vi "WorkingWithoutCheck-MatlabImageProcessing-red_tweezers_interface_linegen - test_edited for seq order - Copy - Copy - Copy.vi"() -> ()   [LabVIEW 2015]
doc: "This is the interface, the one VI which loads all the others. Run this one first.\n\n(the line below ensures settings are saved)\n[Red Tweezers Save Settings]"
uses:
  subvis/line_trapping.ctl
  subvis/spot.ctl
  <vilib>/userdefined/High Color/IMAQdx.ctl
  subvis/selection_element.ctl
  subvis/mouse_info.ctl
  <vilib>/Analysis/baseanly.llb/Real A x B.vi
  subvis/red_tweezers_globals_INTERNAL_VOLATILE.vi
  subvis/red_tweezers_globals.vi
  <vilib>/Analysis/NI_AALBase.lvlib
  <vilib>/vision/driver/NI_Vision_Acquisition_Software.lvlib
panel:
  out "Spot Storage":T1[](array[typedef]) {"Amplitude Correction" step=0.1; "Line Trapping"."Phase Gradient" step=0.05; "Line Trapping"."Vector"."x" step=1e-06 format="%#_6p"; "Line Trapping"."Vector"."y" step=1e-06 format="%#_6p"; "Line Trapping"."Vector"."z" step=1e-06 format="%#_6p"; "NA Position"."r" step=1e-06; "NA Position"."y" step=1e-06; "NA Position"."x" step=1e-06; "Position"."z" step=1e-06; "Position"."y" step=1e-06; "Position"."x" step=1e-06; "Phase" step=0.7753; "Intensity" step=0.1}
  out "# selected":i16
  out "Last Pattern":T1[](array[typedef]) {"Amplitude Correction" step=0.1; "Line Trapping"."Phase Gradient" step=0.05; "Line Trapping"."Vector"."x" step=1e-06 format="%#_6p"; "Line Trapping"."Vector"."y" step=1e-06 format="%#_6p"; "Line Trapping"."Vector"."z" step=1e-06 format="%#_6p"; "NA Position"."r" step=1e-06; "NA Position"."y" step=1e-06; "NA Position"."x" step=1e-06; "Position"."z" step=1e-06; "Position"."y" step=1e-06; "Position"."x" step=1e-06; "Phase" step=0.7753; "Intensity" step=0.1}
  out "Plugins":T3(array[cluster])=[{"Name"="ASI Stage", "Folder"=path "C:/Users/Richard Bowman/Dropbox/red_tweezers_1_4_rc4/plugins/ASI Stage.llb", "vi reference"=refnum, "Needs to be run"=TRUE, "Error"={"status"=FALSE, "code"=0, "source"=""}}, {"Name"="iTweezers", "Folder"=path "C:/Users/Richard Bowman/Dropbox/red_tweezers_1_4_rc4/plugins/iTweezers.llb", "vi reference"=refnum, "Needs to be run"=TRUE, "Error"={"status"=FALSE, "code"=0, "source"=""}}, {"Name"="MightexLED", "Folder"=path "C:/Users/Richard Bowman/Dropbox/red_tweezers_1_4_rc4/plugins/MightexLED.llb", "vi reference"=refnum, "Needs to be run"=TRUE, "Error"={"status"=FALSE, "code"=0, "source"=""}}]
  in  "Tab":T4(tab)
  out "Play Pressed":bool
  out "Y":dbl
  out "X":dbl
  in  "O Button":bool
  in  "OK Button":bool
  in  "Bubble Size":dbl=50.0002
  out "Hit Indicator":bool
  in  "On":bool
  out "Induce check":bool
  out "Area+ Buffer":dbl
  in  "Area to check":dbl=0.00025
  out "Prev Current Spot":dbl
  out "spots selected 2":i32=4
  out "Spot # Check":dbl
  out "Orig Y SC":dbl
  out "Orig X SC":dbl
  out "ID num check":dbl
  out "Value Check":dbl
  out "ID":dbl[](array[numeric])
  out "Null array":dbl[](array[numeric])
  out "Potential Collisions":dbl
  out "What to Check":dbl[](array[numeric])
  out "Num":dbl
  out "Old Y":dbl
  out "Old X":dbl
  out "init":dbl
  out "Looper":bool
  in  "Output to SLM":bool
  out "Maximum":dbl
  out "Projected Distance":dbl
  out "Previous Distance":dbl
  out "Group ID #":dbl
  in  "Buffer Zone":dbl=7e-05
  out "# of Spots":dbl
  out "Distance":dbl
  out "Hit":bool
  out "Y Displacement":dbl
  out "X Displacement":dbl
  out "Current Spot #":dbl
  out "spots selected":i32=4
  in  "lock aspect ratio":bool=TRUE
  in  "Size":cluster{"x":dbl, "y":dbl, "z":dbl} {"z" step=1e-06 format="%#_4p"; "y" step=1e-06 format="%#_4p"; "x" step=1e-06 format="%#_4p"}
  in  "Position":cluster{"x":dbl, "y":dbl, "z":dbl}={"x"=1e-06, "y"=-6.3e-06, "z"=0.0} {"z" step=1e-06 format="%#_4p"; "y" step=1e-06 format="%#_4p"; "x" step=1e-06 format="%#_4p"}
  in  "phase":dbl step=0.7753
  in  "Vortex Charge":i8
  in  "Intensity":dbl=1.0 step=0.1
  in  "add to selection":bool
  in  "random position":bool
  in  "new spot":bool
  in  "delete":bool
  in  "rotate":bool
  in  "Rotation Axis":u16(ring)=2 items=["Z", "X", "Y", "Custom"]
  in  "Angle (degrees)":dbl=2.0
  in  "Custom Axis":cluster{dbl, dbl, dbl}
  in  "Spot Shape":enum32{"Normal", "Line", "NA", "Mixed"}(tab)=enum."Mixed"
  in  "Line Trapping":T2 {"Phase Gradient" step=0.05; "Vector"."x" step=1e-06 format="%#_4p"; "Vector"."y" step=1e-06 format="%#_4p"; "Vector"."z" step=1e-06 format="%#_4p"}
  in  "Scale back aperture":dbl=1.1 step=0.1
  in  "Scale BA":bool
  in  "Position on back aperture":cluster{"x":dbl, "y":dbl}={"x"=-5.84327907697451e-18, "y"=0.0} {"y" step=0.1 format="%#_4p"; "x" step=0.1 format="%#_4p"}
  in  "Radius on back aperture":dbl=1.1 step=0.1
  in  "Generate":bool
  in  "Pattern":T5(tab)
  in  "Spots across centre":i32=5
  in  "Reference Array?":bool
  in  "Fraction of SLM":dbl=1.0
  in  "Spots across centre":i32=5
  in  "N":cluster{i32, i32}
  in  "spacing/m":dbl=2.0
  in  "Iterations":i32=10
  out "non-uniformity":dbl(slide)=0.031119223416512406 scale=0.0..0.2
  out "efficiency":dbl(slide)=0.8985936267644501 scale=0.0..1.0
  in  "Optimise":bool
  in  "Reset Phase/Amplitude":bool
  in  "Fall-off/m":dbl=0.00025 min=0.0 step=1e-06 format="%#_4p"
  in  "Abort Plugin":bool
  in  "Plugin:":u16(ring)=1 items=["ASI Stage", "iTweezers", "MightexLED"]
  in  "Save Video":bool
  in  "Global ROI (requires restart)":i32[](array[numeric])=[0, 0, 1280, 512]
  in  "Zoom":bool
  in  "Draw ROI":bool
  in  "Zoom to Fit":bool
  out "Image Information":string="640x480 1.93X 8-bit image 255    (0,0)"
  in  "Camera":T6
  in  "Time per Frame (ms)":dbl
  in  "Edit Sequence Mode":bool
  in  "Manual Edit":bool
  in  "Bubble ID to Empty":dbl
  in  "Clearance Button":bool
  in  "Manual Sequence":bool
  in  "Play Sequence":bool
  in  "Reset":bool
  out "Sequence Instances":dbl
  out "Counter":dbl
  in  "Save State":bool
  out "Sequence On?":bool
  in  "Sequence Order":dbl
  out "Selection/Group":T7[](array[typedef])
  in  "Sequence Storer":T1[][](array[typedef]) {"Amplitude Correction" step=0.1; "Line Trapping"."Phase Gradient" step=0.05; "Line Trapping"."Vector"."x" step=1e-06 format="%#_6p"; "Line Trapping"."Vector"."y" step=1e-06 format="%#_6p"; "Line Trapping"."Vector"."z" step=1e-06 format="%#_6p"; "NA Position"."r" step=1e-06; "NA Position"."y" step=1e-06; "NA Position"."x" step=1e-06; "Position"."z" step=1e-06; "Position"."y" step=1e-06; "Position"."x" step=1e-06; "Phase" step=0.7753; "Intensity" step=0.1}
  out "Time Elapsed(ms)":i32
  out "Start":i32
  out "Stop":i32
  out "Insert End":bool
  out "NewXYRates":dbl[][](array[numeric])
  out "NewXYArraySize":dbl
  out "NewXYArray":dbl[][](array[numeric])
  out "Rates":dbl
  out "LCS Y":dbl
  out "LCS X":dbl
  out "LCS":dbl
  in  "Play":bool
  out "Initiate Creation 2":dbl
  out "Max Number of Bubbles 2":dbl
  out "Number of Planned Sequence Frames 2":dbl
  in  "Add Additional Frames":bool
  in  "Frame Location":dbl
  in  "Additional Frames Wanted":dbl
  in  "Tab Control":enum32{"Line", "Arc"}(tab)
  out "X Rate":dbl
  out "Y Rate":dbl
  out "Degree Rate":dbl
  out "Radians":dbl
  out "Center Y":dbl
  out "Center X":dbl
  in  "Radius X":dbl
  in  "Theta":dbl
  in  "Lock Current Spot":bool
  out "Locked Current Spot":dbl
  out "Numeric":dbl
  out "probe":dbl
  in  "Insert":bool
  in  "Start at Which Frame?":dbl
  out "Original Y":dbl
  out "Original X":dbl
  in  "Mark Original Position":bool
  in  "How Many Frames?":dbl
  out "New Y":dbl
  out "New X":dbl
  out "Spot Storage 2":T1[](array[typedef]) {"Amplitude Correction" step=0.1; "Line Trapping"."Phase Gradient" step=0.05; "Line Trapping"."Vector"."x" step=1e-06 format="%#_6p"; "Line Trapping"."Vector"."y" step=1e-06 format="%#_6p"; "Line Trapping"."Vector"."z" step=1e-06 format="%#_6p"; "NA Position"."r" step=1e-06; "NA Position"."y" step=1e-06; "NA Position"."x" step=1e-06; "Position"."z" step=1e-06; "Position"."y" step=1e-06; "Position"."x" step=1e-06; "Phase" step=0.7753; "Intensity" step=0.1}
  in  "Save":bool
  in  "Load":bool
  out "Video Frame Rate":dbl(knob)=50.00000000000003 scale=0.0..100.0 scale format="%.1f"
  out "Interface Frame Rate":dbl(knob)=97.23240312927678 scale=0.0..100.0 scale format="%.1f"
  in  "stop":bool=TRUE
  out "error out":errorcluster
  out "MOP pressed":bool
  out "MOP pressed After":bool
  out "X Pos every 10 sec":dbl
  out "Elapsed Time":dbl
  out "Position Indicator":string
  out "Spot Checker":T1[](array[typedef]) {"Amplitude Correction" step=0.1; "Line Trapping"."Phase Gradient" step=0.05; "Line Trapping"."Vector"."x" step=1e-06 format="%#_6p"; "Line Trapping"."Vector"."y" step=1e-06 format="%#_6p"; "Line Trapping"."Vector"."z" step=1e-06 format="%#_6p"; "NA Position"."r" step=1e-06; "NA Position"."y" step=1e-06; "NA Position"."x" step=1e-06; "Position"."z" step=1e-06; "Position"."y" step=1e-06; "Position"."x" step=1e-06; "Phase" step=0.7753; "Intensity" step=0.1}
  out "Image":T8(plugin-control)
  # "Notes:\n\nIf you are doing non-sequence controls,\nthe delete function can be used as intended.\nHowever, do not use the delete function after\nrunning a sequence! Using it will prevent\nthe bubbles from appearing as the\nnumber of spots will change, which is\nessential for the sequence to work (it would\nbe displaying the maximum number of\nbubbles). \n\nIf you happen to delete a bubble, it can be \nrestored by inserting a new spot. Once enough\nspots have been restored, click on manual edit\nto correct the # of spots tracker. It should \nbe restored to where it originally was."
  # "The SLM can be used to shape spots; here you can restrict the NA of a spot (so it comes only from part of the back aperture), or create a line-trap"
  # "The traps do not have any spot-shaping applied (so they should just be diffraction-limited focal spots)."
  # "This shapes the amplitude (and phase) of the beam to create extended line traps.  The \"Phase Gradient\" control allows the Poynting vector to push things along the line.  Unfortunately, some work is needed on the scaling factors so the phase gradient control will need tweaking if the line trap has a nonzero z component."
  # "By default,each spot comes from the whole back aperture.  Here, you can limit a spot to come from a specific part of the back aperture."
  # "The control below allows you to scale the whole back aperture (i.e. the position and size of all the apertures).  It's a one-time operation, i.e. only changes things when you push \"ok\"."
  # "A Combination of line-trapping and NA restriction has been applied to these traps.  You can get at the line trap or NA parameters on the other tabs, switching to the NA tab does not delete the line-trap settings."
  # "This tab generates Shack-Hartmann type holograms, which are often useful when aligning the system, and arrays of spots."
  # "The controls above only work when using the \"IMAQdx with ROI Buttons\" case in the bottom loop.  You can save video regardless of camera code though."
  # "Manual Edit allows a user to\ngo to a specific sequence frame."
  # "To clear the sequence, you must\nclear the array. Right click on sequence\nstorer to do this."
  # "Use this to \"clear\" a \nspecific bubble. If\nworking on a sequence,\nuse this as your delete\nbutton! You can update\nthe view by using manual edit."
  # "Use the reset button\nto clear counter.\nIt becomes necessary\nwhen you clear the array,\nespecially in manual mode."
  # "Use the sequence creator tab to specify the\nnumber of bubbles you want along with\nthe number of frames.\n\nTo save at a specific interval, the sequence\norder can be used to place the state. If used\nto correct something, it will replace the\nentire sequence frame.\n\n\"Sequence On?\" is only used in auto mode."
  # "Multiple bubbles can  be done with the\nline function. One bubble at a time for the arc\nfunction."
  # "Using the Load/Save function:\n\nRed Tweezers itself is unable to save long \nsequences, but a separate program is able to\naccomplish this. To do this, follow these\nsteps:\n\n1. After creating your sequence, press the save\nbutton below.\n\n2. Then, go to the subvi folder and find\nSequenceSaver.vi.\n\n3. At the control \"Sequence Storer,\" right-click\nthe dimensions part of the array and go to\ndata operations.\n\n4. Press \"Make Current Values Default\" and save\nthe sequence.\n\n5. The next time you load the program, simply\npress load to re-acquire the sequence. You\nwill need to insert the bubbles again, but after\nthe first frame can be recovered by using\nSequenceControl.vi."
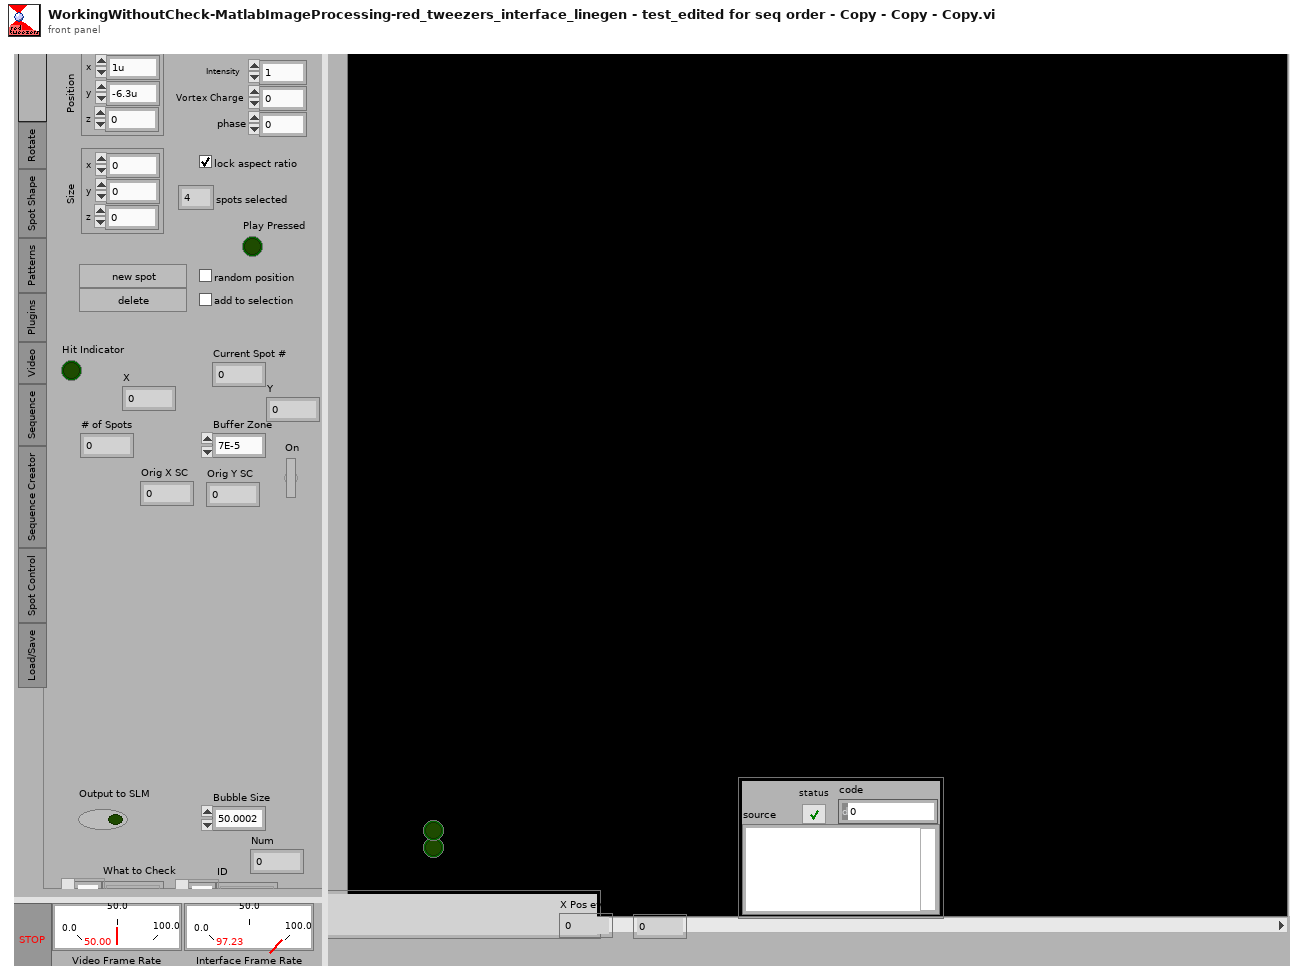
[diagram p1: front panel]
types:
  T1 = typedef "spot.ctl" = cluster{"Position":cluster{"x":dbl, "y":dbl, "z":dbl}, "Intensity":dbl, "Vortex Charge":i8, "Phase":dbl, "NA Position":cluster{"x":dbl, "y":dbl, "r":dbl}, "Line Trapping":T2, "Amplitude Correction":dbl}
  T2 = typedef "line_trapping.ctl" = cluster{"Vector":cluster{"x":dbl, "y":dbl, "z":dbl}, "Phase Gradient":dbl}
  T3 = cluster{"Name":string, "Folder":path, "vi reference":refnum<vi>, "Needs to be run":bool, "Error":errorcluster}[]
  T4 = enum32{"Current Spot", "Rotate", "Spot Shape", "Patterns", "Plugins", "Video", "Sequence", "Sequence Creator", "Spot Control", "Load/Save"}
  T5 = enum32{"HCP Shack-Hartmann", "Square Shack-Hartmann", "Rectangular Grid"}
  T6 = typedef "IMAQdx.ctl" = refnum<k21>
  T7 = typedef "selection_element.ctl" = cluster{"Group ID":i32, "Selected":bool}
  T8 = typedef "IMAQ Image.ctl" = refnum<image>
  T9 = typedef "mouse_info.ctl" = cluster{"Button Down":bool, "Dragging":bool, "Position (Image Pixels)":cluster{"X":dbl, "Y":dbl}, "Previous Position (Image Pixels)":cluster{"X":dbl, "Y":dbl}, "Button":u16, "Mods":cluster{"Double Click":bool, "Menu Key":bool}, "PlatMods":cluster{"Shift":bool, "Ctrl":bool, "Alt":bool, "Cmd":bool, "Opt":bool}}
  T10 = cluster{"Position":cluster{"x":dbl, "y":dbl, "z":dbl}, "Intensity":dbl, "Vortex Charge":i8, "Phase":dbl, "NA Position":cluster{"x":dbl, "y":dbl, "r":dbl}, "Line Trapping":T2, "Amplitude Correction":dbl}
  T11 = enum16{"Set guide visibility", "Set grid visibility", "Show front panel", "Render on image"}
  T12 = enum32{"Current Spot", "Rotate", "Spot Shape", "Patterns", "Plugins", "Video"}
  T13 = enum16{"Left Button", "Center Button", "Right Button", "Window Close"}
  T14 = cluster{"number: 0 to 1":dbl, "number: 0 to 1":dbl}
  T15 = typedef "NI_Matrix.lvlib/RealMatrix.ctl" = dbl[][]
  T16 = typedef "overlay_element.ctl" = cluster{"Tool":enum16{"Lines", "Oval", "Rectangle", "Text"}, "Points":cluster{"X":dbl, "Y":dbl}[], "Drawing Mode":u32, "Color":u32, "String":string}
  T17 = enum32{"Current Spot", "Rotate", "Spot Shape", "Patterns", "Plugins", "Video", "Particle Tracking", "Clamping", "Blank"}[]
  T18 = typedef "LVMenuShortCut.ctl" = cluster{"include Shift key?":bool, "include Ctrl key?":bool, "shortcut key":string}
  T19 = typedef "LVPoint32TypeDef.ctl" = cluster{"Horizontal":i32, "Vertical":i32}
  T20 = cluster{"Shift":bool, "Ctrl":bool, "Alt":bool, "Cmd":bool, "Opt":bool}
  T21 = cluster{"Button Down":bool, "Dragging":bool, "Mouse Coords (image pixels)":cluster{dbl, dbl}, "Mouse Coords (image pixels)":cluster{dbl, dbl}, "Button":u16, "Mods":cluster{"Double Click":bool, "Menu Key":bool}, "PlatMods":cluster{"Shift":bool, "Ctrl":bool, "Alt":bool, "Cmd":bool, "Opt":bool}}
  T22 = cluster{"NewXYArray[0]":dbl, "NewXYArray[1]":dbl, "NewXYArray[2]":dbl, "NewXYArray[3]":dbl, "NewXYArray[4]":dbl, "NewXYArray[5]":dbl, "NewXYArray[6]":dbl, "NewXYArray[7]":dbl, "NewXYArray[8]":dbl}
  T23 = cluster{"Average Frame Time":dbl, "millisecond timer value":u32}
  T24 = cluster{"Position":cluster{"x":dbl, "y":dbl, "z":dbl}, "Intensity":dbl, "Vortex Charge":i8, "Phase":dbl, "NA Position":cluster{"x":dbl, "y":dbl, "r":dbl}, "Line Trapping":T2, "Amplitude Correction":dbl}[]
  T25 = enum32{"Bad", "Idle", "Run top level", "Running"}
  T26 = typedef "Image Type" = u32
  T27 = typedef "AviRefnum.ctl" = refnum<k1>
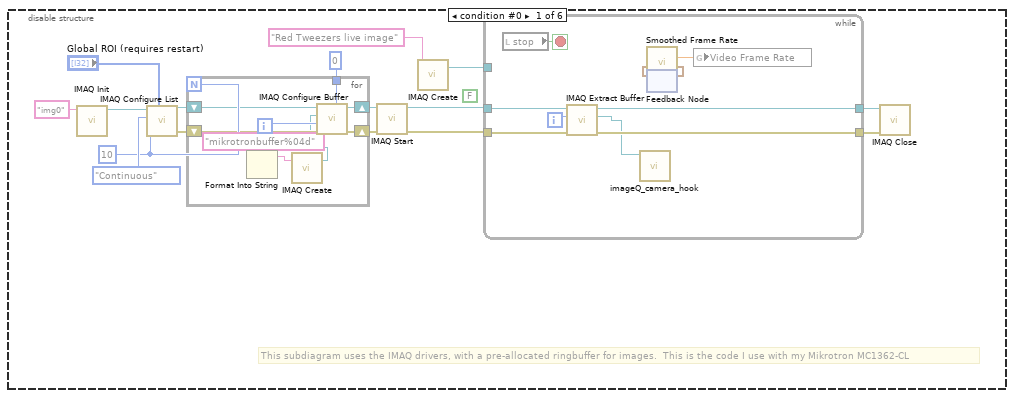
[diagram p3: hidden frame]
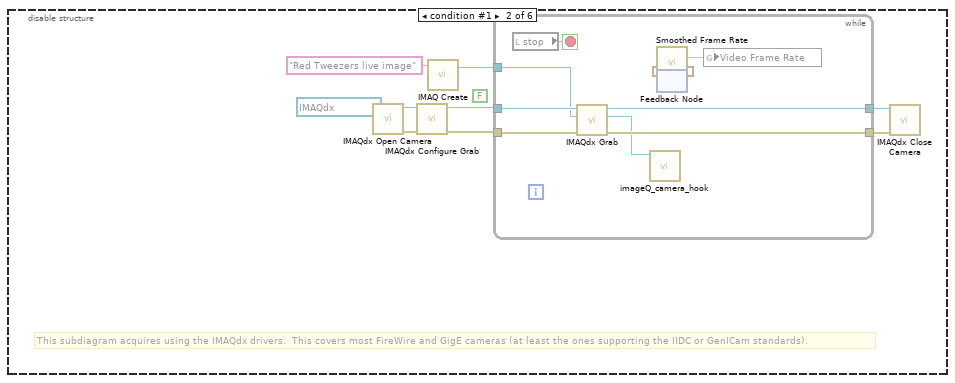
[diagram p4: hidden frame]
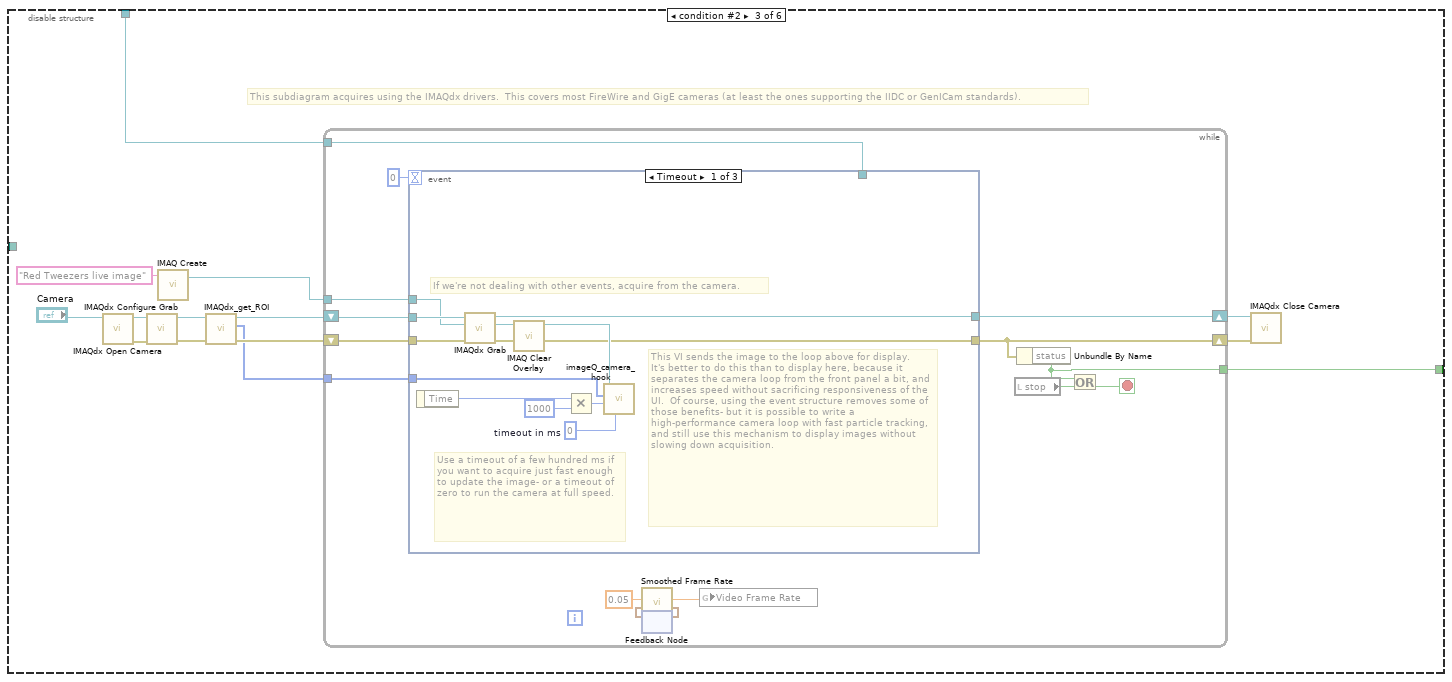
[diagram p5: hidden frame]
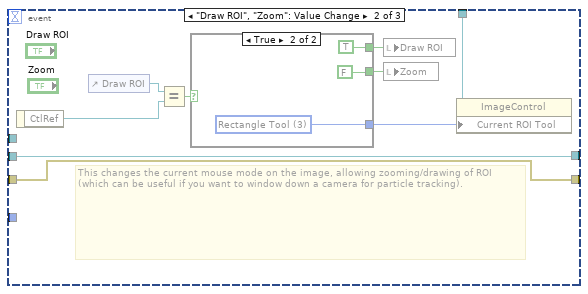
[diagram p6: hidden frame]
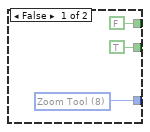
[diagram p7: hidden frame]
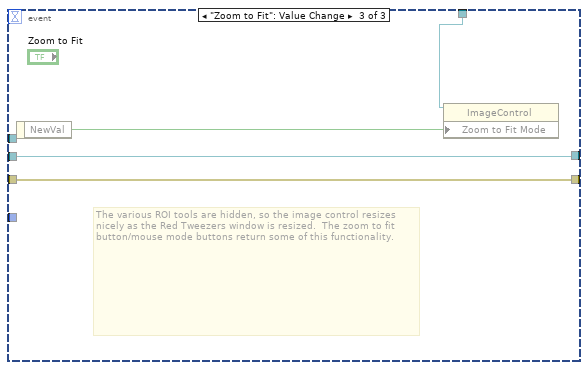
[diagram p8: hidden frame]
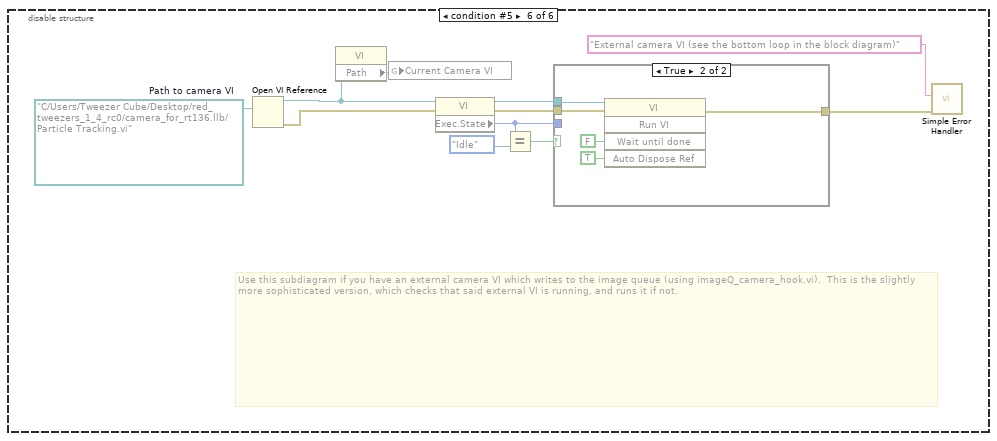
[diagram p10: hidden frame]
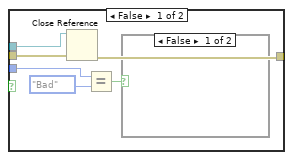
[diagram p11: hidden frame]
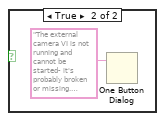
[diagram p12: hidden frame]
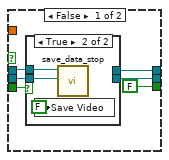
[diagram p13: hidden frame]
diagram:
  w11 = "red_tweezers_display_imageQ" ("Queue Name")
  w23 = T9 {"Button Down"=FALSE, "Dragging"=FALSE, "Position (Image Pixels)"={"X"=0.0, "Y"=0.0}, "Previous Position (Image Pixels)"={"X"=0.0, "Y"=0.0}, "Button"=0, "Mods"={"Double Click"=FALSE, "Menu Key"=FALSE}, "PlatMods"={"Shift"=FALSE, "Ctrl"=FALSE, "Alt"=FALSE, "Cmd"=FALSE, "Opt"=FALSE}}  # Mouse Information
  w24 = refnum<vi> refnum  # Image
  # "The funny looking feedback-node structure is deliberate (if odd).  We want to reload settings from the last used file (stored in the registry) only if this program has not been run since it was last loaded from file/recompiled.  That's why I use an uninitialised shift register: every time the program runs, it increments.  So, if it is zero, this is our first run (or we've been recently recompiled)."
  # "This loop handles the video that is displayed on-screen and saved to file."
  # "Initially, we only register to be told when the user clicks the image"
  # "This is the actual image control"
  # "This is a generic reference.\nIt is just a placeholder, so we can register for events later."
  # "This version of red tweezers uses two coordinate systems: \n1. Real Coordinates - corresponding to physical distances in 3D in microns\n2. Image Coordinates - position on the camera image, relative to the top left of the CURRENT ROI, measured in pixels. If the ROI changes, the relationship between \"real units\" and \"image pixels\" may change, so all values should be stored and presented to the user in REAL units unless there is a good reason to do otherwise."
  n1 = control-ref of="Plugin Pnl"() -> (w20:refnum<vi>)
  n2 = flat-sequence {
    tunnel: [w27] -> w6
    tunnel: w4 -> [_]
    frame #0 {
      n3 = vi-ref "red_tweezers_globals_INTERNAL.vi"() -> (w28:refnum<vi>)
      n4 = property class="VI"(reference=w28) -> ("Path"=w27:path)  [unwired: 1 in, 2 out]
      n5 = global write "red_tweezers_globals_INTERNAL_VOLATILE.vi" "Current Camera VI"(w27) -> ()
    }
  }
  n6 = control-ref of="Plugin:"() -> (w21:refnum<vi>)
  n7 = feedback #1() -> (w14:dbl)  [unwired: 1 in]
  n8 = Equal To 0?(x=w14) -> (x = 0?=w13:bool)
  n9 = Increment(x=w14) -> (x+1=w12:dbl)
  n10 = feedback-in #1(w12) -> ()
  n11 = call "plugins_load.vi"("Sub Panel"=w20, "Plugin Chooser"=w21) -> ("error out"=w15:errorcluster, "Plugins"=w17:T3)  [unwired: 2 in, 2 out]
  "Plugins" <- w17
  n12 = control-ref of="Image"() -> (w5:refnum<vi>)
  n13 = case shown="True" w13 {
    tunnel: w15 -> [_ w29]
    tunnel: [_ w29] -> w4
    frame False {
    }
    frame True {
      n14 = call "settings_load_default_file.vi"("error out"=w29) -> ()
    }
  }
  n15 = flat-sequence {
    tunnel: w4 -> [_]
    tunnel: w2 -> [w31]
    frame #0 {
      # "ensure we don't accidentally start saving video, and run UDP Sender to set up the hologram window."
      n16 = local write "Save Video"(FALSE ("background subtraction")) -> ()
      n17 = call "UDP Sender generic_2.vi"("Spots"=w31) -> ()  [unwired: 2 in, 1 out]
    }
  }
  n18 = global read "red_tweezers_globals.vi" "Selection/Group"() -> (w22:T7[])
  n19 = register-events(w5, w24, w24, w24) -> (reference out=w25:refnum<event-registration>)  [unwired: 2 in, 1 out]
  n20 = global read "red_tweezers_globals.vi" "Spots"() -> (w2:T1[])
  n21 = local write "stop"(FALSE ("STOP")) -> ()
  n22 = call "ensure_selection_matches_spots.vi"("Selection and Groups in"=w22, "Spots"=w2) -> ("Selection and Groups out"=w26:T7[], "Spots (duplicate)"=w1:T1[])  [unwired: 4 in]
  n23 = call "IMAQ Create"("Image Name"=w11) -> ("New Image"=w9:T8)  [unwired: 4 in, 1 out]
  n24 = call "imageQ_create_return_queue.vi"("Queue Name"=w11) -> ("queue out"=w10:refnum<queue>)
  n25 = while {
    shift-right: [w110] -> _
    shift-left: w1 -> [w130]
    shift-right: [w129] -> _
    shift-left: w26 -> [w128]
    shift-right: [w132] -> _
    shift-left: _ -> [w123]
    shift-right: [w131] -> _
    shift-left: _ -> [w122]
    tunnel: w5 -> [w127]
    shift-right: [w121] -> _
    shift-left: w23 -> [w120]
    shift-right: [w124] -> _
    shift-left: w25 -> [w125]
    border: errorcluster {"status"=FALSE, "code"=0, "source"=""} ("error out") -> [_]
    tunnel: [errorcluster {"status"=FALSE, "code"=0, "source"=""} ("error in (no error)")] -> w18
    border: w17 -> [_]
    tunnel: w1 -> [w111]
    stop <- w112 stop-if-true
    # "This Play Function inserts bubbles from a given .mat file into the sequence storer"
    # "The function inserts the newly generated sequence for the automatic sequence generator. It also contains the code\nthe code necessary to check whether the bubbles will intersect with each other in the sequence."
    # "This calculates the size of the area including the buffer zone length.\nThe bubble diameter will also be included in the near future."
    # "The statement to the right controls the area that are being chcecked and checks\nwhich bubbles need to be checked.  There are two instances where this activates\nin this case:\n\nWhen a new bubble is selected\nWhen a bubble is deselected, reverting to the last current spot #\n\nThe other case, when the bubble moves out of the area specified, is located\ninside the while loop controlling the bubble movement with a mouse."
    # "Timer function example"
    # "These functions help with the calculations for the sequence generator."
    # "This loads the sequence from the \"saver\" VI. The save function below \"saves\" the sequence into the saver VI."
    # "The VI above is SequenceSaver.vi which contains the\ncode necessary to create a sequence."
    # "This case structure is the Save State structure. This stores\nthe current state of the bubbles (ie position)."
    # "Reset sets the counter back to zero. This is particularly useful \nwhen using the manual sequence."
    # "This case structure helps to continue the sequence.\nThis takes the true case of the Sequence On? function\nor the true case for the Manual Sequence function\nin order to go to the next sequence frame."
    # "This case structure allows for the playing of the sequence.\nThe amount of time it takes to go through the sequence\ncan be edited on the current spot menu."
    # "We only write to the image overlay when we are in one of the tabs, to prevent it disappearing when we are (for example) using the mouse."
    # "These wires control saving undo info. See the VI below's tip strips for details."
    # "Setting these wires to false means:\n(1) dragging moves the selection\n(2) clicking spots changes selection\nset them to true to stop the default mouse behaviour, don't wire them straight through!"
    n26 = event shown="[0] Timeout" {
      selector: w125 -> [w440 w1111 w1116 w1338 w1366 w1383 w1480 _]
      dyn-events: [w440 w1110 w1116 w1336 w1363 w1384 w1480 _] -> w124
      timeout: 0 -> [_ _ _ _ _ _ _ _]
      tunnel: [w448 _ w1118 w1333 w1368 w1375 w1467 _] -> w132
      tunnel: [w447 _ w1117 w1332 w1367 w1374 w1471 _] -> w131
      tunnel: [w446 _ _ _ _ _ _ _] -> w83
      tunnel: w130 -> [w445 w1106 w1123 w1328 w1361 w1380 w1475 w1798]
      tunnel: [w444 w1106 w1121 w1328 w1361 w1371 w1473 w1798] -> w118
      tunnel: [w443 w1105 w1120 w1317 w1360 w1381 w1463 w1797] -> w117
      tunnel: w128 -> [w442 w1105 w1122 w1317 w1360 w1379 w1474 w1797]
      tunnel: w127 -> [w441 w1107 w1113 w1327 w1364 w1382 w1476 _]
      tunnel: [w439 _ w1115 w1337 T9 {"Button Down"=FALSE, "Dragging"=FALSE, "Position (Image Pixels)"={"X"=0.0, "Y"=0.0}, "Previous Position (Image Pixels)"={"X"=0.0, "Y"=0.0}, "Button"=0, "Mods"={"Double Click"=FALSE, "Menu Key"=FALSE}, "PlatMods"={"Shift"=FALSE, "Ctrl"=FALSE, "Alt"=FALSE, "Cmd"=FALSE, "Opt"=FALSE}} T9 {"Button Down"=FALSE, "Dragging"=FALSE, "Position (Image Pixels)"={"X"=0.0, "Y"=0.0}, "Previous Position (Image Pixels)"={"X"=0.0, "Y"=0.0}, "Button"=0, "Mods"={"Double Click"=FALSE, "Menu Key"=FALSE}, "PlatMods"={"Shift"=FALSE, "Ctrl"=FALSE, "Alt"=FALSE, "Cmd"=FALSE, "Opt"=FALSE}} w1479 _] -> w121
      tunnel: w120 -> [w439 _ w1115 _ _ w1378 w1470 _]
      tunnel: w123 -> [_ _ w1118 w1333 w1368 w1375 w1467 _]
      tunnel: w122 -> [_ _ w1117 w1332 w1367 w1374 w1471 _]
      tunnel: [w438 _ _ _ _ _ _ _] -> w119
      tunnel: [_ _ w1114 _ _ _ TRUE _] -> w116
      tunnel: [_ _ _ TRUE TRUE TRUE FALSE _] -> w115
      tunnel: [TRUE _ _ _ _ _ _ _] -> w113
      tunnel: [_ _ _ _ _ _ _ "stop"] -> w112
      tunnel: w111 -> [_ _ _ _ _ _ w1464 _]
      event Timeout {
        n27 = event-data() -> ()  [unwired: 1 in, 1 out]
        n28 = case shown="\"Current Spot\", Default" "Tab" {
          tunnel: [w463 w731 w878 w980 w1061 w1099] -> w444
          tunnel: w445 -> [w460 w733 w879 w982 w1061 w1099]
          tunnel: w442 -> [w449 w732 w876 w981 w1060 w1098]
          tunnel: [w462 w730 w877 w979 w1060 w1098] -> w443
          tunnel: [w450 _ TRUE _ _ _] -> w448
          tunnel: [w450 _ _ _ _ _] -> w447
          tunnel: [_ _ _ FALSE _ _] -> w446
          tunnel: w441 -> [_ _ _ _ _ w1095]
          tunnel: w439 -> [_ _ w858 _ _ _]
          tunnel: [_ _ w860 _ _ _] -> w438
          frame "Current Spot", Default {
            w450 = FALSE
            # "The function below contains the code necessary to use the automatic sequence generator to create specific movements. It also helps translate cases where the point is entered in not dragged.\nThis prevents bubbles from intersecting if the bubble is told not to intersect."
            # "If it's out of date, update front panel"
            n29 = call "find_centroid.vi"("Selection and Groups"=w449, "Spots"=w460) -> ("Mean Values"=w458:T1, "size"=w452:cluster{"x":dbl, "y":dbl, "z":dbl}, "centroid"=w453:cluster{"x":dbl, "y":dbl, "z":dbl}, "# selected"=w451:i16)  [unwired: 2 in, 1 out]
            n30 = stacked-sequence {
              tunnel: w451 -> [_ w465]
              frame #0 {
                n31 = local read "spots selected"() -> (→"spots selected 2":i32)
              }
              frame #1 {
                "spots selected" <- w465
              }
            }
            n32 = feedback-in #2(w458) -> ()
            n33 = feedback #2() -> (w459:T1)  [unwired: 1 in]
            n34 = feedback #3() -> (w457:cluster{"x":dbl, "y":dbl, "z":dbl})  [unwired: 1 in]
            n35 = feedback-in #3(w452) -> ()
            n36 = Not Equal?(x=w459, y=w458) -> (x != y?=w456:bool)
            n37 = Not Equal?(x=w457, y=w452) -> (x != y?=w455:bool)
            n38 = Or(x=w456, y=w455) -> (x .or. y?=w454:bool)
            n39 = case shown="True" w454 {
              tunnel: w458 -> [_ w471]
              tunnel: w452 -> [_ w467]
              frame False {
              }
              frame True {
                n40 = Unbundle By Name(w471) -> ("Position"=w466:cluster{"x":dbl, "y":dbl, "z":dbl}, "Intensity"=w469:dbl, "Vortex Charge"=w468:i8, "Phase"=w470:dbl)
                n41 = local write "Size"(w467) -> ()
                n42 = local write "Vortex Charge"(w468) -> ()
                n43 = local write "Intensity"(w469) -> ()
                n44 = local write "Position"(w466) -> ()
                n45 = local write "phase"(w470) -> ()
                n46 = Unbundle By Name(w466) -> ()  [unwired: 2 out]
              }
            }
            n47 = local write "Selection/Group"(w449) -> ()
            n48 = event shown="[0] Timeout" {
              selector: _ -> [_ _ _ _ _ _ _ _]
              dyn-events: _ -> [_ _ _ _ _ _ _ _]
              timeout: 10 -> [_ _ _ _ _ _ _ _]
              tunnel: w460 -> [w473 w477 w491 w514 w618 w663 w689 w712]
              tunnel: w449 -> [w472 w476 w494 w521 w605 w660 w686 w710]
              tunnel: [w473 w475 w492 w513 w606 w661 w687 w711] -> w463
              tunnel: [w472 w474 w493 w521 w605 w660 w686 w710] -> w462
              tunnel: w453 -> [_ _ _ _ w617 _ _ _]
              event Timeout {
                n49 = event-data() -> ()  [unwired: 3 out]
              }
              event "delete": Value Change {
                n50 = event-data() -> ()  [unwired: 7 out]
                n51 = call "delete_selected_spots.vi"("Selection/Group 3"=w476, "Spots 3"=w477) -> ("Selection/Group 2"=w474:T7[], "Spots 2"=w475:T1[])  [unwired: 4 in]
              }
              event "new spot": Value Change {
                # "If we're not adding it to the selection, de-select all the other spots"
                n52 = event-data() -> ()  [unwired: 7 out]
                n53 = call "coords_ROI_currentimage.vi"() -> ("Mono ROI"=w478:i32[])
                n54 = case shown="False" "add to selection" {
                  tunnel: w494 -> [w507 w512]
                  tunnel: [w506 w512] -> w489
                  frame False {
                    n55 = for {
                      tunnel: w507 -> [w510] mode=indexing
                      tunnel: [w511] -> w506 mode=indexing
                      n56 = Unbundle(w510) -> ("Group ID"=w509:i32)  [unwired: 1 out]
                      n57 = Bundle(cluster=w510, "Group ID"=w509, "Selected"=FALSE ("Label.Visible")) -> (w511:T7)
                    }
                  }
                  frame True {
                  }
                }
                n58 = Index Array(array=w478) -> (element #1=w484:i32, element #2=w485:i32, element #3=w483:i32, element #4=w482:i32)  [unwired: 4 in]
                n59 = Bundle("Numeric"=w484, "Numeric"=w485) -> (w479:cluster{"Numeric":i32, "Numeric":i32})  [unwired: 1 in]
                n60 = Bundle("Numeric"=w483, "Numeric"=w482) -> (w481:cluster{"Numeric":i32, "Numeric":i32})  [unwired: 1 in]
                n61 = Subtract(x=w481, y=w479) -> (x-y=w480:cluster{"Numeric":i32, "Numeric":i32})
                n62 = case shown="True" "random position" {
                  tunnel: [w496 w502] -> w487
                  tunnel: w480 -> [_ w498]
                  tunnel: w479 -> [_ w497]
                  frame False {
                    n63 = call "replace_position.vi"("Position"=cluster{"x":dbl, "y":dbl, "z":dbl} {"x"=0.0, "y"=0.0, "z"=0.0}) -> ("Spot"=w496:T1)  [unwired: 1 in, 2 out]
                  }
                  frame True {
                    n64 = Random Number (0-1)() -> (number: 0 to 1=w504:dbl)
                    n65 = Random Number (0-1)() -> (number: 0 to 1=w505:dbl)
                    n66 = Bundle("number: 0 to 1"=w505, "number: 0 to 1"=w504) -> (w503:T14)  [unwired: 1 out]
                    n67 = Multiply(x=w503, y=w498) -> (x*y=w500:cluster{dbl, dbl})
                    n68 = Add(x=w500, y=w497) -> (x+y=w499:cluster{dbl, dbl})
                    n69 = call "coords_image_to_real_currentimage.vi"("Position (pixels on image)"=w499) -> ("Position (real coords)"=w501:cluster{dbl, dbl, "Z":dbl})  [unwired: 9 in]
                    n70 = call "replace_position.vi"("Position"=w501) -> ("Spot"=w502:T1)  [unwired: 1 in, 2 out]
                  }
                }
                n71 = Build Array (concatenate)(w491, w487) -> (w492:T1[])
                n72 = Build Array (concatenate)(w489, cluster{i32, "Label.Visible":bool} {0, "Label.Visible"=TRUE}) -> (w493:T7[])
              }
              event "Position": Value Change {
                # "If the position has changed, translate the spots"
                n73 = event-data() -> ("OldVal"=w519:cluster{"x":dbl, "y":dbl, "z":dbl}, "NewVal"=w520:cluster{"x":dbl, "y":dbl, "z":dbl})  [unwired: 5 out]
                n74 = flat-sequence {
                  tunnel: w521 -> [w525]
                  tunnel: w518 -> [w524]
                  tunnel: w514 -> [w523]
                  tunnel: [w522] -> w515
                  frame #0 {
                    n75 = for {
                      tunnel: w523 -> [w530] mode=indexing
                      tunnel: w525 -> [w527] mode=indexing
                      tunnel: [w529] -> w522 mode=indexing
                      tunnel: w524 -> [w528]
                      n76 = Unbundle(w527) -> ("Selected"=w526:bool)  [unwired: 1 out]
                      n77 = case shown="True" w526 {
                        tunnel: w530 -> [w531 w536]
                        tunnel: [w531 w535] -> w529
                        tunnel: w528 -> [_ w532]
                        frame False {
                        }
                        frame True {
                          n78 = call "extract_position.vi"("Spot"=w536) -> ("Position"=w533:cluster{"x":dbl, "y":dbl, "z":dbl})
                          n79 = Add(x=w533, y=w532) -> (x+y=w534:cluster{"x":dbl, "y":dbl, "z":dbl})
                          n80 = call "replace_position.vi"("Position"=w534, "Spot in"=w536) -> ("Spot"=w535:T1)  [unwired: 2 out]
                        }
                      }
                    }
                  }
                }
                n81 = Subtract(x=w520, y=w519) -> (x-y=w518:cluster{"x":dbl, "y":dbl, "z":dbl})
                n82 = local read "# of Spots"() -> (w517:dbl)
                n83 = stacked-sequence {
                  tunnel: w514 -> [_ w541 _]
                  tunnel: w515 -> [_ w540 _]
                  tunnel: w517 -> [_ w539 _]
                  tunnel: [_ _ w588] -> w516
                  tunnel: w515 -> [_ _ w587]
                  tunnel: w514 -> [_ _ w586]
                  tunnel: [_ _ w585] -> w513
                  frame #0 {
                    n84 = local write "Looper"(FALSE) -> ()
                    "init" <- 0
                  }
                  frame #1 {
                    n85 = for {
                      N: w539 -> [_]
                      tunnel: w541 -> [w546]
                      tunnel: w540 -> [w551]
                      stop <- w552 stop-if-true
                      n86 = local read "init"() -> (w545:dbl)
                      n87 = Index Array(array=w551, index=w545) -> (element=w550:T1)
                      n88 = Index Array(array=w546, index=w545) -> (element=w544:T1)
                      n89 = Unbundle By Name(w550) -> ("Position.x"=w549:dbl, "Position.y"=w548:dbl)
                      n90 = local read "# of Spots"() -> (w547:dbl)
                      n91 = Unbundle By Name(w544) -> ("Position.x"=→"Old X":dbl, "Position.y"=→"Old Y":dbl)
                      n92 = local write "New X"(w549) -> ()
                      n93 = local write "New Y"(w548) -> ()
                      n94 = stacked-sequence {
                        tunnel: w546 -> [w557 _]
                        tunnel: w549 -> [w556 _]
                        tunnel: w548 -> [w555 _]
                        tunnel: w547 -> [w554 _]
                        tunnel: w545 -> [w553 _]
                        frame #0 {
                          n95 = for {
                            N: w554 -> [_]
                            tunnel: w557 -> [w579]
                            tunnel: w556 -> [w578]
                            tunnel: w555 -> [w576]
                            tunnel: w553 -> [w561]
                            i -> [w563]
                            stop <- w562 stop-if-true
                            n96 = Index Array(array=w579, index=w563) -> (element=w580:T1)
                            n97 = Unbundle By Name(w580) -> ("Position.x"=w577:dbl, "Position.y"=w575:dbl)
                            n98 = Subtract(x=w578, y=w577) -> (x-y=w574:dbl)
                            n99 = Subtract(x=w576, y=w575) -> (x-y=w573:dbl)
                            n100 = Square(x=w574) -> (x^2=w572:dbl)
                            n101 = Square(x=w573) -> (x^2=w571:dbl)
                            n102 = local read "# of Spots"() -> (w565:dbl)
                            n103 = Add(x=w572, y=w571) -> (x+y=w570:dbl)
                            n104 = local read "Buffer Zone"() -> (w560:dbl)
                            n105 = Square Root(x=w570) -> (sqrt(x)=w569:dbl)
                            n106 = Multiply(x=2, y=w560) -> (x*y=w558:dbl)
                            n107 = Less?(x=w569, y=w558) -> (x < y?=w567:bool)
                            n108 = Not Equal?(x=w561, y=w563) -> (x != y?=w566:bool)
                            n109 = Equal?(x=w565, y=w563) -> (x = y?=w568:bool)
                            n110 = And(x=w566, y=w567) -> (x .and. y?=w564:bool)
                            "Looper" <- w564
                            n111 = Or(x=w564, y=w568) -> (x .or. y?=w562:bool)
                          }
                        }
                        frame #1 {
                          n112 = local read "Looper"() -> (w581:bool)
                          n113 = case shown="False" w581 {
                            frame False {
                              n114 = local read "init"() -> (w582:dbl)
                              n115 = Add(x=w582, y=1) -> (x+y=w584:dbl)
                              n116 = local write "init"(w584) -> ()
                            }
                            frame True {
                            }
                          }
                        }
                      }
                      n117 = local read "Looper"() -> (w552:bool)
                    }
                  }
                  frame #2 {
                    n118 = local read "Looper"() -> (w589:bool)
                    n119 = case shown="True" w589 {
                      tunnel: w587 -> [w593 _]
                      tunnel: w586 -> [_ w601]
                      tunnel: ["This is an acceptable entry." "ERROR: A bubble will intersect the buffer zone."] -> w588
                      tunnel: [w593 w601] -> w585
                      frame False {
                        n120 = local write "Looper"(FALSE) -> ()
                        n121 = local read "Current Spot #"() -> (w594:dbl)
                        n122 = Index Array(array=w593, index=w594) -> (element=w592:T1)
                        n123 = Unbundle By Name(w592) -> ("Position.x"=w591:dbl, "Position.y"=w590:dbl)
                        n124 = local write "New Y"(w590) -> ()
                        n125 = local write "New X"(w591) -> ()
                      }
                      frame True {
                        # "Restore original position"
                        n126 = local write "Looper"(FALSE) -> ()
                        n127 = local read "Old Y"() -> (w598:dbl)
                        n128 = local read "Old X"() -> (w599:dbl)
                        n129 = local read "Position"() -> (w597:cluster{"x":dbl, "y":dbl, "z":dbl})
                        n130 = Bundle By Name(cluster=w597, "x"=w599, "y"=w598) -> (w600:cluster{"x":dbl, "y":dbl, "z":dbl})
                        n131 = local write "Position"(w600) -> ()
                      }
                    }
                  }
                }
                "Position Indicator" <- w516
              }
              event "Size": Value Change {
                # "If we were constraining the aspect ratio, or preventing a divide by zero, the size control on the FP may be incorrect.  We refresh it in here to stop it displaying a wrong value."
                # "If the size has changed, scale the spots"
                n132 = event-data() -> ("OldVal"=w610:cluster{"x":dbl, "y":dbl, "z":dbl}, "NewVal"=w616:cluster{"x":dbl, "y":dbl, "z":dbl})  [unwired: 5 out]
                n133 = Not Equal?(x=w610, y=w616) -> (x != y?=w609:cluster{"x":bool, "y":bool, "z":bool})
                n134 = Divide(x=w616, y=w610) -> (x/y=w615:cluster{"x":dbl, "y":dbl, "z":dbl})
                n135 = Not Equal To 0?(x=w610) -> (x != 0?=w608:cluster{"x":bool, "y":bool, "z":bool})
                n136 = And(x=w609, y=w608) -> (x .and. y?=w607:cluster{"x":bool, "y":bool, "z":bool})
                n137 = Cluster To Array(cluster=w607) -> (array=w614:bool[])
                n138 = Cluster To Array(cluster=w615) -> (array=w613:dbl[])
                n139 = case shown="True" "lock aspect ratio" {
                  tunnel: w614 -> [w622 w639]
                  tunnel: w613 -> [w621 w637]
                  tunnel: [w619 w629] -> w612
                  frame False {
                    # "We are not constraining the aspect ratio here, so just check we're not introducing NAs"
                    n140 = for {
                      tunnel: w622 -> [w628] mode=indexing
                      tunnel: w621 -> [w624] mode=indexing
                      tunnel: [w626] -> w620 mode=indexing
                      n141 = Not A Number/Path/Refnum?(number/path/refnum=w624) -> (NaN/Path/Refnum?=w625:bool)
                      n142 = Compound Arithmetic op=AND(w628, invert w625) -> (w627:bool)
                      n143 = Select(t=w624, s=w627, f=1.0) -> (s? t:f=w626:dbl)
                    }
                    n144 = Array To Cluster(array=w620) -> (cluster=w619:cluster{"[0]":dbl, "[1]":dbl, "[2]":dbl})
                  }
                  frame True {
                    # "Pick the first element that changed and use it.  Also need to make sure (1) an element did change and (2) everything's valid (no divide by zeros)"
                    n145 = Search 1D Array(1D array=w639, element=TRUE) -> (index of element=w636:i32)  [unwired: 1 in]
                    n146 = Index Array(array=w637, index=w636) -> (element=w632:dbl)
                    n147 = Not A Number/Path/Refnum?(number/path/refnum=w632) -> (NaN/Path/Refnum?=w635:bool)
                    n148 = Less Than 0?(x=w636) -> (x < 0?=w634:bool)
                    n149 = Or(x=w635, y=w634) -> (x .or. y?=w633:bool)
                    n150 = Select(t=1.0, s=w633, f=w632) -> (s? t:f=w630:dbl)
                    n151 = Bundle("x"=w630, "x"=w630, "x"=w630) -> (w629:cluster{"x":dbl, "x":dbl, "x":dbl})  [unwired: 1 in]
                  }
                }
                n152 = for {
                  tunnel: w618 -> [w645] mode=indexing
                  tunnel: w605 -> [w642] mode=indexing
                  tunnel: [w644] -> w606 mode=indexing
                  tunnel: w612 -> [w643]
                  tunnel: w617 -> [w640]
                  n153 = Unbundle(w642) -> ("Selected"=w641:bool)  [unwired: 1 out]
                  n154 = case shown="True" w641 {
                    tunnel: w645 -> [w646 w654]
                    tunnel: [w646 w653] -> w644
                    tunnel: w643 -> [_ w652]
                    tunnel: w640 -> [_ w648]
                    frame False {
                    }
                    frame True {
                      n155 = call "extract_position.vi"("Spot"=w654) -> ("Position"=w650:cluster{"x":dbl, "y":dbl, "z":dbl})
                      n156 = Subtract(x=w650, y=w648) -> (x-y=w651:cluster{"x":dbl, "y":dbl, "z":dbl})
                      n157 = Multiply(x=w651, y=w652) -> (x*y=w649:cluster{"x":dbl, dbl, dbl})
                      n158 = Add(x=w648, y=w649) -> (x+y=w647:cluster{"x":dbl, dbl, dbl})
                      n159 = call "replace_position.vi"("Position"=w647, "Spot in"=w654) -> ("Spot"=w653:T1)  [unwired: 2 out]
                    }
                  }
                }
                n160 = call "find_centroid.vi"("Selection and Groups"=w605, "Spots"=w606) -> ("size"=w604:cluster{"x":dbl, "y":dbl, "z":dbl})  [unwired: 2 in, 4 out]
                n161 = local write "Size"(w604) -> ()
              }
              event "Intensity": Value Change {
                # "When  the user changes intensity, scale all the spots selected so the new mean is correct but keep the ratio between the selected spots.\n\nThe exception to this is when the mean intensity is zero, in which case multiplying makes no sense- in that case we just replace with the new value."
                n162 = event-data() -> ("NewVal"=w655:dbl, "OldVal"=w662:dbl)  [unwired: 5 out]
                n163 = Equal To 0?(x=w662) -> (x = 0?=w658:bool)
                n164 = Not A Number/Path/Refnum?(number/path/refnum=w662) -> (NaN/Path/Refnum?=w657:bool)
                n165 = Or(x=w658, y=w657) -> (x .or. y?=w656:bool)
                n166 = Divide(x=w655, y=w662) -> (x/y=w659:dbl)
                n167 = for {
                  tunnel: w663 -> [w668] mode=indexing
                  tunnel: w660 -> [w670] mode=indexing
                  tunnel: [w667] -> w661 mode=indexing
                  tunnel: w659 -> [w666]
                  tunnel: w656 -> [w665]
                  tunnel: w655 -> [w664]
                  n168 = Unbundle(w670) -> ("Selected"=w669:bool)  [unwired: 1 out]
                  n169 = case shown="True" w669 {
                    tunnel: w668 -> [w671 w678]
                    tunnel: [w671 w675] -> w667
                    tunnel: w666 -> [_ w674]
                    tunnel: w665 -> [_ w673]
                    tunnel: w664 -> [_ w672]
                    frame False {
                    }
                    frame True {
                      n170 = Unbundle By Name(w678) -> ("Intensity"=w676:dbl)
                      n171 = case shown="True" w673 {
                        tunnel: [w681 w682] -> w677
                        tunnel: w676 -> [w680 _]
                        tunnel: w674 -> [w679 _]
                        tunnel: w672 -> [_ w682]
                        frame False {
                          n172 = Multiply(x=w680, y=w679) -> (x*y=w681:dbl)
                        }
                        frame True {
                        }
                      }
                      n173 = Bundle By Name(cluster=w678, "Intensity"=w677) -> (w675:T1)
                    }
                  }
                }
              }
              event "phase": Value Change {
                # "When  the user changes phase, translate the phase of all spots selectedd"
                n174 = event-data() -> ("NewVal"=w684:dbl, "OldVal"=w688:dbl)  [unwired: 5 out]
                n175 = Not A Number/Path/Refnum?(number/path/refnum=w688) -> (NaN/Path/Refnum?=w683:bool)
                n176 = Subtract(x=w684, y=w688) -> (x-y=w685:dbl)
                n177 = for {
                  tunnel: w689 -> [w694] mode=indexing
                  tunnel: w686 -> [w696] mode=indexing
                  tunnel: [w693] -> w687 mode=indexing
                  tunnel: w685 -> [w692]
                  tunnel: w683 -> [w691]
                  tunnel: w684 -> [w690]
                  n178 = Unbundle(w696) -> ("Selected"=w695:bool)  [unwired: 1 out]
                  n179 = case shown="False" w695 {
                    tunnel: w694 -> [w697 w704]
                    tunnel: [w697 w701] -> w693
                    tunnel: w692 -> [_ w700]
                    tunnel: w691 -> [_ w699]
                    tunnel: w690 -> [_ w698]
                    frame False {
                    }
                    frame True {
                      n180 = Unbundle By Name(w704) -> ("Phase"=w702:dbl)
                      n181 = case shown="False" w699 {
                        tunnel: [w707 w708] -> w703
                        tunnel: w702 -> [w706 _]
                        tunnel: w700 -> [w705 _]
                        tunnel: w698 -> [_ w708]
                        frame False {
                          n182 = Add(x=w706, y=w705) -> (x+y=w707:dbl)
                        }
                        frame True {
                        }
                      }
                      n183 = Bundle By Name(cluster=w704, "Phase"=w703) -> (w701:T1)
                    }
                  }
                }
              }
              event "Vortex Charge": Value Change {
                # "When  the user changes l, just set all selected spots to have that value of l."
                n184 = event-data() -> ("NewVal"=w709:i8)  [unwired: 6 out]
                n185 = for {
                  tunnel: w712 -> [w715] mode=indexing
                  tunnel: w710 -> [w717] mode=indexing
                  tunnel: [w714] -> w711 mode=indexing
                  tunnel: w709 -> [w713]
                  n186 = Unbundle(w717) -> ("Selected"=w716:bool)  [unwired: 1 out]
                  n187 = case shown="True" w716 {
                    tunnel: w715 -> [w718 w721]
                    tunnel: [w718 w720] -> w714
                    tunnel: w713 -> [_ w719]
                    frame False {
                    }
                    frame True {
                      n188 = Bundle By Name(cluster=w721, "Vortex Charge"=w719) -> (w720:T1)
                    }
                  }
                }
              }
            }
          }
          frame "Spot Shape" {
            # "We update the spot shape tab only when spots have changed OUTSIDE this tab.  This avoids unnecessary jumping about of the tab control."
            n189 = call "find_centroid.vi"("Selection and Groups"=w732, "Spots"=w733) -> ("Mean Values"=w728:T1)  [unwired: 2 in, 4 out]
            n190 = Wait (ms)(milliseconds to wait=u32 10) -> ()  [unwired: 1 out]
            n191 = call "spots_shape.vi"("Selection and Groups"=w732, "Spots"=w733) -> ("Spot Shape"=w735:enum32{"Normal", "Line", "NA", "Mixed"})  [unwired: 7 in]
            n192 = feedback-in #4(w728) -> ()
            n193 = feedback #4() -> (w729:T1)  [unwired: 1 in]
            n194 = Not Equal?(x=w729, y=w728) -> (x != y?=w734:bool)
            n195 = feedback #5() -> (w724:enum32{"Normal", "Line", "NA", "Mixed"})  [unwired: 1 in]
            n196 = feedback #6() -> (w726:T1)  [unwired: 1 in]
            n197 = Not Equal?(x=w726, y=w728) -> (x != y?=w725:bool)
            n198 = case shown="False" w725 {
              tunnel: w735 -> [_ w854]
              tunnel: ["Spot Shape" w854] -> w723
              frame False {
              }
              frame True {
                n199 = local write "Spot Shape"(w854) -> ()
              }
            }
            n200 = feedback-in #5(w723) -> ()
            n201 = Not Equal?(x=w723, y=w724) -> (x != y?=w722:bool)
            n202 = case shown="\"Normal\", Default" w723 {
              tunnel: w733 -> [w739 w756 w782 w852]
              tunnel: w732 -> [w738 w755 w781 w851]
              tunnel: [w738 w754 w779 w851] -> w730
              tunnel: [w737 w753 w780 w852] -> w731
              tunnel: w728 -> [_ w752 w778 _]
              tunnel: w734 -> [_ w751 w777 _]
              tunnel: w722 -> [_ w749 w775 _]
              frame "Normal", Default {
                # "If \"normal\" is selected, don't allow any NA or line-trapping stuff"
                n203 = for {
                  tunnel: w739 -> [w742] mode=indexing
                  tunnel: w738 -> [w741] mode=indexing
                  tunnel: [w743] -> w737 mode=indexing
                  n204 = Unbundle(w741) -> ("Selected"=w740:bool)  [unwired: 1 out]
                  n205 = case shown="True" w740 {
                    tunnel: [w744 w748] -> w743
                    tunnel: w742 -> [w744 w747]
                    frame False {
                    }
                    frame True {
                      n206 = Bundle By Name(cluster=w747, "NA Position"=cluster{"x":dbl, "y":dbl, "r":dbl} {"x"=0.0, "y"=0.0, "r"=1.0} ("x"), "Line Trapping"=T2 {"Vector"={"x"=0.0, "y"=0.0, "z"=0.0}, "Phase Gradient"=0.0}) -> (w748:T1)
                    }
                  }
                }
              }
              frame "Line" {
                # "If it's out of date, update front panel"
                n207 = Or(x=w751, y=w749) -> (x .or. y?=w750:bool)
                n208 = case shown="True" w750 {
                  tunnel: w752 -> [_ w759]
                  frame False {
                  }
                  frame True {
                    n209 = Unbundle By Name(w759) -> ("Line Trapping"=w758:T2)
                    n210 = local write "Line Trapping"(w758) -> ()
                  }
                }
                n211 = event shown="[1] \"Line Trapping\": Value Change" {
                  selector: _ -> [_ _]
                  dyn-events: _ -> [_ _]
                  timeout: 10 -> [_ _]
                  tunnel: w756 -> [w761 w765]
                  tunnel: w755 -> [w760 w763]
                  tunnel: [w761 w764] -> w753
                  tunnel: [w760 w763] -> w754
                  event Timeout {
                    n212 = event-data() -> ()  [unwired: 3 out]
                  }
                  event Value Change {
                    # "If the line vector has changed, update it"
                    n213 = event-data() -> ("NewVal"=w762:T2)  [unwired: 6 out]
                    n214 = for {
                      tunnel: w765 -> [w770] mode=indexing
                      tunnel: w763 -> [w767] mode=indexing
                      tunnel: [w769] -> w764 mode=indexing
                      tunnel: w762 -> [w768]
                      n215 = Unbundle(w767) -> ("Selected"=w766:bool)  [unwired: 1 out]
                      n216 = case shown="True" w766 {
                        tunnel: w770 -> [w771 w773]
                        tunnel: [w771 w774] -> w769
                        tunnel: w768 -> [_ w772]
                        frame False {
                        }
                        frame True {
                          n217 = Bundle By Name(cluster=w773, "Line Trapping"=w772) -> (w774:T1)
                        }
                      }
                    }
                  }
                }
              }
              frame "NA" {
                n218 = Or(x=w775, y=w777) -> (x .or. y?=w776:bool)
                n219 = case shown="True" w776 {
                  tunnel: w778 -> [_ w787]
                  frame False {
                  }
                  frame True {
                    n220 = Unbundle By Name(w787) -> ("NA Position"=w786:cluster{"x":dbl, "y":dbl, "r":dbl})
                    n221 = call "xyz_to_xy.vi"("Position"=w786) -> ("Position (2D)"=w785:cluster{"x":dbl, "y":dbl}, "z"=w784:dbl)  [unwired: 6 out]
                    n222 = local write "Position on back aperture"(w785) -> ()
                    n223 = local write "Radius on back aperture"(w784) -> ()
                  }
                }
                n224 = event shown="[3] \"Scale BA\": Value Change" {
                  selector: _ -> [_ _ _ _]
                  dyn-events: _ -> [_ _ _ _]
                  timeout: 10 -> [_ _ _ _]
                  tunnel: w782 -> [w789 w795 w816 w838]
                  tunnel: w781 -> [w788 w793 w813 w839]
                  tunnel: [w789 w794 w814 w836] -> w780
                  tunnel: [w788 w793 w813 w839] -> w779
                  event Timeout {
                    n225 = event-data() -> ()  [unwired: 3 out]
                  }
                  event "Position on back aperture": Value Change {
                    # "If the position has changed, translate the spots"
                    n226 = event-data() -> ("OldVal"=w791:cluster{"x":dbl, "y":dbl}, "NewVal"=w792:cluster{"x":dbl, "y":dbl})  [unwired: 5 out]
                    n227 = Subtract(x=w792, y=w791) -> (x-y=w790:cluster{"x":dbl, "y":dbl})
                    n228 = for {
                      tunnel: w795 -> [w800] mode=indexing
                      tunnel: w793 -> [w797] mode=indexing
                      tunnel: [w799] -> w794 mode=indexing
                      tunnel: w790 -> [w798]
                      n229 = Unbundle(w797) -> ("Selected"=w796:bool)  [unwired: 1 out]
                      n230 = case shown="True" w796 {
                        tunnel: w800 -> [w801 w803]
                        tunnel: [w801 w804] -> w799
                        tunnel: w798 -> [_ w805]
                        frame False {
                        }
                        frame True {
                          n231 = Unbundle By Name(w803) -> ("NA Position"=w807:cluster{"x":dbl, "y":dbl, "r":dbl})
                          n232 = call "xy_to_xyz.vi"("Position (2D)"=w805) -> ("Position (3D)"=w806:cluster{dbl, dbl, dbl})  [unwired: 1 in, 2 out]
                          n233 = Add(x=w807, y=w806) -> (x+y=w802:cluster{dbl, dbl, dbl})
                          n234 = Bundle By Name(cluster=w803, "NA Position"=w802) -> (w804:T1)
                        }
                      }
                    }
                  }
                  event "Radius on back aperture": Value Change {
                    # "When  the user changes intensity, scale all the spots selected so the new mean is correct but keep the ratio between the selected spots.\n\nThe exception to this is when the mean intensity is zero, in which case multiplying makes no sense- in that case we just replace with the new value."
                    n235 = event-data() -> ("NewVal"=w808:dbl, "OldVal"=w815:dbl)  [unwired: 5 out]
                    n236 = Equal To 0?(x=w815) -> (x = 0?=w811:bool)
                    n237 = Not A Number/Path/Refnum?(number/path/refnum=w815) -> (NaN/Path/Refnum?=w810:bool)
                    n238 = Or(x=w811, y=w810) -> (x .or. y?=w809:bool)
                    n239 = Divide(x=w808, y=w815) -> (x/y=w812:dbl)
                    n240 = for {
                      tunnel: w816 -> [w821] mode=indexing
                      tunnel: w813 -> [w823] mode=indexing
                      tunnel: [w820] -> w814 mode=indexing
                      tunnel: w812 -> [w819]
                      tunnel: w809 -> [w818]
                      tunnel: w808 -> [w817]
                      n241 = Unbundle(w823) -> ("Selected"=w822:bool)  [unwired: 1 out]
                      n242 = case shown="True" w822 {
                        tunnel: w821 -> [w824 w831]
                        tunnel: [w824 w828] -> w820
                        tunnel: w819 -> [_ w827]
                        tunnel: w818 -> [_ w826]
                        tunnel: w817 -> [_ w825]
                        frame False {
                        }
                        frame True {
                          n243 = Unbundle By Name(w831) -> ("NA Position.r"=w829:dbl)
                          n244 = case shown="False" w826 {
                            tunnel: [w834 w835] -> w830
                            tunnel: w829 -> [w833 _]
                            tunnel: w827 -> [w832 _]
                            tunnel: w825 -> [_ w835]
                            frame False {
                              n245 = Multiply(x=w833, y=w832) -> (x*y=w834:dbl)
                            }
                            frame True {
                            }
                          }
                          n246 = Bundle By Name(cluster=w831, "NA Position.r"=w830) -> (w828:T1)
                        }
                      }
                    }
                  }
                  event "Scale BA": Value Change {
                    n247 = event-data() -> ()  [unwired: 7 out]
                    n248 = for {
                      tunnel: w839 -> [w844] mode=indexing
                      tunnel: w838 -> [w842] mode=indexing
                      tunnel: "Scale back aperture" -> [w841]
                      tunnel: [w840] -> w836 mode=indexing
                      n249 = Unbundle(w844) -> ("Selected"=w843:bool)  [unwired: 1 out]
                      n250 = case shown="True" w843 {
                        tunnel: w842 -> [w845 w846]
                        tunnel: w841 -> [_ w849]
                        tunnel: [w845 w847] -> w840
                        frame False {
                        }
                        frame True {
                          n251 = Unbundle By Name(w846) -> ("NA Position"=w850:cluster{"x":dbl, "y":dbl, "r":dbl})
                          n252 = Multiply(x=w849, y=w850) -> (x*y=w848:cluster{"x":dbl, "y":dbl, "r":dbl})
                          n253 = Bundle By Name(cluster=w846, "NA Position"=w848) -> (w847:T1)
                        }
                      }
                    }
                  }
                }
              }
              frame "Mixed" {
              }
            }
            n254 = call "find_centroid.vi"("Selection and Groups"=w730, "Spots"=w731) -> ("Mean Values"=w727:T1)  [unwired: 2 in, 4 out]
            n255 = feedback-in #6(w727) -> ()
          }
          frame "Rotate" {
            w865 = u32 0 items=["Frame", "Fill", "Highlight"] ("Drawing Mode")
            w864 = u32 0 ("Color")
            w861 = i16 100 ("radius")
            # "It's necessary to check this has changed to stop us unintentionally \"spinning\" the spots..."
            # "Draw the centroid as a spot, then a large circle+cross"
            # "It's important that this loop doesn't go too fast- it hogs the CPU.  However, each tab can have a different loop speed."
            n256 = Unbundle By Name(w858) -> ("Position (Image Pixels)"=w874:cluster{"X":dbl, "Y":dbl}, "Previous Position (Image Pixels)"=w873:cluster{"X":dbl, "Y":dbl}, "Dragging"=w875:bool)
            n257 = feedback-in #7(w858) -> ()
            n258 = feedback #7() -> (w859:T9)  [unwired: 1 in]
            n259 = call "find_centroid.vi"("Selection and Groups"=w876, "Spots"=w879) -> ("centroid"=w872:cluster{"x":dbl, "y":dbl, "z":dbl})  [unwired: 2 in, 4 out]
            n260 = Not Equal?(x=w858, y=w859) -> (x != y?=w856:bool)
            n261 = Wait (ms)(milliseconds to wait=u32 10) -> ()  [unwired: 1 out]
            n262 = And(x=w856, y=w875) -> (x .and. y?=w857:bool)
            n263 = call "coords_real_to_image_currentview.vi"("Position (real coords)"=w872) -> ("Position (pixels, relative to the top left of the image)"=w855:cluster{dbl, dbl})  [unwired: 7 in, 1 out]
            n264 = case shown="True" w857 {
              tunnel: w879 -> [w888 w932]
              tunnel: [w890 w931] -> w878
              tunnel: w876 -> [w889 w933]
              tunnel: [w889 w933] -> w877
              tunnel: w872 -> [w887 w924]
              tunnel: w874 -> [_ w923]
              tunnel: w873 -> [_ w922]
              tunnel: w855 -> [_ w921]
              frame False {
                n265 = event shown="[1] Timeout" {
                  selector: _ -> [_ _]
                  dyn-events: _ -> [_ _]
                  timeout: 10 -> [_ _]
                  tunnel: [w903 w920] -> w890
                  tunnel: w889 -> [w902 _]
                  tunnel: w888 -> [w901 w920]
                  tunnel: w887 -> [w897 _]
                  event "rotate": Value Change {
                    n266 = event-data() -> ()  [unwired: 6 out]
                    n267 = case shown="3" "Rotation Axis" {
                      tunnel: [cluster{dbl, dbl, dbl} {0.0, 0.0, 1.0} ("Custom Axis") cluster{dbl, dbl, dbl} {1.0, 0.0, 0.0} ("Custom Axis") cluster{dbl, dbl, dbl} {0.0, 1.0, 0.0} ("Custom Axis") "Custom Axis"] -> w898
                      frame 0, Default {
                        # "Z"
                      }
                      frame 1 {
                        # "X"
                      }
                      frame 2 {
                        # "Y"
                      }
                      frame 3 {
                      }
                    }
                    n268 = call "normalise_3d_vector.vi"("Vector"=w898) -> ("Unit Vector"=w900:cluster{dbl, dbl, dbl})  [unwired: 3 out]
                    n269 = Divide(x=6.283185307179586, y=360.0) -> (x/y=w895:dbl)
                    n270 = Multiply(x="Angle (degrees)", y=w895) -> (x*y=w892:dbl)
                    n271 = call "arb_rotation_matrix.vi"("Unit Vector"=w900, "theta"=w892) -> ("Real Matrix"=w904:T15)
                    n272 = for {
                      tunnel: w902 -> [w914] mode=indexing
                      tunnel: w901 -> [w909] mode=indexing
                      tunnel: [w910] -> w903 mode=indexing
                      tunnel: w897 -> [w912]
                      tunnel: w904 -> [w911]
                      n273 = Unbundle(w914) -> ("Selected"=w913:bool)  [unwired: 1 out]
                      n274 = case shown="True" w913 {
                        tunnel: w912 -> [_ w919]
                        tunnel: [w915 w918] -> w910
                        tunnel: w909 -> [w915 w917]
                        tunnel: w911 -> [_ w916]
                        frame False {
                        }
                        frame True {
                          n275 = call "apply_matrix_transformation_to_spots.vi"("Transform centre (i.e. transform about this point)"=w919, "Transformation Matrix (3x3)"=w916, "Spot In"=w917) -> ("Spot Out"=w918:T1)  [unwired: 5 out]
                        }
                      }
                    }
                  }
                  event Timeout {
                    n276 = event-data() -> ()  [unwired: 4 out]
                  }
                }
              }
              frame True {
                # "if the mouse has not moved, stuff will be NaN, so let's make like a leopard and not change our spots"
                # "the magnitude of the change in our direction vector gives the rotation angle in radians"
                # "If it's within 100px of the centroid, pretend the mouse is on the surface of a sphere, and synthesize Z accordingly (z^2=100^2-x^2-y^2).  This allows rotation in 3d :)  The output should always be a unit vector."
                n277 = Build Array(w923, w922) -> (w938:cluster{"X":dbl, "Y":dbl}[])
                n278 = for {
                  tunnel: w921 -> [w971]
                  tunnel: w938 -> [w967] mode=indexing
                  tunnel: [w957] -> w937 mode=indexing
                  n279 = Subtract(x=w967, y=w971) -> (x-y=w962:cluster{dbl, dbl})
                  n280 = Divide(x=w962, y=100.0 ("x")) -> (x/y=w963:cluster{dbl, dbl})
                  n281 = Square(x=w963) -> (x^2=w970:cluster{dbl, dbl})
                  n282 = Unbundle(w970) -> (w968:dbl, w969:dbl)
                  n283 = Add(x=w968, y=w969) -> (x+y=w959:dbl)
                  n284 = Subtract(x=1.0, y=w959) -> (x-y=w965:dbl)
                  n285 = Square Root(x=w959) -> (sqrt(x)=w960:dbl)
                  n286 = Greater Than 0?(x=w965) -> (x > 0?=w966:bool)
                  n287 = case shown="False" w966 {
                    tunnel: w965 -> [_ w978]
                    tunnel: [0.0 w977] -> w956
                    tunnel: w963 -> [w975 w976]
                    tunnel: w960 -> [w974 _]
                    tunnel: [w973 w976] -> w958
                    frame False {
                      n288 = Divide(x=w975, y=w974) -> (x/y=w973:cluster{dbl, dbl})
                    }
                    frame True {
                      n289 = Square Root(x=w978) -> (sqrt(x)=w977:dbl)
                    }
                  }
                  n290 = call "xy_to_xyz.vi"("z"=w956, "Position (2D)"=w958) -> ("Position (3D)"=w957:cluster{dbl, dbl, dbl})  [unwired: 2 out]
                }
                n291 = Index Array(array=w937) -> (element #1=w936:cluster{dbl, dbl, dbl}, element #2=w927:cluster{dbl, dbl, dbl})  [unwired: 2 in]
                n292 = Add(x=w936, y=w927) -> (x+y=w926:cluster{dbl, dbl, dbl})
                n293 = Subtract(x=w936, y=w927) -> (x-y=w925:cluster{dbl, dbl, dbl})
                n294 = call "cross_product.vi"("b"=w926, "a"=w925) -> ("a cross b"=w935:cluster{dbl, dbl, dbl})
                n295 = call "normalise_3d_vector.vi"("Vector"=w935) -> ("Unit Vector"=w934:cluster{dbl, dbl, dbl})  [unwired: 3 out]
                n296 = call "normalise_3d_vector.vi"("Vector"=w925) -> ("magnitude"=w929:dbl)  [unwired: 3 out]
                n297 = Not Equal To 0?(x=w929) -> (x != 0?=w928:bool)
                n298 = call "arb_rotation_matrix.vi"("Unit Vector"=w934, "theta"=w929) -> ("Real Matrix"=w930:T15)
                n299 = case shown="True" w928 {
                  tunnel: w933 -> [_ w944]
                  tunnel: w932 -> [w939 w943]
                  tunnel: [w939 w942] -> w931
                  tunnel: w930 -> [_ w941]
                  tunnel: w924 -> [_ w940]
                  frame False {
                  }
                  frame True {
                    n300 = for {
                      tunnel: w944 -> [w950] mode=indexing
                      tunnel: w943 -> [w947] mode=indexing
                      tunnel: [w946] -> w942 mode=indexing
                      tunnel: w941 -> [w948]
                      tunnel: w940 -> [w945]
                      n301 = Unbundle(w950) -> ("Selected"=w949:bool)  [unwired: 1 out]
                      n302 = case shown="True" w949 {
                        tunnel: [w951 w954] -> w946
                        tunnel: w947 -> [w951 w955]
                        tunnel: w948 -> [_ w952]
                        tunnel: w945 -> [_ w953]
                        frame False {
                        }
                        frame True {
                          n303 = call "apply_matrix_transformation_to_spots.vi"("Transform centre (i.e. transform about this point)"=w953, "Transformation Matrix (3x3)"=w952, "Spot In"=w955) -> ("Spot Out"=w954:T1)  [unwired: 5 out]
                        }
                      }
                    }
                  }
                }
              }
            }
            n304 = call "coords_real_to_image_currentview.vi"("Position (real coords)"=w872) -> ("Position (pixels, relative to the top left of the image)"=w867:cluster{dbl, dbl}, "z (real coords)"=w871:dbl)  [unwired: 7 in]
            n305 = expression code="z*1e7+20"(w871) -> (w883:dbl)
            n306 = In Range and Coerce(upper limit=100.0, x=w883, lower limit=2.0) -> (coerced(x)=w870:dbl)  [unwired: 1 out]
            n307 = Bundle("upper limit"=w870, "upper limit"=w870) -> (w863:cluster{"upper limit":dbl, "upper limit":dbl})  [unwired: 1 in]
            n308 = call "myoverlay_oval.vi"("Color"=w864, "Drawing Mode"=w865, "Size"=w863, "Centre Position (pixels on image)"=w867) -> ("Overlay Elements Out"=w869:T16[])  [unwired: 5 in]
            n309 = Bundle("radius"=w861, "radius"=w861) -> (w862:cluster{"radius":i16, "radius":i16})  [unwired: 1 in]
            n310 = call "myoverlay_oval.vi"("Color"=w864, "Drawing Mode"=w865, "Size"=w862, "Centre Position (pixels on image)"=w867, "Overlay Elements In"=w869) -> ("Overlay Elements Out"=w868:T16[])  [unwired: 4 in]
            n311 = Multiply(x=w861, y=cluster{dbl, dbl}[] [{0.0, 0.0}, {1.0, 0.0}, {0.0, 0.0}, {0.0, 1.0}, {0.0, 0.0}, {-1.0, 0.0}, {0.0, 0.0}, {0.0, -1.0}, {0.0, 0.0}]) -> (x*y=w880:cluster{dbl, dbl}[])
            n312 = Add(x=w867, y=w880) -> (x+y=w866:cluster{dbl, dbl}[])
            n313 = call "myoverlay_lines.vi"("Color"=w864, "Drawing Mode"=w865, "Line Endpoints"=w866, "Overlay Elements In"=w868) -> ("Overlay Elements Out"=w860:T16[])  [unwired: 5 in]
          }
          frame "Patterns" {
            n314 = event shown="[3] \"Optimise\": Value Change" {
              selector: _ -> [_ _ _ _ _]
              dyn-events: _ -> [_ _ _ _ _]
              timeout: u32 10 ("milliseconds to wait") -> [_ _ _ _ _]
              tunnel: [w997 w1027 w1031 w1034 w1045] -> w980
              tunnel: [w996 w1028 w1030 w1037 w1046] -> w979
              tunnel: w982 -> [w995 w1027 w1031 w1035 w1044]
              tunnel: w981 -> [w994 w1028 w1030 w1037 w1046]
              event "Generate": Value Change {
                # "If there were previous spots, centre the pattern on the spots"
                n315 = event-data() -> ()  [unwired: 1 in, 1 out]
                n316 = call "find_centroid.vi"("Selection and Groups"=w994, "Spots"=w995) -> ("size"=w990:cluster{"x":dbl, "y":dbl, "z":dbl}, "centroid"=w986:cluster{"x":dbl, "y":dbl, "z":dbl}, "# selected"=w992:i16)  [unwired: 2 in, 2 out]
                n317 = Greater?(x=w992, y=i16 1) -> (0:w987:bool)
                n318 = case shown="False" w987 {
                  tunnel: w990 -> [_ w1013]
                  tunnel: [cluster{"x":dbl, "y":dbl, "z":dbl} {"x"=2e-05, "y"=2e-05, "z"=2e-05} ("size") w1013] -> w989
                  frame False {
                  }
                  frame True {
                  }
                }
                n319 = case shown="\"HCP Shack-Hartmann\"" "Pattern" {
                  tunnel: [w1015 w1018 w1024] -> w988
                  tunnel: w989 -> [_ w1017 _]
                  frame "Square Shack-Hartmann" {
                    n320 = call "patterns_square_shack_hartmann.vi"("N"="Spots across centre") -> ("Spots"=w1015:T1[])
                  }
                  frame "HCP Shack-Hartmann" {
                    n321 = Unbundle By Name(w1017) -> ("x"=w1016:dbl)
                    n322 = call "pattern_hcp_shack_hartmann.vi"("Width"=w1016, "Reference Array?"="Reference Array?", "Fraction of SLM"="Fraction of SLM", "N"="Spots across centre") -> ("Shack-Hartmann Spots"=w1018:T1[])  [unwired: 7 in]
                  }
                  frame "Rectangular Grid" {
                    n323 = call "patterns_rectangular_grid.vi"("spacing/m"="spacing/m", "N"="N") -> ("Spots"=w1024:T1[])
                  }
                }
                n324 = local write "Generate"(FALSE ("Generate")) -> ()
                n325 = case shown="True" w987 {
                  tunnel: w988 -> [w1000 w1004]
                  tunnel: w986 -> [_ w1006]
                  tunnel: [w1000 w1002] -> w998
                  frame False {
                  }
                  frame True {
                    n326 = call "find_centroid.vi"("Spots"=w1004) -> ("centroid"=w1005:cluster{"x":dbl, "y":dbl, "z":dbl}, "# selected"=→"# selected":i16)  [unwired: 3 in, 3 out]
                    n327 = Subtract(x=w1006, y=w1005) -> (x-y=w1003:cluster{"x":dbl, "y":dbl, "z":dbl})
                    n328 = for {
                      tunnel: w1004 -> [w1009] mode=indexing
                      tunnel: w1003 -> [w1008]
                      tunnel: [w1007] -> w1002 mode=indexing
                      n329 = call "extract_position.vi"("Spot"=w1009) -> ("Position"=w1010:cluster{"x":dbl, "y":dbl, "z":dbl})
                      n330 = Add(x=w1010, y=w1008) -> (x+y=w1011:cluster{"x":dbl, "y":dbl, "z":dbl})
                      n331 = call "replace_position.vi"("Position"=w1011, "Spot in"=w1009) -> ("Spot"=w1007:T1)  [unwired: 2 out]
                    }
                  }
                }
                "Last Pattern" <- w998
                n332 = call "ensure_selection_matches_spots.vi"("Select All (default: no)"=TRUE ("Select All (default: true)"), "Spots"=w998) -> ("Selection and Groups out"=w996:T7[], "Spots (duplicate)"=w997:T1[])  [unwired: 4 in]
              }
              event "Spots across centre", "Fraction of SLM", "Reference Array?", "N", "spacing/m", "Spots across centre": Value Change {
                n333 = event-data() -> ()  [unwired: 1 in, 1 out]
                n334 = local read "Last Pattern"() -> (w1026:T1[])
                n335 = Equal?(x=w1027, y=w1026) -> (x = y?=w1025:bool)
                n336 = case shown="True" w1025 {
                  selector: w1025 -> [_ w1029]
                  frame False {
                  }
                  frame True {
                    n337 = property on="Generate" class="Bool (strict)"("Val(Sgnl)"=w1029) -> ()  [unwired: 2 in, 2 out]
                  }
                }
              }
              event Timeout {
                n338 = event-data() -> ()  [unwired: 1 in, 1 out]
              }
              event "Optimise": Value Change {
                n339 = event-data() -> ()  [unwired: 1 in, 1 out]
                n340 = for {
                  N: "Iterations" -> [_]
                  tunnel: 203 ("Optimisation Resolution") -> [w1041]
                  shift-right: [w1042] -> w1034
                  shift-left: w1035 -> [w1043]
                  tunnel: "Fall-off/m" -> [w1038]
                  n341 = call "do_gsw_step.vi"("Optimisation Resolution"=w1041, "Sinc Zero"=w1038, "Spots In"=w1043) -> ("non-uniformity"=→"non-uniformity":dbl, "efficiency"=→"efficiency":dbl, "Spots Out"=w1042:T1[])  [unwired: 6 in]
                }
              }
              event "Reset Phase/Amplitude": Value Change {
                n342 = event-data() -> ()  [unwired: 1 in, 1 out]
                n343 = for {
                  tunnel: [w1049] -> w1045 mode=indexing
                  tunnel: w1044 -> [w1050] mode=indexing
                  n344 = Bundle By Name(cluster=w1050, "Phase"=0.0, "Amplitude Correction"=0.0) -> (w1049:T1)
                }
              }
            }
          }
          frame "Plugins" {
            # "The local variable ensures the references are  correct when they make it through to the \"close plugins\" block."
            # "This is the error from loading/unloading VIs on the front panel"
            n345 = control-ref of="Plugin Pnl"() -> (w1054:refnum<vi>)
            n346 = Wait (ms)(milliseconds to wait=u32 10) -> ()  [unwired: 1 out]
            n347 = feedback #8() -> (w1053:T3)
            n348 = feedback #9() -> (w1055:errorcluster)
            n349 = event shown="[1] \"Plugin:\": Value Change" {
              selector: _ -> [_ _ _]
              dyn-events: _ -> [_ _ _]
              timeout: 10 -> [_ _ _]
              tunnel: "Abort Plugin" -> [w1062 _ _]
              tunnel: "Plugin:" -> [w1067 _ w1083]
              tunnel: w1055 -> [w1066 w1081 w1085]
              tunnel: [w1065 w1076 w1084] -> w1056
              tunnel: [w1064 w1077 w1087] -> w1052
              tunnel: w1053 -> [w1068 w1078 w1086]
              tunnel: w1054 -> [_ w1079 _]
              event Timeout {
                n350 = event-data() -> ()  [unwired: 1 in, 2 out]
                n351 = Not(x=w1062) -> (.not. x?=w1063:bool)
                n352 = case shown="True" w1063 {
                  tunnel: w1068 -> [w1070 w1075]
                  tunnel: w1067 -> [_ w1074]
                  tunnel: w1066 -> [w1069 w1073]
                  tunnel: [w1069 w1072] -> w1065
                  tunnel: [w1070 w1071] -> w1064
                  frame False {
                  }
                  frame True {
                    n353 = call "plugins_run.vi"("Error In"=w1073, "Plugin Index"=w1074, "Plugins In"=w1075) -> ("Error Out"=w1072:errorcluster, "Plugins"=w1071:T3)  [unwired: 7 in]
                  }
                }
              }
              event "Plugin:": Value Change {
                n354 = event-data() -> ("NewVal"=w1080:u16)  [unwired: 1 in]
                n355 = call "plugins_switch.vi"("error in"=w1081, "Plugin Pnl"=w1079, "Plugin Index"=w1080, "Plugins In"=w1078) -> ("error out"=w1076:errorcluster, "Plugins Out"=w1077:T3)  [unwired: 4 in]
              }
              event "Abort Plugin": Value Change {
                n356 = event-data() -> ("NewVal"=w1082:bool)  [unwired: 1 in]
                n357 = case shown="True" w1082 {
                  tunnel: [w1089 w1094] -> w1087
                  tunnel: w1086 -> [w1089 w1093]
                  tunnel: w1085 -> [w1088 w1092]
                  tunnel: [w1088 w1091] -> w1084
                  tunnel: w1083 -> [_ w1090]
                  frame False {
                  }
                  frame True {
                    n358 = call "plugins_abort.vi"("Error In"=w1092, "Plugin Index"=w1090, "Plugins In"=w1093) -> ("Error Out"=w1091:errorcluster, "Plugins Out"=w1094:T3)  [unwired: 7 in]
                  }
                }
              }
            }
            n359 = feedback-in #8(w1052) -> ()
            n360 = feedback-in #9(w1056) -> ()
            n361 = local write "Plugins"(w1052) -> ()
          }
          frame "Video" {
            # "All the controls on this tab are in the bottom (camera) loop."
            n362 = Wait (ms)(milliseconds to wait=u32 10) -> ()  [unwired: 1 out]
            n363 = property on="Property Node" class="ImageControl"(reference=w1095) -> ("Image Information String"=→"Image Information":string)  [unwired: 1 in, 2 out]
          }
        }
      }
      event "Tab": Value Change {
        w1103 = T17 [enum."Video", enum."Particle Tracking"] items=["Current Spot", "Rotate", "Spot Shape", "Patterns", "Plugins", "Video", "Particle Tracking", "Clamping", "Blank"]
        w1108 = refnum<vi> refnum  # Image
        # "This allows us to disable custom mouse-handling for certain tabs.  It can also be done from within the \"mouse down\" event case."
        n364 = event-data() -> ("NewVal"=w1104:T4)  [unwired: 1 in, 3 out]
        n365 = Equal?(x=w1103, y=w1104) -> (x = y?=w1102:bool[])
        n366 = Or Array Elements(Boolean array=w1102) -> (logical OR=w1101:bool)
        n367 = Not(x=w1101) -> (.not. x?=w1100:bool)
        n368 = Select(t=w1107, s=w1100, f=w1108) -> (s? t:f=w1109:refnum<vi>)
        n369 = register-events(reference=w1111, w1109, w1108, w1108, w1108) -> (reference out=w1110:refnum<event-registration>)  [unwired: 1 in, 1 out]
      }
      event Menu Selection (User) {
        n370 = event-data() -> ("ItemTag"=w1119:string, "MenuRef"=w1112:refnum<k9>)  [unwired: 1 in]
        n371 = case shown="\"ToggleSavingData\"" w1119 {
          tunnel: w1123 -> [w1127 w1137 w1146 w1160 w1179 w1183 w1186 w1193 w1200 w1202 w1205 w1234 w1260 w1281 w1292 w1303 w1306 w1308 w1313 w1316]
          tunnel: w1122 -> [w1126 w1136 w1145 w1169 w1178 w1182 w1184 w1191 w1199 w1201 w1204 w1233 w1259 w1280 w1291 w1302 w1305 w1309 w1314 w1315]
          tunnel: [w1127 w1137 w1146 w1160 w1177 w1180 w1186 w1193 w1200 w1202 w1205 w1234 w1260 w1281 w1292 w1303 w1306 w1308 w1313 w1316] -> w1121
          tunnel: [w1126 w1136 w1145 w1169 w1176 w1181 w1185 w1192 w1198 w1203 w1206 w1233 w1259 w1280 w1291 w1302 w1305 w1309 w1314 w1315] -> w1120
          tunnel: [_ _ _ _ TRUE _ _ _ _ _ _ _ _ _ _ _ _ _ _ _] -> w1114
          tunnel: w1113 -> [_ _ _ _ _ _ _ _ _ _ _ w1232 w1258 w1272 _ _ _ _ _ _]
          tunnel: w1112 -> [_ _ _ _ _ _ _ _ _ _ _ w1223 w1252 w1275 w1286 w1297 _ _ _ _]
          frame "ToggleSavingData" {
            # "Data is saved from the middle loop: look there for an explanation."
            n372 = local read "Save Video"() -> (w1125:bool)
            n373 = Not(x=w1125) -> (.not. x?=w1124:bool)
            n374 = local write "Save Video"(w1124) -> ()
          }
          frame "SaveStateToFile" {
            # "Save the current settings (i.e. the values of all the controls in VIs that have [Red Tweezers Save Settings] in their documentation string) to a file."
            n375 = call "File Dialog"("prompt"="Please select a location to save the settings", "button label"="Save", "default name"="red_tweezers_settings.xml", "pattern (all files)"="*.xml" ("pattern label"), "pattern label"="XML Settings Files") -> ("selected path"=w1135:path, "cancelled"=w1128:bool)  [unwired: 7 in, 2 out]
            n376 = Not(x=w1128) -> (.not. x?=w1129:bool)
            n377 = case shown="True" w1129 {
              tunnel: w1135 -> [_ w1139]
              frame False {
              }
              frame True {
                n378 = Path To String(path=w1139) -> (string=w1138:string)
                n379 = call "settings_save_to_file.vi"("XML File Path"=w1139) -> ()  [unwired: 11 in]
                n380 = call "settings_filename_to_registry.vi"("Last Used Settings File"=w1138) -> ()  [unwired: 11 in]
              }
            }
          }
          frame "SaveStateToCurrentFile" {
            # "As SaveStateToFile, but using the current file (i.e. Save not Save As...)."
            n381 = global read "red_tweezers_globals_INTERNAL_VOLATILE.vi" "Current Settings File"() -> (w1144:path)
            n382 = call <vilib>:"Check if File or Folder Exists.vi"("path"=w1144) -> ("file or folder exists?"=w1143:bool, "dup path"=w1142:path)  [unwired: 8 in, 1 out]
            n383 = case shown="True" w1143 {
              selector: w1143 -> [_ w1157]
              tunnel: w1142 -> [_ w1158]
              tunnel: [w1149 w1158] -> w1141
              tunnel: [w1150 w1157] -> w1140
              frame False {
                n384 = call "File Dialog3"("prompt"="Please select a location to save the settings", "button label"="Save", "default name"="red_tweezers_settings.xml", "pattern (all files)"="*.xml" ("pattern label"), "pattern label"="XML Settings Files") -> ("selected path"=w1149:path, "cancelled"=w1156:bool)  [unwired: 7 in, 2 out]
                n385 = Not(x=w1156) -> (.not. x?=w1150:bool)
              }
              frame True {
              }
            }
            n386 = case shown="True" w1140 {
              tunnel: w1141 -> [_ w1148]
              frame False {
              }
              frame True {
                n387 = Path To String(path=w1148) -> (string=w1147:string)
                n388 = call "settings_save_to_file.vi"("XML File Path"=w1148) -> ()  [unwired: 11 in]
                n389 = call "settings_filename_to_registry.vi"("Last Used Settings File"=w1147) -> ()  [unwired: 11 in]
              }
            }
          }
          frame "LoadStateFromFile" {
            # "Load a file, and use it to reset the values of all the front panel controls."
            # "We need to re-run the initialisation stuff in UDP sender after changing settings\n(for example, this synchronises the settings like camera pixel size with the\nrelevant global variable)"
            n390 = call "File Dialog2"("prompt"="Please select a settings file", "button label"="Open", "default name"="red_tweezers_settings.xml", "pattern (all files)"="*.xml" ("pattern label"), "pattern label"="XML Settings Files") -> ("selected path"=w1161:path, "cancelled"=w1168:bool)  [unwired: 7 in, 2 out]
            n391 = Not(x=w1168) -> (.not. x?=w1167:bool)
            n392 = case shown="False" w1167 {
              selector: w1167 -> [w1170 w1171]
              tunnel: w1161 -> [_ w1172]
              tunnel: [w1170 w1171] -> w1159
              frame False {
              }
              frame True {
                n393 = call "settings_load_from_file.vi"("XML File Path"=w1172) -> ()  [unwired: 9 in, 2 out]
                n394 = Path To String(path=w1172) -> (string=w1173:string)
                n395 = call "settings_filename_to_registry.vi"("Last Used Settings File"=w1173) -> ()  [unwired: 11 in]
              }
            }
            n396 = call "UDP Sender generic_2.vi"("re-initialise"=w1159, "Spots"=w1160) -> ()  [unwired: 1 in, 1 out]
          }
          frame "Undo" {
            # "This should get the last undo vector and replace the spots with it :)"
            n397 = call "red_tweezers_UNDO.vi"("Selection/Group"=w1178, "Undo/Store (store, False)"=TRUE, "Spots"=w1179) -> ("Selection/Group Out (Undo only)"=w1176:T7[], "Spots Out (Undo only)"=w1177:T1[])  [unwired: 7 in]
          }
          frame "Delete" {
            n398 = call "delete_selected_spots.vi"("Selection/Group 3"=w1182, "Spots 3"=w1183) -> ("Selection/Group 2"=w1181:T7[], "Spots 2"=w1180:T1[])  [unwired: 4 in]
          }
          frame "SelectAllSpots" {
            n399 = for {
              tunnel: w1184 -> [w1189] mode=indexing
              tunnel: [w1190] -> w1185 mode=indexing
              n400 = Unbundle(w1189) -> ("Group ID"=w1188:i32)  [unwired: 1 out]
              n401 = Bundle(cluster=w1189, "Group ID"=w1188, "Selected"=TRUE ("Label.Visible")) -> (w1190:T7)
            }
          }
          frame "SelectNoSpots" {
            n402 = for {
              tunnel: w1191 -> [w1196] mode=indexing
              tunnel: [w1197] -> w1192 mode=indexing
              n403 = Unbundle(w1196) -> ("Group ID"=w1195:i32)  [unwired: 1 out]
              n404 = Bundle(cluster=w1196, "Group ID"=w1195, "Selected"=FALSE ("Label.Visible")) -> (w1197:T7)
            }
          }
          frame "SelectSpecificSpots" {
            n405 = call "select_by_id.vi"("Selection/Group"=w1199, "Spots"=w1200) -> ("Selection/Group Out"=w1198:T7[])  [unwired: 9 in]
          }
          frame "Group" {
            # "Group the currently selected spots"
            n406 = call "group_selected_spots.vi"("Selection/Group 2"=w1201) -> ("Array"=w1203:T7[])
          }
          frame "Ungroup" {
            # "Ungroup the currently selected spots"
            n407 = for {
              tunnel: [w1210] -> w1206 mode=indexing
              tunnel: w1204 -> [w1209] mode=indexing
              tunnel: 0 -> [w1208]
              n408 = Unbundle(w1209) -> ("Selected"=w1211:bool)  [unwired: 1 out]
              n409 = case shown="False" w1211 {
                tunnel: [w1212 w1215] -> w1210
                tunnel: w1209 -> [w1212 w1214]
                tunnel: w1208 -> [_ w1213]
                frame False {
                }
                frame True {
                  n410 = Unbundle(w1214) -> ("Selected"=w1216:bool)  [unwired: 1 out]
                  n411 = Bundle(cluster=w1214, "Group ID"=w1213, "Selected"=w1216) -> (w1215:T7)
                }
              }
            }
          }
          frame "ZoomIn" {
            w1217 = "ZoomToFit" ("item tag")
            # "turn off \"zoom to fit\""
            n412 = property class="ImageControl"(reference=w1232) -> (reference out=w1226:refnum<vi>, "ZoomSingle"=w1231:cluster{"X":sgl, "Y":sgl}, "Image Center Position"=w1224:cluster{"X":u32, "Y":u32})  [unwired: 1 in, 1 out]
            n413 = Unbundle(w1231) -> ("X"=w1229:sgl)  [unwired: 1 out]
            n414 = Round To Nearest(number=w1229) -> (nearest integer value=w1225:sgl)
            n415 = Greater Than 0?(x=w1225) -> (x > 0?=w1230:bool)
            n416 = case shown="True" w1230 {
              tunnel: w1229 -> [w1239 w1242]
              tunnel: [w1238 w1240] -> w1228
              frame False {
                n417 = Reciprocal(x=w1239) -> (1/x=w1236:sgl)
                n418 = Round Toward +Infinity(x=w1236) -> (ceil(x): smallest int >= x=w1237:sgl)
                n419 = Decrement(x=w1237) -> (x-1=w1235:sgl)
                n420 = Reciprocal(x=w1235) -> (1/x=w1238:sgl)
              }
              frame True {
                n421 = Round Toward -Infinity(1:w1242) -> (0:w1241:sgl)
                n422 = Increment(x=w1241) -> (x+1=w1240:sgl)
              }
            }
            n423 = Bundle(w1228, w1228) -> (w1227:cluster{sgl, sgl})  [unwired: 1 in]
            n424 = property class="ImageControl"(reference=w1226, "ZoomSingle"=w1227, "Image Center Position"=w1224) -> ()  [unwired: 1 in, 2 out]
            n425 = Get Menu Item Info(7:w1217, 11:w1223) -> (1:w1220:bool, 2:w1221:string, 3:w1222:refnum<k9>, 6:w1219:T18)  [unwired: 1 in, 3 out]
            n426 = Set Menu Item Info(4:w1219, 6:FALSE ("checked"), 7:w1217, 9:w1220, 10:w1221, 11:w1222) -> ()  [unwired: 1 in, 2 out]
          }
          frame "ZoomOut" {
            w1246 = "ZoomToFit" ("item tag")
            # "turn off \"zoom to fit\""
            n427 = property class="ImageControl"(reference=w1258) -> (reference out=w1254:refnum<vi>, "ZoomSingle"=w1257:cluster{"X":sgl, "Y":sgl}, "Image Center Position"=w1253:cluster{"X":u32, "Y":u32})  [unwired: 1 in, 1 out]
            n428 = Unbundle(w1257) -> ("X"=w1243:sgl)  [unwired: 1 out]
            n429 = Greater?(x=w1243, y=1.0) -> (0:w1245:bool)
            n430 = case shown="False" w1245 {
              tunnel: w1243 -> [w1267 w1270]
              tunnel: [w1266 w1268] -> w1256
              frame False {
                n431 = Reciprocal(x=w1267) -> (1/x=w1264:sgl)
                n432 = Add(x=w1264, y=sgl 0.01 ("x")) -> (x+y=w1262:sgl)
                n433 = Round Toward -Infinity(1:w1262) -> (0:w1265:sgl)
                n434 = Increment(x=w1265) -> (x+1=w1263:sgl)
                n435 = Reciprocal(x=w1263) -> (1/x=w1266:sgl)
              }
              frame True {
                n436 = Round Toward +Infinity(x=w1270) -> (ceil(x): smallest int >= x=w1269:sgl)
                n437 = Decrement(x=w1269) -> (x-1=w1268:sgl)
              }
            }
            n438 = Bundle(w1256, w1256) -> (w1255:cluster{sgl, sgl})  [unwired: 1 in]
            n439 = property class="ImageControl"(reference=w1254, "ZoomSingle"=w1255, "Image Center Position"=w1253) -> ()  [unwired: 1 in, 2 out]
            n440 = Get Menu Item Info(7:w1246, 11:w1252) -> (1:w1249:bool, 2:w1250:string, 3:w1251:refnum<k9>, 6:w1248:T18)  [unwired: 1 in, 3 out]
            n441 = Set Menu Item Info(4:w1248, 6:FALSE ("checked"), 7:w1246, 9:w1249, 10:w1250, 11:w1251) -> ()  [unwired: 1 in, 2 out]
          }
          frame "ZoomToFit" {
            w1276 = "ZoomToFit" ("item tag")
            # "and make sure the image obeys the result"
            # "Toggle menu checkmark"
            n442 = Get Menu Item Info(7:w1276, 11:w1275) -> (1:w1274:bool, 2:w1278:string, 3:w1279:refnum<k9>, 4:w1273:bool, 6:w1277:T18)  [unwired: 1 in, 2 out]
            n443 = Not(x=w1273) -> (.not. x?=w1271:bool)
            n444 = Set Menu Item Info(4:w1277, 6:w1271, 7:w1276, 9:w1274, 10:w1278, 11:w1279) -> ()  [unwired: 1 in, 2 out]
            n445 = property class="ImageControl"(reference=w1272, "Zoom to Fit Mode"=w1271) -> ()  [unwired: 1 in, 2 out]
          }
          frame "ShowGrid" {
            w1287 = "ShowGrid" ("item tag")
            # "Toggle menu checkmark"
            n446 = Get Menu Item Info(7:w1287, 11:w1286) -> (1:w1285:bool, 2:w1289:string, 3:w1290:refnum<k9>, 4:w1284:bool, 6:w1288:T18)  [unwired: 1 in, 2 out]
            n447 = Not(x=w1284) -> (.not. x?=w1283:bool)
            n448 = Set Menu Item Info(4:w1288, 6:w1283, 7:w1287, 9:w1285, 10:w1289, 11:w1290) -> ()  [unwired: 1 in, 2 out]
            n449 = call "grid_and_guides.vi"("Boolean"=w1283, "Operation"=T11."Set grid visibility") -> ()  [unwired: 9 in, 1 out]
          }
          frame "ShowGuides" {
            w1298 = "ShowGuides" ("item tag")
            # "Toggle menu checkmark"
            n450 = Get Menu Item Info(7:w1298, 11:w1297) -> (1:w1296:bool, 2:w1300:string, 3:w1301:refnum<k9>, 4:w1295:bool, 6:w1299:T18)  [unwired: 1 in, 2 out]
            n451 = Not(x=w1295) -> (.not. x?=w1294:bool)
            n452 = Set Menu Item Info(4:w1299, 6:w1294, 7:w1298, 9:w1296, 10:w1300, 11:w1301) -> ()  [unwired: 1 in, 2 out]
            n453 = call "grid_and_guides.vi"("Boolean"=w1294, "Operation"=T11."Set guide visibility") -> ()  [unwired: 9 in, 1 out]
          }
          frame "ConfigureGridAndGuides" {
            n454 = call "grid_and_guides.vi"("Operation"=T11."Show front panel") -> ()  [unwired: 10 in, 1 out]
          }
          frame "ShowSettings" {
            n455 = call "UDP Sender generic_2.vi"("Show panel"=TRUE, "Spots"=w1308) -> ()  [unwired: 1 in, 1 out]
          }
          frame "CameraSettings" {
            n456 = global read "red_tweezers_globals_INTERNAL_VOLATILE.vi" "Current Camera VI"() -> (w1311:path)
            n457 = Open VI Reference(vi path=w1311) -> (vi reference=w1310:refnum<vi>)  [unwired: 5 in, 1 out]
            n458 = property class="VI"(reference=w1310, "Front Panel.Open"=TRUE ("Front Panel Window:Open")) -> ()  [unwired: 1 in, 2 out]
          }
          frame Default {
          }
        }
      }
      event Mouse Down? {
        # "We don't process clicks when the user is on the video tab, so that we can set ROIs."
        # "When the mouse button goes down over the image, we save where it went down, etc. and wait to see what happens next.  We also register to be told when the mouse leaves the control, goes up, or moves.  \"click\" or \"drag\" are only detected once the mouse moves or goes up."
        n459 = event-data() -> ("Coords"=w1331:T19, "Button"=w1326:u16, "Mods"=w1335:cluster{"Double Click":bool, "Menu Key":bool}, "PlatMods"=w1334:T20)  [unwired: 1 in]
        n460 = call "mouse_to_image_coords.vi"("Mouse Coords (screen/pane units)"=w1331, "Image Control"=w1327) -> ("Cursor is on Display Area"=w1325:bool, "Mouse Coords (image pixels)"=w1330:cluster{dbl, dbl})  [unwired: 4 in]
        n461 = disable-structure shown="Enabled" {
          disable-tunnel: w1326 -> [w1343 _]
          disable-tunnel: w1325 -> [w1341 w1344]
          disable-tunnel: [w1340 w1344] -> w1321
          frame Enabled {
            n462 = Equal?(x=u16 1, y=w1343) -> (x = y?=w1342:bool)
            n463 = And(x=w1341, y=w1342) -> (x .and. y?=w1340:bool)
          }
          frame Disabled {
            # "use other pane to allow right-clicking on image"
          }
        }
        n464 = local read "Tab"() -> (w1322:T4)
        n465 = Not Equal?(x=w1322, y=T12."Video" ("Tab")) -> (x != y?=w1320:bool)
        n466 = And(x=w1321, y=w1320) -> (x .and. y?=w1319:bool)
        n467 = case shown="False" w1319 {
          tunnel: w1338 -> [w1347 w1358]
          tunnel: [T9 {"Button Down"=FALSE, "Dragging"=FALSE, "Position (Image Pixels)"={"X"=0.0, "Y"=0.0}, "Previous Position (Image Pixels)"={"X"=0.0, "Y"=0.0}, "Button"=0, "Mods"={"Double Click"=FALSE, "Menu Key"=FALSE}, "PlatMods"={"Shift"=FALSE, "Ctrl"=FALSE, "Alt"=FALSE, "Cmd"=FALSE, "Opt"=FALSE}} w1357] -> w1337
          tunnel: [w1347 w1354] -> w1336
          tunnel: w1326 -> [_ w1353]
          tunnel: w1335 -> [_ w1352]
          tunnel: w1334 -> [_ w1351]
          tunnel: w1330 -> [_ w1350]
          tunnel: [FALSE TRUE] -> w1329
          tunnel: w1327 -> [_ w1348]
          frame False {
            # "If the user clicked on a scrollbar, ignore it and let LabVIEW handle it. (this keeps the scrollbars working)"
          }
          frame True {
            w1356 = FALSE  # Dragging
            w1355 = TRUE  # Button Down
            n468 = register-events(reference=w1358, w1348, w1348, w1348, w1348) -> (reference out=w1354:refnum<event-registration>)  [unwired: 1 in, 1 out]
            n469 = Bundle("Button Down"=w1355, "Dragging"=w1356, "Mouse Coords (image pixels)"=w1350, "Mouse Coords (image pixels)"=w1350, "Button"=w1353, "Mods"=w1352, "PlatMods"=w1351) -> (w1357:T21)  [unwired: 1 in]
          }
        }
        n470 = Array Size(array=w1317) -> (size(s)=w1318:i32)
        n471 = local write "# of Spots"(w1318) -> ()
        n472 = local write "Selection/Group"(w1317) -> ()
        n473 = event-data("Discard?"=w1329) -> ()  [unwired: 4 in, 1 out]
      }
      event Mouse Leave {
        w1365 = refnum<vi> refnum  # Dummy
        # "When the mouse leaves, we reset things."
        n474 = event-data() -> ()  [unwired: 1 in, 2 out]
        n475 = register-events(reference=w1366, w1364, w1365, w1365, w1365) -> (reference out=w1363:refnum<event-registration>)  [unwired: 1 in, 1 out]
      }
      event Mouse Up {
        w1385 = refnum<vi> refnum  # Dummy
        # "Double clicking adds a spot at the mouse position."
        # "deregister"
        # "If we get here the mouse has gone down and up again.  If we've not moved in between, we have a Click.\nEither way we're no longer interested in mouse leave/move/up events."
        n476 = event-data() -> ("Mods"=w1372:cluster{"Double Click":bool, "Menu Key":bool})  [unwired: 1 in, 5 out]
        n477 = Unbundle By Name(w1378) -> ("Dragging"=w1387:bool)
        n478 = Unbundle By Name(w1372) -> ("Double Click"=w1369:bool)
        n479 = Not(x=w1387) -> (.not. x?=w1386:bool)
        n480 = Not(x=w1374) -> (.not. x?=w1376:bool)
        n481 = And(x=w1386, y=w1376) -> (x .and. y?=w1370:bool)
        n482 = case shown="True" w1370 {
          tunnel: w1378 -> [_ w1393]
          tunnel: w1380 -> [w1388 w1392]
          tunnel: w1379 -> [w1389 w1395]
          tunnel: [w1389 w1394] -> w1381
          tunnel: w1369 -> [_ w1390]
          tunnel: [w1388 w1391] -> w1371
          frame False {
          }
          frame True {
            n483 = case shown="True" w1390 {
              tunnel: w1395 -> [w1402 w1452]
              tunnel: [w1400 w1458] -> w1394
              tunnel: w1392 -> [w1396 w1459]
              tunnel: w1393 -> [w1399 w1454]
              tunnel: [w1396 w1450] -> w1391
              frame False {
                w1406 = 400.0  # 20^2 px
                # "If the user clicked, determine which spots should be selected: if we've clicked a spot/group then select it.  Shift-clicking toggles selection for that spot, and leaves the rest of the selection unchanged."
                # "check we're close enough"
                # "find closest"
                n484 = Unbundle By Name(w1399) -> ("Position (Image Pixels)"=w1398:cluster{"X":dbl, "Y":dbl}, "PlatMods.Shift"=w1397:bool)
                n485 = for {
                  tunnel: [w1442] -> w1404 mode=indexing
                  tunnel: w1398 -> [w1441]
                  tunnel: w1396 -> [w1440] mode=indexing
                  # "calculate distances between mouse position and spot positions"
                  n486 = call "extract_position.vi"("Spot"=w1440) -> ("Position"=w1439:cluster{"x":dbl, "y":dbl, "z":dbl})
                  n487 = call "coords_real_to_image_currentview.vi"("Position (real coords)"=w1439) -> ("Position (pixels, relative to the top left of the image)"=w1438:cluster{dbl, dbl})  [unwired: 7 in, 1 out]
                  n488 = Subtract(x=w1438, y=w1441) -> (x-y=w1445:cluster{dbl, dbl})
                  n489 = Multiply(x=w1445, y=w1445) -> (x*y=w1444:cluster{dbl, dbl})
                  n490 = Cluster To Array(cluster=w1444) -> (array=w1443:dbl[])
                  n491 = Add Array Elements(numeric array=w1443) -> (sum=w1442:dbl)
                }
                n492 = Array Max & Min(array=w1404) -> (min value=w1405:dbl, min index (indices)=w1401:i32)  [unwired: 2 out]
                n493 = Less Or Equal?(x=w1405, y=w1406) -> (x <= y?=w1403:bool)
                n494 = case shown="True" w1403 {
                  tunnel: w1402 -> [w1407 w1414]
                  tunnel: w1401 -> [_ w1408]
                  tunnel: w1397 -> [_ w1410]
                  tunnel: [w1407 w1409] -> w1400
                  frame False {
                    # "If we didn't click a spot, do nothing."
                  }
                  frame True {
                    # "If the spot is in a group, act on all spots in that group, not just the spot we clicked."
                    # "This case statement toggles the selection of the spot/group we clicked, and leaves other spots unchanged if we're holding shift.  Otherwise, we select the spot/group that was clicked and deselect everything else."
                    n495 = stacked-sequence {
                      tunnel: w1408 -> [_ w1416]
                      frame #0 {
                        n496 = local read "Current Spot #"() -> (→"Prev Current Spot":dbl)
                      }
                      frame #1 {
                        "Current Spot #" <- w1416
                      }
                    }
                    n497 = Index Array(array=w1414, index=w1408) -> (element=w1413:T7)
                    n498 = Unbundle(w1413) -> ("Group ID"=w1411:i32)  [unwired: 1 out]
                    n499 = Greater Than 0?(x=w1411) -> (x > 0?=w1412:bool)
                    n500 = for {
                      tunnel: w1414 -> [w1427] mode=indexing
                      tunnel: w1412 -> [w1424]
                      tunnel: w1411 -> [w1423]
                      tunnel: w1408 -> [w1422]
                      tunnel: w1410 -> [w1420]
                      tunnel: [w1418] -> w1409 mode=indexing
                      i -> [w1421]
                      n501 = Unbundle(w1427) -> ("Group ID"=w1417:i32, "Selected"=w1425:bool)
                      n502 = case shown="True" w1424 {
                        tunnel: w1417 -> [_ w1431]
                        tunnel: [w1429 w1433] -> w1419
                        tunnel: w1423 -> [_ w1432]
                        tunnel: w1422 -> [w1430 _]
                        tunnel: w1421 -> [w1428 _]
                        frame False {
                          n503 = Equal?(x=w1428, y=w1430) -> (x = y?=w1429:bool)
                        }
                        frame True {
                          n504 = Equal?(x=w1431, y=w1432) -> (x = y?=w1433:bool)
                        }
                      }
                      n505 = case shown="True" w1420 {
                        tunnel: [w1434 w1435] -> w1426
                        tunnel: w1425 -> [_ w1436]
                        tunnel: w1419 -> [w1434 w1437]
                        frame False {
                        }
                        frame True {
                          n506 = Exclusive Or(1:w1437, 2:w1436) -> (0:w1435:bool)
                        }
                      }
                      n507 = Bundle("Group ID"=w1417, w1426) -> (w1418:cluster{"Group ID":i32, bool})  [unwired: 1 out]
                    }
                  }
                }
              }
              frame True {
                # "convert mouse position to real coords, and add a spot there."
                # "Double-click detected"
                n508 = Unbundle By Name(w1454) -> ("Position (Image Pixels)"=w1453:cluster{"X":dbl, "Y":dbl})
                n509 = for {
                  tunnel: w1452 -> [w1462] mode=indexing
                  tunnel: [w1461] -> w1451 mode=indexing
                  n510 = Bundle(cluster=w1462, "Selected"=FALSE) -> (w1461:T7)  [unwired: 1 in]
                }
                n511 = call "coords_image_to_real_currentimage.vi"("Position (pixels on image)"=w1453) -> ("Position (real coords)"=w1455:cluster{dbl, dbl, "Z":dbl})  [unwired: 9 in]
                n512 = call "replace_position.vi"("Position"=w1455) -> ("Spot"=w1457:T1)  [unwired: 3 in]
                n513 = Build Array (concatenate)(w1459, w1457) -> (w1450:T1[])
                n514 = Build Array (concatenate)(w1451, T7 {"Group ID"=0, "Selected"=TRUE} ("selection_element")) -> (w1458:T7[])
                n515 = Array Size(array=w1450) -> (size(s)=w1449:i32)
                n516 = local write "Induce check"(TRUE) -> ()
                n517 = Subtract(x=w1449, y=1) -> (x-y=w1448:i32)
                n518 = local write "Current Spot #"(w1448) -> ()
              }
            }
          }
        }
        n519 = register-events(reference=w1383, w1382, w1385, w1385, w1385) -> (reference out=w1384:refnum<event-registration>)  [unwired: 1 in, 1 out]
      }
      event Mouse Move {
        n520 = event-data() -> ("Coords"=w1477:T19)  [unwired: 1 in, 2 out]
        n521 = call "mouse_to_image_coords.vi"("Mouse Coords (screen/pane units)"=w1477, "Image Control"=w1476) -> ("Mouse Coords (image pixels)"=w1468:cluster{dbl, dbl})  [unwired: 4 in, 1 out]
        n522 = Not(x=w1467) -> (.not. x?=w1472:bool)
        n523 = case shown="True" w1472 {
          tunnel: w1470 -> [_ w1490]
          tunnel: w1475 -> [w1482 w1492]
          tunnel: w1474 -> [w1481 w1491]
          tunnel: [w1481 w1491] -> w1463
          tunnel: [w1482 w1493] -> w1473
          tunnel: w1468 -> [_ w1484]
          tunnel: w1464 -> [_ w1483]
          frame False {
          }
          frame True {
            # "this is the displacement of the mouse, since the last iteration, in \"real\" coordinates (NB the conversions go before subtracting, as it may involve adding a constant as well as multiplying, which would confuse things as we're only interested in displacements here."
            # "The \"position\" local variable is there just in case we're on the \"current spot\" tab, so that the position updates nicely"
            # "If the user is dragging, translate the spots.\nHolding down shift causes the mouse's motion to be transformed into scaling about the centroid of the spots and rotation about the same point"
            n524 = Unbundle By Name(w1490) -> ("Position (Image Pixels)"=w1485:cluster{"X":dbl, "Y":dbl})
            n525 = call "find_centroid.vi"("Selection and Groups"=w1491, "Spots"=w1492) -> ("centroid"=w1486:cluster{"x":dbl, "y":dbl, "z":dbl})  [unwired: 2 in, 4 out]
            n526 = Unbundle By Name(w1490) -> ("PlatMods.Shift"=w1489:bool)
            n527 = disable-structure shown="Disabled" {
              disable-tunnel: w1486 -> [w1494 _]
              frame Disabled {
                n528 = local write "Position"(w1494) -> ()
              }
              frame Enabled {
              }
            }
            n529 = call "coords_image_to_real_currentimage.vi"("Position (pixels on image)"=w1484) -> ("Position (real coords)"=w1487:cluster{dbl, dbl, "Z":dbl})  [unwired: 9 in]
            n530 = call "coords_image_to_real_currentimage.vi"("Position (pixels on image)"=w1485) -> ("Position (real coords)"=w1488:cluster{dbl, dbl, "Z":dbl})  [unwired: 9 in]
            n531 = case shown="False" w1489 {
              tunnel: [w1499 w1773] -> w1493
              tunnel: w1492 -> [w1505 w1774]
              tunnel: w1491 -> [w1504 w1772]
              tunnel: w1488 -> [w1503 w1759]
              tunnel: w1486 -> [_ w1769]
              tunnel: w1487 -> [w1500 w1760]
              tunnel: w1483 -> [_ _]
              frame False {
                # "Spot Checker passes on information for the bubble collision,system so proper calculations can be made."
                n532 = while {
                  tunnel: w1503 -> [w1544]
                  tunnel: [w1534] -> w1501
                  tunnel: w1500 -> [w1533]
                  i -> [w1527]
                  stop <- w1529 stop-if-true
                  w1519 = 0
                  # "This while loop statement makes sure\nthat every spot gets checked before \nallowing any spot to move."
                  # "Buffer zone controls the amount of space between the\ncenter of a spot compared to the center of another spot.\nThis is used to prevent bubbles from colliding with each other."
                  # "Projected distance calculates the distance between two spots- this is used for when a \"hit\" occurs. If the projected distance becomes larger than the previous distance, the program will assume that the spot is being pulled from the buffer zone and as a result will allow the bubble to exit."
                  # "This subVI leads to the distance function, which outputs the distance between a spot being checked compared to the current spot number."
                  n533 = control-ref of="Value Check"() -> (w1524:refnum<vi>)
                  n534 = control-ref of="ID num check"() -> (w1523:refnum<vi>)
                  n535 = control-ref of="Spot Checker"() -> (w1540:refnum<vi>)
                  n536 = Subtract(x=w1533, y=w1544) -> (x-y=w1534:cluster{dbl, dbl, "Z":dbl})
                  n537 = call "DistanceFunction.vi"("Condition Driver"=FALSE, "Position (real coords)"=w1544, "Current Spot Number"=w1523, "Spot Checker"=w1540, "Spot Number Being Checked"=w1524) -> ("Distance"=w1508:dbl)  [unwired: 6 in]
                  n538 = stacked-sequence {
                    tunnel: w1508 -> [_ w1549]
                    frame #0 {
                      n539 = local read "Distance"() -> (→"Previous Distance":dbl)
                    }
                    frame #1 {
                      "Distance" <- w1549
                    }
                  }
                  n540 = Unbundle(w1534) -> (→"X Displacement":dbl, →"Y Displacement":dbl)  [unwired: 1 out]
                  n541 = control-ref of="ID num check"() -> (w1525:refnum<vi>)
                  n542 = control-ref of="Spot Checker"() -> (w1538:refnum<vi>)
                  n543 = control-ref of="Y Displacement"() -> (w1536:refnum<vi>)
                  n544 = control-ref of="Value Check"() -> (w1526:refnum<vi>)
                  n545 = control-ref of="X Displacement"() -> (w1537:refnum<vi>)
                  n546 = call "ProjectedDistance.vi"("X Displacement"=w1537, "Spot Number Check"=w1526, "Current Spot #"=w1525, "Spot Checker"=w1538, "Y Displacement"=w1536) -> ("Numeric"=→"Projected Distance":dbl)  [unwired: 6 in]
                  n547 = Multiply(x="Buffer Zone", y=2) -> (x*y=w1543:dbl)
                  n548 = local read "ID num check"() -> (w1520:dbl)
                  n549 = local read "Value Check"() -> (w1521:dbl)
                  n550 = local read "Projected Distance"() -> (w1512:dbl)
                  n551 = Equal?(x=w1508, y=0) -> (x = y?=w1509:bool)
                  n552 = case shown="False" w1509 {
                    frame False {
                      n553 = local read "Hit"() -> (w1546:bool)
                      n554 = local write "Hit Indicator"(w1546) -> ()
                    }
                    frame True {
                      "Hit Indicator" <- FALSE
                    }
                  }
                  n555 = Not Equal?(x=w1512, y=0) -> (x != y?=w1510:bool)
                  n556 = Less Or Equal?(x=w1508, y=w1543) -> (x <= y?=w1513:bool)
                  n557 = Equal?(x=w1520, y=w1519) -> (x = y?=w1518:bool)
                  n558 = And(x=w1513, y=w1510) -> (x .and. y?=w1506:bool)
                  "Hit" <- w1506
                  n559 = Equal?(x=w1519, y=w1521) -> (x = y?=w1517:bool)
                  n560 = Not(x=w1506) -> ()  [unwired: 1 out]
                  n561 = And(x=w1518, y=w1517) -> (x .and. y?=w1516:bool)
                  n562 = Or(x=w1506, y=w1516) -> (x .or. y?=w1522:bool)
                  n563 = case shown="False" w1522 {
                    frame False {
                      n564 = stacked-sequence {
                        frame #0 {
                          n565 = local read "Potential Collisions"() -> (w1552:dbl)
                          n566 = local read "Spot # Check"() -> (w1554:dbl)
                          n567 = Subtract(x=w1552, y=1) -> (x-y=w1550:dbl)
                          n568 = Less Or Equal?(x=w1554, y=w1550) -> (x <= y?=w1553:bool)
                          n569 = case shown="True" w1553 {
                            frame False {
                              # "Spot # Check resets if the the number of potential collisons is more than Spot # Check."
                              n570 = local write "Spot # Check"(0) -> ()
                            }
                            frame True {
                              n571 = stacked-sequence {
                                frame #0 {
                                # "Spot # Check increments by 1 every time it is greater than the # of potential collisions."
                                n572 = local read "Spot # Check"() -> (w1558:dbl)
                                n573 = Add(x=w1558, y=1) -> (x+y=→"Spot # Check":dbl)
                                }
                                frame #1 {
                                # "Spot # Check resets if the Spot # Check is eqaul to the # of potential collisions."
                                n574 = local read "Potential Collisions"() -> (w1559:dbl)
                                n575 = local read "Spot # Check"() -> (w1560:dbl)
                                n576 = Equal?(x=w1560, y=w1559) -> (x = y?=w1561:bool)
                                n577 = case shown="True" w1561 {
                                frame False {
                                }
                                frame True {
                                n578 = local write "Spot # Check"(0) -> ()
                                }
                                }
                                }
                                frame #2 {
                                n579 = local read "Spot Checker"() -> (w1576:T1[])
                                n580 = local read "Current Spot #"() -> (w1577:dbl)
                                n581 = local read "Area to check"() -> (w1563:dbl)
                                n582 = Index Array(array=w1576, index=w1577) -> (element=w1575:T1)
                                n583 = local read "Orig Y SC"() -> (w1572:dbl)
                                n584 = Unbundle By Name(w1575) -> ("Position.x"=w1573:dbl, "Position.y"=w1571:dbl)
                                n585 = local read "Orig X SC"() -> (w1574:dbl)
                                n586 = Subtract(x=w1571, y=w1572) -> (x-y=w1564:dbl)
                                n587 = Absolute Value(x=w1564) -> (abs(x)=w1565:dbl)
                                n588 = Subtract(x=w1573, y=w1574) -> (x-y=w1567:dbl)
                                n589 = Greater?(x=w1565, y=w1563) -> (0:w1569:bool)
                                n590 = Absolute Value(x=w1567) -> (abs(x)=w1566:dbl)
                                n591 = Greater?(x=w1566, y=w1563) -> (0:w1568:bool)
                                n592 = Or(x=w1568, y=w1569) -> (x .or. y?=w1570:bool)
                                n593 = case shown="True" w1570 {
                                frame False {
                                }
                                frame True {
                                n594 = stacked-sequence {
                                frame #0 {
                                n595 = local read "Null array"() -> (w1582:dbl[])
                                n596 = local write "What to Check"(w1582) -> ()
                                n597 = local write "ID"(w1582) -> ()
                                n598 = local read "Current Spot #"() -> (w1584:dbl)
                                n599 = local write "Potential Collisions"(0) -> ()
                                n600 = local read "Spot Checker"() -> (w1583:T1[])
                                n601 = Index Array(array=w1583, index=w1584) -> (element=w1585:T1)
                                n602 = Wait (ms)(milliseconds to wait=100) -> ()  [unwired: 1 out]
                                n603 = Unbundle By Name(w1585) -> ("Position.x"=w1579:dbl, "Position.y"=w1580:dbl)
                                n604 = local write "Orig Y SC"(w1580) -> ()
                                n605 = local write "Orig X SC"(w1579) -> ()
                                }
                                frame #1 {
                                # "All this is a  statement checking whether the microrobot is within the area being checked using absolute value statements. The number of potential collisions gets added by 1 every time a bubble is detected within the area."
                                n606 = local read "# of Spots"() -> (w1586:dbl)
                                n607 = for {
                                N: w1586 -> [_]
                                tunnel: w1586 -> [w1591]
                                i -> [w1587]
                                n608 = local read "Selection/Group"() -> (w1590:T7[])
                                n609 = Index Array(array=w1590, index=w1587) -> (element=w1589:T7)
                                n610 = Unbundle By Name(w1589) -> ("Selected"=w1588:bool)
                                n611 = case shown="True" w1588 {
                                tunnel: w1591 -> [_ w1593]
                                tunnel: w1587 -> [_ w1592]
                                frame False {
                                }
                                frame True {
                                n612 = for {
                                N: w1593 -> [_]
                                tunnel: w1592 -> [w1594]
                                i -> [w1595]
                                n613 = local read "Selection/Group"() -> (w1599:T7[])
                                n614 = Index Array(array=w1599, index=w1595) -> (element=w1598:T7)
                                n615 = Unbundle By Name(w1598) -> ("Selected"=w1596:bool)
                                n616 = Not(x=w1596) -> (.not. x?=w1597:bool)
                                n617 = case shown="True" w1597 {
                                tunnel: w1595 -> [_ w1603]
                                tunnel: w1594 -> [_ w1602]
                                tunnel: w1594 -> [_ w1601]
                                frame False {
                                }
                                frame True {
                                n618 = local read "Spot Checker"() -> (w1620:T1[])
                                n619 = Index Array(array=w1620, index=w1603) -> (element=w1621:T1)
                                n620 = Index Array(array=w1620, index=w1602) -> (element=w1619:T1)
                                n621 = Unbundle By Name(w1619) -> ("Position.x"=w1616:dbl, "Position.y"=w1612:dbl)
                                n622 = Unbundle By Name(w1621) -> ("Position.x"=w1613:dbl, "Position.y"=w1609:dbl)
                                n623 = local read "Area+ Buffer"() -> (w1600:dbl)
                                n624 = Subtract(x=w1616, y=w1600) -> (x-y=w1617:dbl)
                                n625 = Greater Or Equal?(x=w1613, y=w1617) -> (x >= y?=w1618:bool)
                                n626 = Add(x=w1612, y=w1600) -> (x+y=w1611:dbl)
                                n627 = Subtract(x=w1612, y=w1600) -> (x-y=w1610:dbl)
                                n628 = Add(x=w1616, y=w1600) -> (x+y=w1614:dbl)
                                n629 = Less Or Equal?(x=w1609, y=w1611) -> (x <= y?=w1608:bool)
                                n630 = Greater Or Equal?(x=w1609, y=w1610) -> (x >= y?=w1607:bool)
                                n631 = Less Or Equal?(x=w1613, y=w1614) -> (x <= y?=w1615:bool)
                                n632 = And(x=w1618, y=w1615) -> (x .and. y?=w1605:bool)
                                n633 = And(x=w1608, y=w1607) -> (x .and. y?=w1606:bool)
                                n634 = And(x=w1605, y=w1606) -> (x .and. y?=w1604:bool)
                                n635 = case shown="True" w1604 {
                                tunnel: w1603 -> [_ _]
                                tunnel: w1603 -> [_ w1623]
                                tunnel: w1601 -> [_ w1622]
                                frame False {
                                }
                                frame True {
                                n636 = stacked-sequence {
                                tunnel: w1623 -> [w1624 _]
                                tunnel: w1622 -> [w1625 _]
                                frame #0 {
                                n637 = local read "Potential Collisions"() -> (w1628:dbl)
                                n638 = local read "What to Check"() -> (w1629:dbl[])
                                n639 = Insert Into Array(array=w1629, index=w1628, new element=w1624) -> (w1630:dbl[])
                                n640 = local read "ID"() -> (w1627:dbl[])
                                n641 = local write "What to Check"(w1630) -> ()
                                n642 = Insert Into Array(array=w1627, index=w1628, new element=w1625) -> (w1626:dbl[])
                                n643 = local write "ID"(w1626) -> ()
                                }
                                frame #1 {
                                n644 = local read "Potential Collisions"() -> (w1633:dbl)
                                n645 = Add(x=w1633, y=1) -> (x+y=w1631:dbl)
                                n646 = local write "Potential Collisions"(w1631) -> ()
                                }
                                }
                                }
                                }
                                }
                                }
                                }
                                }
                                }
                                }
                                }
                                frame #2 {
                                n647 = local read "Current Spot #"() -> (w1634:dbl)
                                n648 = local write "Prev Current Spot"(w1634) -> ()
                                }
                                }
                                }
                                }
                                }
                              }
                            }
                          }
                        }
                        frame #1 {
                          # "This updates the ID and Value being checked at the beginning of IDs and values being checked."
                          n649 = local read "Spot # Check"() -> (w1637:dbl)
                          n650 = local read "What to Check"() -> (w1638:dbl[])
                          n651 = local read "ID"() -> (w1639:dbl[])
                          n652 = Index Array(array=w1639, index=w1637) -> (element=w1636:dbl)
                          n653 = Index Array(array=w1638, index=w1637) -> (element=w1635:dbl)
                          n654 = local write "Value Check"(w1635) -> ()
                          n655 = local write "ID num check"(w1636) -> ()
                        }
                      }
                    }
                    frame True {
                      n656 = stacked-sequence {
                        frame #0 {
                          # "This section activate a case statement which allows us to change the area being checked. Orig X/Y SC holds the position of the area to check and changes after the bubble exits the area beig checked."
                          # "This statement controls the areas selected and finds which bubbles needs to be checked. This activates when the bubble\nmoves out of the area specified."
                          n657 = local read "# of Spots"() -> (w1659:dbl)
                          n658 = local read "Current Spot #"() -> (w1658:dbl)
                          n659 = Subtract(x=w1659, y=1) -> (x-y=w1660:dbl)
                          n660 = Equal?(x=w1658, y=w1660) -> (x = y?=w1656:bool)
                          n661 = case shown="True" w1656 {
                            tunnel: [w1719 w1722] -> w1657
                            frame True {
                              n662 = local read "# of Spots"() -> (w1720:dbl)
                              n663 = Subtract(x=w1720, y=2) -> (x-y=w1719:dbl)
                            }
                            frame False {
                              n664 = local read "# of Spots"() -> (w1721:dbl)
                              n665 = Subtract(x=w1721, y=1) -> (x-y=w1722:dbl)
                            }
                          }
                          "Maximum" <- w1657
                          n666 = local read "Spot Checker"() -> (w1655:T1[])
                          n667 = local read "Current Spot #"() -> (w1654:dbl)
                          n668 = Index Array(array=w1655, index=w1654) -> (element=w1653:T1)
                          n669 = Unbundle By Name(w1653) -> ("Position.x"=w1652:dbl, "Position.y"=w1651:dbl)
                          n670 = local read "Orig Y SC"() -> (w1649:dbl)
                          n671 = local read "Orig X SC"() -> (w1650:dbl)
                          n672 = Subtract(x=w1651, y=w1649) -> (x-y=w1646:dbl)
                          n673 = Subtract(x=w1652, y=w1650) -> (x-y=w1648:dbl)
                          n674 = Absolute Value(x=w1646) -> (abs(x)=w1645:dbl)
                          n675 = Absolute Value(x=w1648) -> (abs(x)=w1647:dbl)
                          n676 = local read "Area to check"() -> (w1641:dbl)
                          n677 = local read "Area to check"() -> (w1640:dbl)
                          n678 = Greater?(x=w1647, y=w1641) -> (0:w1644:bool)
                          n679 = Greater?(x=w1645, y=w1640) -> (0:w1643:bool)
                          n680 = Or(x=w1644, y=w1643) -> (x .or. y?=w1642:bool)
                          n681 = case shown="True" w1642 {
                            frame False {
                            }
                            frame True {
                              n682 = stacked-sequence {
                                frame #0 {
                                # "A small time delay of 100 ms is provided to allow the data to pass throguh properly."
                                n683 = Wait (ms)(milliseconds to wait=100) -> ()  [unwired: 1 out]
                                n684 = local read "Null array"() -> (→"What to Check" →"ID":dbl[])
                                n685 = local read "Spot Checker"() -> (w1667:T1[])
                                n686 = local read "Current Spot #"() -> (w1666:dbl)
                                n687 = Index Array(array=w1667, index=w1666) -> (element=w1665:T1)
                                n688 = Unbundle By Name(w1665) -> ("Position.x"=→"Orig X SC":dbl, "Position.y"=→"Orig Y SC":dbl)
                                "Potential Collisions" <- 0
                                }
                                frame #1 {
                                n689 = local read "# of Spots"() -> (w1670:dbl)
                                n690 = for {
                                N: w1670 -> [_]
                                tunnel: w1670 -> [w1675]
                                i -> [w1671]
                                n691 = local read "Selection/Group"() -> (w1674:T7[])
                                n692 = Index Array(array=w1674, index=w1671) -> (element=w1673:T7)
                                n693 = Unbundle By Name(w1673) -> ("Selected"=w1672:bool)
                                n694 = case shown="True" w1672 {
                                tunnel: w1675 -> [_ w1677]
                                tunnel: w1671 -> [_ w1676]
                                frame False {
                                }
                                frame True {
                                n695 = for {
                                N: w1677 -> [_]
                                tunnel: w1676 -> [w1678]
                                i -> [w1679]
                                n696 = local read "Selection/Group"() -> (w1683:T7[])
                                n697 = Index Array(array=w1683, index=w1679) -> (element=w1682:T7)
                                n698 = Unbundle By Name(w1682) -> ("Selected"=w1680:bool)
                                n699 = Not(x=w1680) -> (.not. x?=w1681:bool)
                                n700 = case shown="True" w1681 {
                                tunnel: w1679 -> [_ w1687]
                                tunnel: w1678 -> [_ w1686]
                                tunnel: w1678 -> [_ w1685]
                                frame False {
                                }
                                frame True {
                                n701 = local read "Spot Checker"() -> (w1704:T1[])
                                n702 = Index Array(array=w1704, index=w1687) -> (element=w1705:T1)
                                n703 = Index Array(array=w1704, index=w1686) -> (element=w1703:T1)
                                n704 = Unbundle By Name(w1703) -> ("Position.x"=w1700:dbl, "Position.y"=w1696:dbl)
                                n705 = Unbundle By Name(w1705) -> ("Position.x"=w1697:dbl, "Position.y"=w1693:dbl)
                                n706 = local read "Area+ Buffer"() -> (w1684:dbl)
                                n707 = Subtract(x=w1700, y=w1684) -> (x-y=w1701:dbl)
                                n708 = Greater Or Equal?(x=w1697, y=w1701) -> (x >= y?=w1702:bool)
                                n709 = Add(x=w1696, y=w1684) -> (x+y=w1695:dbl)
                                n710 = Subtract(x=w1696, y=w1684) -> (x-y=w1694:dbl)
                                n711 = Add(x=w1700, y=w1684) -> (x+y=w1698:dbl)
                                n712 = Less Or Equal?(x=w1693, y=w1695) -> (x <= y?=w1692:bool)
                                n713 = Greater Or Equal?(x=w1693, y=w1694) -> (x >= y?=w1691:bool)
                                n714 = Less Or Equal?(x=w1697, y=w1698) -> (x <= y?=w1699:bool)
                                n715 = And(x=w1702, y=w1699) -> (x .and. y?=w1689:bool)
                                n716 = And(x=w1692, y=w1691) -> (x .and. y?=w1690:bool)
                                n717 = And(x=w1689, y=w1690) -> (x .and. y?=w1688:bool)
                                n718 = case shown="True" w1688 {
                                tunnel: w1687 -> [_ _]
                                tunnel: w1687 -> [_ w1707]
                                tunnel: w1685 -> [_ w1706]
                                frame False {
                                }
                                frame True {
                                n719 = stacked-sequence {
                                tunnel: w1707 -> [w1708 _]
                                tunnel: w1706 -> [w1709 _]
                                frame #0 {
                                n720 = local read "Potential Collisions"() -> (w1712:dbl)
                                n721 = local read "What to Check"() -> (w1713:dbl[])
                                n722 = Insert Into Array(array=w1713, index=w1712, new element=w1708) -> (w1714:dbl[])
                                n723 = local read "ID"() -> (w1711:dbl[])
                                n724 = Insert Into Array(array=w1711, index=w1712, new element=w1709) -> (w1710:dbl[])
                                n725 = local write "What to Check"(w1714) -> ()
                                n726 = local write "ID"(w1710) -> ()
                                }
                                frame #1 {
                                n727 = local read "Potential Collisions"() -> (w1717:dbl)
                                n728 = Add(x=w1717, y=1) -> (x+y=w1715:dbl)
                                n729 = local write "Potential Collisions"(w1715) -> ()
                                }
                                }
                                }
                                }
                                }
                                }
                                }
                                }
                                }
                                }
                                }
                              }
                            }
                          }
                        }
                        frame #1 {
                          n730 = local read "# of Spots"() -> (w1726:dbl)
                          n731 = Not Equal?(x=w1726, y=1) -> (x != y?=w1724:bool)
                          n732 = case shown="True" w1724 {
                            frame False {
                            }
                            frame True {
                              n733 = stacked-sequence {
                                frame #0 {
                                n734 = local read "Potential Collisions"() -> (w1729:dbl)
                                n735 = local read "Spot # Check"() -> (w1731:dbl)
                                n736 = Subtract(x=w1729, y=1) -> (x-y=w1727:dbl)
                                n737 = Less Or Equal?(x=w1731, y=w1727) -> (x <= y?=w1730:bool)
                                n738 = case shown="False" w1730 {
                                frame False {
                                n739 = local write "Spot # Check"(0) -> ()
                                }
                                frame True {
                                }
                                }
                                }
                                frame #1 {
                                n740 = local read "What to Check"() -> (w1737:dbl[])
                                n741 = local read "ID"() -> (w1735:dbl[])
                                n742 = local read "Spot # Check"() -> (w1733:dbl)
                                n743 = Index Array(array=w1737, index=w1733) -> (element=→"Value Check":dbl)
                                n744 = Index Array(array=w1735, index=w1733) -> (element=→"ID num check":dbl)
                                }
                              }
                            }
                          }
                        }
                      }
                    }
                  }
                  n745 = local read "Potential Collisions"() -> (w1514:dbl)
                  n746 = Subtract(x=w1514, y=1) -> (x-y=w1515:dbl)
                  n747 = local read "Hit"() -> (w1532:bool)
                  n748 = Equal?(x=w1527, y=w1515) -> (x = y?=w1531:bool)
                  n749 = Or(x=w1532, y=w1531) -> (x .or. y?=w1529:bool)
                }
                n750 = for {
                  tunnel: w1504 -> [w1751] mode=indexing
                  tunnel: w1505 -> [w1748] mode=indexing
                  tunnel: [w1750] -> w1499 mode=indexing
                  tunnel: w1501 -> [w1749]
                  # "If the projected distance is greater than the\nprevious distance, then the selected spots will move. \nThis situation only occurs if the bubble is about to/crossing \nthe buffer zone of another bubble. \n\nThe selected spots will also move if none of the bubbles\nare near/crossing the buffer zone of another bubble."
                  n751 = local read "Hit"() -> (w1741:bool)
                  n752 = Unbundle By Name(w1748) -> ()  [unwired: 1 out]
                  n753 = local read "Projected Distance"() -> (w1740:dbl)
                  n754 = Unbundle(w1751) -> ("Group ID"=→"Group ID #":i32, "Selected"=w1745:bool)
                  n755 = local read "Previous Distance"() -> (w1743:dbl)
                  n756 = Not(x=w1741) -> (.not. x?=w1739:bool)
                  n757 = Greater?(x=w1740, y=w1743) -> (0:w1742:bool)
                  n758 = And(x=w1741, y=w1742) -> (x .and. y?=w1738:bool)
                  n759 = Or(x=w1739, y=w1738) -> (x .or. y?=w1744:bool)
                  n760 = And(x=w1745, y=w1744) -> (x .and. y?=w1746:bool)
                  n761 = case shown="True" w1746 {
                    tunnel: w1748 -> [w1752 w1756]
                    tunnel: [w1752 w1755] -> w1750
                    tunnel: w1749 -> [_ w1757]
                    frame False {
                      # "otherwise, leave it alone!"
                    }
                    frame True {
                      # "If the spot is selected, move it by the same amount as the mouse"
                      n762 = call "extract_position.vi"("Spot"=w1756) -> ("Position"=w1754:cluster{"x":dbl, "y":dbl, "z":dbl})
                      n763 = Add(x=w1754, y=w1757) -> (x+y=w1753:cluster{dbl, dbl, dbl})
                      n764 = call "replace_position.vi"("Position"=w1753, "Spot in"=w1756) -> ("Spot"=w1755:T1)  [unwired: 2 out]
                    }
                  }
                }
                "Spot Checker" <- w1499
                n765 = local read "Locked Current Spot"() -> (w1495:dbl)
                n766 = Index Array(array=w1499, index=w1495) -> (element=w1498:T1)
                n767 = Unbundle By Name(w1498) -> ("Position.x"=→"New X":dbl, "Position.y"=→"New Y":dbl)  [unwired: 1 out]
                n768 = Array Size(array=w1499) -> (size(s)=→"# of Spots":i32)
              }
              frame True {
                # "coordinate conversion to find the rotation and scaling done by the mouse, about the centroid of the spots"
                n769 = Subtract(x=w1759, y=w1769) -> (x-y=w1778:cluster{dbl, dbl, dbl})
                n770 = Subtract(x=w1760, y=w1769) -> (x-y=w1777:cluster{dbl, dbl, dbl})
                n771 = Unbundle(w1777) -> (w1763:dbl, w1764:dbl)  [unwired: 1 out]
                n772 = Unbundle(w1778) -> (w1768:dbl, w1767:dbl)  [unwired: 1 out]
                n773 = Re/Im To Polar(2:w1764, 3:w1763) -> (0:w1761:dbl, 1:w1762:dbl)
                n774 = Re/Im To Polar(2:w1767, 3:w1768) -> (0:w1765:dbl, 1:w1766:dbl)
                n775 = Divide(x=w1762, y=w1766) -> (x/y=w1758:dbl)
                n776 = Subtract(x=w1761, y=w1765) -> (x-y=w1770:dbl)
                n777 = Bundle(w1758, w1758, w1758) -> (w1780:cluster{dbl, dbl, dbl})  [unwired: 1 out]
                n778 = call "scale_matrix.vi"("Scale Factors"=w1780) -> ("Scale Matrix"=w1776:T15)
                n779 = call "arb_rotation_matrix.vi"("Unit Vector"=cluster{dbl, dbl, dbl} {0.0, 0.0, 1.0}, "theta"=w1770) -> ("Real Matrix"=w1775:T15)
                n780 = call-poly <vilib>:"A x B.vi"("B"=w1775, "A"=w1776) -> ("A x B"=w1771:T15)  [unwired: 1 out]
                n781 = for {
                  tunnel: w1774 -> [w1786] mode=indexing
                  tunnel: [w1785] -> w1773 mode=indexing
                  tunnel: w1772 -> [w1784] mode=indexing
                  tunnel: w1769 -> [w1782]
                  tunnel: w1771 -> [w1781]
                  n782 = Unbundle(w1784) -> ("Selected"=w1783:bool)  [unwired: 1 out]
                  n783 = case shown="True" w1783 {
                    tunnel: w1786 -> [w1787 w1791]
                    tunnel: [w1787 w1790] -> w1785
                    tunnel: w1782 -> [_ w1789]
                    tunnel: w1781 -> [_ w1788]
                    frame False {
                    }
                    frame True {
                      n784 = call "apply_matrix_transformation_to_spots.vi"("Transform centre (i.e. transform about this point)"=w1789, "Transformation Matrix (3x3)"=w1788, "Spot In"=w1791) -> ("Spot Out"=w1790:T1)  [unwired: 5 out]
                    }
                  }
                }
              }
            }
          }
        }
        "Selection/Group" <- w1463
        n785 = Unbundle By Name(w1470) -> ("Position (Image Pixels)"=w1469:cluster{"X":dbl, "Y":dbl})
        n786 = Bundle By Name(cluster=w1470, "Dragging"=TRUE, "Previous Position (Image Pixels)"=w1469, "Position (Image Pixels)"=w1468) -> (w1479:T9)
      }
      event "stop": Value Change {
        n787 = event-data() -> ()  [unwired: 1 in, 4 out]
        n788 = global read "red_tweezers_globals_INTERNAL_VOLATILE.vi" "Current Settings File"() -> (w1795:path)
        n789 = call <vilib>:"Check if File or Folder Exists.vi"("path"=w1795) -> ("file or folder exists?"=w1794:bool)  [unwired: 8 in, 2 out]
        n790 = case shown="False" w1794 {
          tunnel: [w1802 w1806] -> w1796
          frame False {
            n791 = Two Button Dialog(message="Save current settings?", 1:"Don't Save" ("F button name (\"Cancel\")"), 2:"Save As..." ("T button name (\"OK\")")) -> (T button?=w1799:bool)
            n792 = Select(t=T13."Center Button" ("Which Button?"), s=w1799, f=T13."Right Button" ("Which Button?")) -> (s? t:f=w1802:T13)
          }
          frame True {
            n793 = call <vilib>:"Three Button Dialog.vi"("Allow user to close window? (TRUE)"=TRUE, "Window Title (\"\")"="Save Settings?" ("Window Title (\"\")"), "Right Button Text (\"Cancel\")"="No" ("Right Button Text (\"Cancel\")"), "Center Button Text (\"No\")"="Save As..." ("Center Button Text (\"No\")"), "Left Button Text (\"Yes\")"="Save" ("Left Button Text (\"Yes\")"), "message"="Would you like to save the current settings? You can choose to use the current settings file or save to a new location.") -> ("Which Button?"=w1806:T13)  [unwired: 5 in]
          }
        }
        n794 = case shown="\"Center Button\"" w1796 {
          tunnel: [TRUE TRUE FALSE FALSE] -> w1793
          frame "Left Button", Default {
          }
          frame "Center Button" {
            n795 = call "File Dialog5"("prompt"="Please select a location to save the settings", "button label"="Save", "default name"="red_tweezers_settings.xml", "pattern (all files)"="*.xml" ("pattern label"), "pattern label"="XML Settings Files") -> ("selected path"=w1814:path)  [unwired: 7 in, 3 out]
            n796 = global write "red_tweezers_globals_INTERNAL_VOLATILE.vi" "Current Settings File"(w1814) -> ()
          }
          frame "Right Button" {
          }
          frame "Window Close" {
          }
        }
        n797 = global write "red_tweezers_globals_INTERNAL_VOLATILE.vi" "Save Settings On Exit"(w1793) -> ()
      }
    }
    n798 = local read "Stop"() -> (w33:i32)
    n799 = local read "Start"() -> (w32:i32)
    n800 = Subtract(x=w33, y=w32) -> (x-y=→"Time Elapsed(ms)":i32)
    n801 = case shown="True" "Play" {
      frame False {
      }
      frame True {
        n802 = stacked-sequence {
          frame #0 {
            n803 = Tick Count (ms)() -> (millisecond timer value=→"Start":u32)
          }
          frame #1 {
            # "Activate the MATLAB code\n\nObtain data"
            n804 = script code="%cd ('C:\\Users\\WENQI\\Desktop\\Research\\Current Red Tweezers\\Closed Loop Control\\05')\n%load('22-Jul-2016 16-05-17HoughRslt.mat')\nNumberofPlannedFrames = 30;\n%MaxNumberOfBubbles = 1;\n%Initiate = 1;\n%LockCurrentSpot = 1;\nNewXYmatrix = [\n-7.488E-5 5.0E-5;\n];\n%BubbleNewX = 0.000819;\n%BubbleNewY = 0.000131;\n%BubbleNewX = 0.00116;\n%BubbleNewY = 0.000776;\n%BubbleNewX = 0.001495;\n%BubbleNewY = 0.000374;\n%BubbleNewX = location(1,1)*10^-6;\n%BubbleNewY = location(1,2) * 10^-6;\n%Rates = 1;\n%Insert = 1;\n\n % Variable( for LabVIEW)\nMaxNumberOfBubbles = 1;\nInitiate = 1;\nLockCurrentSpot= 0;\nRates = 0;\n%Insert = 1;\n\n% Loacal variable\nFrameSize = 30;%[um]"() -> ("??"=→"error out":errorcluster, "MaxNumberOfBubbles"=→"Max Number of Bubbles 2":dbl, "Initiate"=→"Initiate Creation 2":dbl, "NumberofPlannedFrames"=w272:dbl, "LockCurrentSpot"=→"LCS":dbl, "Rates"=→"Rates":dbl, "NewXYmatrix"=→"NewXYArray":dbl[][])  [unwired: 1 in]
            "Number of Planned Sequence Frames 2" <- w272
            n805 = local write "How Many Frames?"(w272) -> ()
          }
          frame #2 {
            n806 = local read "NewXYArray"() -> (w279:dbl[][])
            n807 = Array Size(array=w279) -> (size(s)=w278:i32[])
            n808 = Index Array(array=w278, index=0) -> (element=w276:i32)
            "NewXYArraySize" <- w276
            n809 = for {
              N: w276 -> [w281]
              i -> [w282]
              stop <- w280 stop-if-true
              n810 = stacked-sequence {
                tunnel: w282 -> [w284 _]
                tunnel: w281 -> [w283 _]
                tunnel: [_ w287] -> w280
                frame #0 {
                  n811 = local write "Locked Current Spot"(w284) -> ()
                  n812 = local write "# of Spots"(w283) -> ()
                  n813 = local write "Rates"(1) -> ()
                  n814 = local write "LCS"(0) -> ()
                }
                frame #1 {
                  n815 = local read "Insert"() -> (w287:bool)
                  n816 = local write "Insert"(TRUE) -> ()
                }
              }
            }
          }
        }
      }
    }
    n817 = case shown="True" "Lock Current Spot" {
      frame False {
      }
      frame True {
        n818 = global read "red_tweezers_globals.vi" "Spots"() -> (w366:T1[])
        n819 = local read "Current Spot #"() -> (w367:dbl)
        "Locked Current Spot" <- w367
        n820 = Index Array(array=w366, index=w367) -> (element=w368:T1)
        n821 = Unbundle By Name(w368) -> ("Position.x"=→"LCS X":dbl, "Position.y"=→"LCS Y":dbl)
        n822 = local write "LCS"(0) -> ()
      }
    }
    n823 = local read "Rates"() -> (w38:dbl)
    n824 = Equal?(x=w38, y=1.0) -> (x = y?=w36:bool)
    n825 = case shown="True" w36 {
      frame False {
      }
      frame True {
        n826 = stacked-sequence {
          frame #0 {
            n827 = local read "Number of Planned Sequence Frames 2"() -> (w217:dbl)
            n828 = local read "Tab Control"() -> (w218:enum32{"Line", "Arc"})
            n829 = case shown="\"Line\"" w218 {
              tunnel: w217 -> [w219 w238]
              frame "Arc" {
                n830 = stacked-sequence {
                  tunnel: w219 -> [_ w232 _]
                  frame #0 {
                    n831 = expression code="(x/180.0)*pi" "degrees to radians"("Theta") -> (→"Radians":dbl)
                    n832 = local read "Radians"() -> (w231:dbl)
                    n833 = local read "Original Y"() -> (w225:dbl)
                    n834 = local read "Original X"() -> (w223:dbl)
                    n835 = Cosine(x=w231) -> (cos(x)=w220:dbl)
                    n836 = Sine(x=w231) -> (sin(x)=w222:dbl)
                    n837 = Multiply(x=w220, y="Radius X") -> (x*y=w224:dbl)
                    n838 = Multiply(x="Radius X", y=w222) -> (x*y=w226:dbl)
                    n839 = Subtract(x=w223, y=w224) -> (x-y=→"Center X":dbl)
                    n840 = Subtract(x=w225, y=w226) -> (x-y=→"Center Y":dbl)
                  }
                  frame #1 {
                    n841 = local read "Radians"() -> (w236:dbl)
                    n842 = Subtract(x=w232, y=1) -> (x-y=w234:dbl)
                    n843 = Divide(x=w236, y=w234) -> (x/y=→"Degree Rate":dbl)
                  }
                  frame #2 {
                  }
                }
              }
              frame "Line" {
                n844 = local read "Max Number of Bubbles 2"() -> (w237:dbl)
                n845 = for {
                  N: w237 -> [_]
                  tunnel: w238 -> [w240]
                  i -> [w239]
                  n846 = stacked-sequence {
                    tunnel: w240 -> [_ w258]
                    tunnel: w239 -> [w244 w255]
                    frame #0 {
                      n847 = local read "NewXYArray"() -> (w250:dbl[][])
                      n848 = Index Array(array=w250, index (row)=w244) -> (element=w249:dbl[])  [unwired: 1 in]
                      n849 = Array To Cluster(array=w249) -> (cluster=w248:T22)
                      n850 = global read "red_tweezers_globals.vi" "Spots"() -> (w245:T1[])
                      n851 = Unbundle By Name(w248) -> ("NewXYArray[0]"=w247:dbl, "NewXYArray[1]"=w246:dbl)
                      n852 = Index Array(array=w245, index=w244) -> (element=w243:T1)
                      n853 = local write "New Y"(w246) -> ()
                      n854 = local write "New X"(w247) -> ()
                      n855 = Unbundle By Name(w243) -> ("Position.x"=w242:dbl, "Position.y"=w241:dbl)
                      n856 = local write "Original X"(w242) -> ()
                      n857 = local write "Original Y"(w241) -> ()
                    }
                    frame #1 {
                      n858 = local read "Original X"() -> (w259:dbl)
                      n859 = local read "Original Y"() -> (w261:dbl)
                      n860 = Subtract(x=w258, y=1) -> (x-y=w265:dbl)
                      n861 = local read "New Y"() -> (w262:dbl)
                      n862 = local read "New X"() -> (w260:dbl)
                      n863 = Subtract(x=w261, y=w262) -> (x-y=w264:dbl)
                      n864 = Subtract(x=w259, y=w260) -> (x-y=w263:dbl)
                      n865 = Divide(x=w264, y=w265) -> (x/y=w253:dbl)
                      "Y Rate" <- w253
                      n866 = Divide(x=w263, y=w265) -> (x/y=w254:dbl)
                      "X Rate" <- w254
                      n867 = Bundle(w254, w253) -> (w252:cluster{dbl, dbl})  [unwired: 1 in]
                      n868 = local read "NewXYRates"() -> (w256:dbl[][])
                      n869 = Cluster To Array(cluster=w252) -> (array=w251:dbl[])
                      n870 = Insert Into Array(array=w256, index (row)=w255, new element=w251) -> (w257:dbl[][])  [unwired: 1 in]
                      n871 = local write "NewXYRates"(w257) -> ()
                    }
                  }
                }
              }
            }
          }
          frame #1 {
            n872 = local write "Rates"(0) -> ()
          }
        }
      }
    }
    n873 = case shown="True" "Mark Original Position" {
      frame False {
      }
      frame True {
        w369 = TRUE
        n874 = local write "Mark Original Position"(FALSE) -> ()
        n875 = local read "New X"() -> (→"Original X":dbl)
        n876 = local read "New Y"() -> (→"Original Y":dbl)
        "MOP pressed After" <- w369
        "MOP pressed" <- w369
      }
    }
    n877 = local read "Sequence Instances"() -> (w94:dbl)
    n878 = case shown="True" w113 {
      tunnel: w119 -> [_ w435]
      frame False {
      }
      frame True {
        n879 = global write "red_tweezers_globals_INTERNAL.vi" "Image Overlay (extras from control loop)"(w435) -> ()
      }
    }
    n880 = local read "Counter"() -> (w93:dbl)
    n881 = call "red_tweezers_UNDO.vi"("Force Save"=w115, "This change is inconsequential (don't save it)"=w116, "Selection/Group"=w117, "Spots"=w118) -> ()  [unwired: 6 in, 2 out]
    n882 = call "sync_with_globals.vi"("Selection/Group"=w117, "Spots"=w118) -> ("Selection/Group 2"=w129:T7[], "Spots 2"=w80:T1[])  [unwired: 4 in]
    n883 = local read "Sequence Storer"() -> (w89:T1[][])
    n884 = local read "Sequence On?"() -> (w92:bool)
    n885 = local read "Sequence On?"() -> (w107:bool)
    n886 = call "SequenceControl.vi"("Sequence On? 2"=w92, "Counter 2"=w93, "Sequence Instances 2"=w94, "Sequence Storer"=w89) -> ("Time per Frame (ms) 2"=w87:dbl, "Sequence Order 2"=w90:dbl, "Reset 2"=w91:bool, "Sequence Storer 2"=w102:T1[][], "Clearance Button 2"=w101:bool, "Manual Edit 2"=w100:bool, "Save State 2"=w99:bool, "Play Sequence 2"=w96:bool, "Bubble ID to Empty 2"=w95:dbl, "Manual Sequence 2"=w97:bool, "Edit Sequence Mode 2"=w98:bool)  [unwired: 1 in]
    n887 = local write "Play Sequence"(w96) -> ()
    n888 = local write "Bubble ID to Empty"(w95) -> ()
    n889 = local write "Manual Sequence"(w97) -> ()
    n890 = local write "Reset"(w91) -> ()
    n891 = local write "Edit Sequence Mode"(w98) -> ()
    n892 = local write "Clearance Button"(w101) -> ()
    n893 = local write "Sequence Storer"(w102) -> ()
    n894 = local write "Save State"(w99) -> ()
    n895 = local write "Manual Edit"(w100) -> ()
    n896 = Or(x=w107, y="Manual Sequence") -> (x .or. y?=w106:bool)
    n897 = local write "Time per Frame (ms)"(w87) -> ()
    n898 = feedback #10() -> (w134:T23)  [unwired: 1 out]
    n899 = call "Smoothed Frame Rate.vi"("Feedback In"=w134) -> ("Feedback Out"=w133:T23, "Frame Rate"=→"Interface Frame Rate":dbl)  [unwired: 1 in, 4 out]
    n900 = feedback-in #10(w133) -> ()
    n901 = local write "Sequence Order"(w90) -> ()
    n902 = Not(x=w83) -> (.not. x?=w84:bool)
    n903 = Not(x="Output to SLM") -> (.not. x?=w85:bool)
    n904 = case shown="True" w106 {
      tunnel: [w405 w410] -> w110
      tunnel: w80 -> [w404 _]
      frame False {
        n905 = Or(x="Manual Edit", y="Edit Sequence Mode") -> (x .or. y?=w403:bool)
        n906 = case shown="False" w403 {
          tunnel: w404 -> [w406 _]
          tunnel: [w406 w407] -> w405
          frame False {
          }
          frame True {
            n907 = local read "Sequence Order"() -> (w408:dbl)
            n908 = local read "Sequence Storer"() -> (w409:T1[][])
            n909 = Index Array(array=w409, index (row)=w408) -> (element=w407:T1[])  [unwired: 1 in]
          }
        }
      }
      frame True {
        n910 = stacked-sequence {
          tunnel: [w412 _] -> w410
          frame #0 {
            n911 = local read "Counter"() -> (w413:dbl)
            n912 = local read "Sequence Storer"() -> (w414:T1[][])
            n913 = Index Array(array=w414, index (row)=w413) -> (element=w412:T1[])  [unwired: 1 in]
            n914 = Wait (ms)(milliseconds to wait="Time per Frame (ms)") -> ()  [unwired: 1 out]
          }
          frame #1 {
            n915 = local read "Sequence Instances"() -> (w416:dbl)
            n916 = local read "Counter"() -> (w419:dbl)
            n917 = Subtract(x=w416, y=1) -> (x-y=w417:dbl)
            n918 = Equal?(x=w419, y=w417) -> (x = y?=w418:bool)
            n919 = case shown="True" w418 {
              frame False {
                n920 = local read "Counter"() -> (w422:dbl)
                n921 = Add(x=w422, y=1) -> (x+y=→"Counter":dbl)
              }
              frame True {
                w423 = FALSE
                n922 = local write "Counter"(0) -> ()
                n923 = local write "Play Sequence"(w423) -> ()
                n924 = local write "Sequence On?"(w423) -> ()
              }
            }
          }
        }
      }
    }
    n925 = case shown="True" "Save State" {
      tunnel: w80 -> [_ w426]
      frame False {
      }
      frame True {
        n926 = local write "Save State"(FALSE) -> ()
        n927 = stacked-sequence {
          tunnel: w426 -> [w427 _]
          frame #0 {
            "Spot Storage" <- w427
          }
          frame #1 {
            n928 = local read "Spot Storage"() -> (w433:T1[])
            n929 = Replace Array Subset(array="Sequence Storer", new element=w433, index (row)="Sequence Order") -> (w431:T1[][])  [unwired: 1 in]
            n930 = Array Size(array=w431) -> (size(s)=w430:i32[])
            n931 = local write "Sequence Storer"(w431) -> ()
            n932 = Index Array(array=w430, index=0) -> (element=→"Sequence Instances":i32)
          }
        }
      }
    }
    n933 = case shown="True" "Clearance Button" {
      frame False {
      }
      frame True {
        # "This is the Bubble ID to Empty tool- this \"deletes\" the bubble in a sequence."
        n934 = local read "Sequence Order"() -> (w396:dbl)
        n935 = local read "Sequence Storer"() -> (w397:T1[][])
        n936 = Replace Array Subset(array=w397, new element=T10 {"Position"={"x"=nan, "y"=nan, "z"=nan}, "Intensity"=1.0, "Vortex Charge"=1, "Phase"=1.0, "NA Position"={"x"=0.0, "y"=0.0, "r"=1.0}, "Line Trapping"={"Vector"={"x"=0.0, "y"=0.0, "z"=0.0}, "Phase Gradient"=0.0}, "Amplitude Correction"=0.0} ("Cluster"), index (row)=w396, index (col)="Bubble ID to Empty") -> (w393:T1[][])
        n937 = local write "Sequence Storer"(w393) -> ()
      }
    }
    n938 = case shown="True" "Save" {
      frame False {
      }
      frame True {
        n939 = local read "Sequence Storer"() -> (w362:T1[][])
        n940 = call "SequenceSaver.vi"("Sequence Storer"=w362) -> ()  [unwired: 10 in, 1 out]
      }
    }
    n941 = And(x=w85, y=w84) -> (x .and. y?=w88:bool)
    n942 = case shown="True" "Load" {
      frame False {
      }
      frame True {
        n943 = call "SequenceSaver.vi"() -> ("Sequence Storer 2"=w361:T1[][])  [unwired: 11 in]
        n944 = local write "Sequence Storer"(w361) -> ()
      }
    }
    n945 = local read "Initiate Creation 2"() -> (w41:dbl)
    n946 = case shown="True" w88 {
      tunnel: w80 -> [w1823 _]
      frame False {
        n947 = call "UDP Sender generic_2.vi"("Spots"=w1823) -> ()  [unwired: 2 in, 1 out]
      }
      frame True {
      }
    }
    n948 = case shown="True" "Reset" {
      frame False {
      }
      frame True {
        n949 = local write "Counter"(0) -> ()
      }
    }
    n950 = case shown="True" "Add Additional Frames" {
      frame False {
      }
      frame True {
        # "This adds additional frames to the sequence."
        n951 = for {
          N: "Additional Frames Wanted" -> [_]
          i -> [w375]
          n952 = local read "Max Number of Bubbles 2"() -> (w379:dbl)
          n953 = Add(x=1, y=w375) -> (x+y=w376:i32)
          n954 = Add(x="Frame Location", y=w376) -> (x+y=w377:dbl)
          n955 = Initialize Array(T10 {"Position"={"x"=nan, "y"=nan, "z"=nan}, "Intensity"=1.0, "Vortex Charge"=1, "Phase"=1.0, "NA Position"={"x"=0.0, "y"=0.0, "r"=1.0}, "Line Trapping"={"Vector"={"x"=0.0, "y"=0.0, "z"=0.0}, "Phase Gradient"=0.0}, "Amplitude Correction"=0.0} ("Cluster"), w379) -> (w380:T24)
          n956 = local read "Sequence Storer"() -> (w381:T1[][])
          n957 = Insert Into Array(array=w381, index (row)=w377, new element=w380) -> (w382:T1[][])  [unwired: 1 in]
          n958 = local write "Sequence Storer"(w382) -> ()
        }
      }
    }
    n959 = case shown="1" w41 {
      frame 0, Default {
      }
      frame 1 {
        # "This create the array needed for a sequential\narray."
        n960 = local read "Number of Planned Sequence Frames 2"() -> (w386:dbl)
        n961 = local read "Max Number of Bubbles 2"() -> (w385:dbl)
        n962 = for {
          N: w386 -> [_]
          tunnel: w385 -> [w387]
          i -> [w390]
          n963 = Initialize Array(T10 {"Position"={"x"=nan, "y"=nan, "z"=nan}, "Intensity"=1.0, "Vortex Charge"=1, "Phase"=1.0, "NA Position"={"x"=0.0, "y"=0.0, "r"=1.0}, "Line Trapping"={"Vector"={"x"=0.0, "y"=0.0, "z"=0.0}, "Phase Gradient"=0.0}, "Amplitude Correction"=0.0} ("Cluster"), w387) -> (w388:T24)
          n964 = local read "Sequence Storer"() -> (w391:T1[][])
          n965 = Insert Into Array(array=w391, index (row)=w390, new element=w388) -> (w392:T1[][])  [unwired: 1 in]
          n966 = local write "Sequence Storer"(w392) -> ()
        }
        n967 = local write "Initiate Creation 2"(0) -> ()
      }
    }
    n968 = case shown="False" "Play Sequence" {
      frame False {
        n969 = local write "Sequence On?"(FALSE) -> ()
      }
      frame True {
        "Sequence On?" <- TRUE
      }
    }
    n970 = local read "Current Spot #"() -> (w63:dbl)
    n971 = local read "Selection/Group"() -> (w64:T7[])
    n972 = local read "# of Spots"() -> (w79:dbl)
    n973 = Not Equal?(x=w63, y=-1) -> (x != y?=w65:bool)
    n974 = local read "spots selected 2"() -> (w53:i32)
    n975 = Index Array(array=w64, index=w63) -> (element=w62:T7)
    n976 = Unbundle By Name(w62) -> ("Selected"=w61:bool)
    n977 = local read "spots selected"() -> (w54:i32)
    n978 = Not(x=w61) -> (.not. x?=w60:bool)
    n979 = And(x=w60, y=w65) -> (x .and. y?=w55:bool)
    n980 = Less?(x=w54, y=w53) -> (x < y?=w51:bool)
    n981 = case shown="True" "Insert" {
      tunnel: w80 -> [_ w137]
      tunnel: w79 -> [_ w136]
      frame False {
      }
      frame True {
        n982 = for {
          N: w136 -> [_]
          tunnel: w137 -> [w139]
          i -> [w138]
          n983 = stacked-sequence {
            tunnel: w139 -> [w141 w146 _]
            tunnel: w138 -> [_ w142 _]
            frame #0 {
              n984 = local read "Start at Which Frame?"() -> (→"Num":dbl)
              "Spot Storage 2" <- w141
            }
            frame #1 {
              n985 = local read "Selection/Group"() -> (w145:T7[])
              n986 = Index Array(array=w145, index=w142) -> (element=w144:T7)
              n987 = Unbundle By Name(w144) -> ("Selected"=w143:bool)
              n988 = case shown="True" w143 {
                tunnel: w146 -> [_ _]
                frame False {
                }
                frame True {
                  n989 = stacked-sequence {
                    frame #0 {
                      n990 = case shown="\"Arc\"" "Tab Control" {
                        frame "Arc" {
                          n991 = local read "How Many Frames?"() -> (w150:dbl)
                          n992 = Subtract(x=w150, y=1) -> (x-y=w148:dbl)
                          n993 = for {
                            N: w150 -> [_]
                            tunnel: w148 -> [w151]
                            i -> [w153]
                            # "What is this ^\n\nFor # of sequence\nframes, don't worry\nabout it"
                            # "How to make position x and y?\nIt's called a cluster, inser the new position to Position.x and Position.y"
                            n994 = Equal?(x=w151, y=w153) -> (x = y?=w152:bool)
                            n995 = case shown="True" w152 {
                              tunnel: [w176 w185] -> w155
                              tunnel: [w175 w184] -> w154
                              tunnel: w153 -> [w172 _]
                              frame False {
                                # "calculating new position"
                                n996 = local read "Degree Rate"() -> (w174:dbl)
                                n997 = Multiply(x=w174, y=w172) -> (x*y=w173:dbl)
                                n998 = Cosine(x=w173) -> (cos(x)=w182:dbl)
                                n999 = Sine(x=w173) -> (sin(x)=w183:dbl)
                                n1000 = local read "Radius X"() -> (w181:dbl)
                                n1001 = Multiply(x=w181, y=w183) -> (x*y=w180:dbl)
                                n1002 = Multiply(x=w182, y=w181) -> (x*y=w179:dbl)
                                n1003 = local read "Center X"() -> (w178:dbl)
                                n1004 = local read "Center Y"() -> (w177:dbl)
                                n1005 = Add(x=w178, y=w179) -> (x+y=w176:dbl)
                                n1006 = Add(x=w177, y=w180) -> (x+y=w175:dbl)
                              }
                              frame True {
                                n1007 = global read "red_tweezers_globals.vi" "Spots"() -> (w188:T1[])
                                n1008 = local read "Numeric"() -> (w187:dbl)
                                n1009 = Index Array(array=w188, index=w187) -> (element=w186:T1)
                                n1010 = Unbundle By Name(w186) -> ("Position.x"=w185:dbl, "Position.y"=w184:dbl)
                              }
                            }
                            n1011 = local read "Spot Storage 2"() -> (w171:T1[])
                            n1012 = local read "Numeric"() -> (w170:dbl)
                            n1013 = Index Array(array=w171, index=w170) -> (element=w157:T1)
                            n1014 = local read "Start at Which Frame?"() -> (w159:dbl)
                            n1015 = Bundle By Name(cluster=w157, "Position.x"=w155, "Position.y"=w154) -> (w156:T1)
                            n1016 = local read "How Many Frames?"() -> (w158:dbl)
                            n1017 = Subtract(x=w159, y=w153) -> (x-y=w168:dbl)
                            n1018 = local read "Sequence Storer"() -> (w169:T1[][])
                            n1019 = local read "Numeric"() -> (w164:dbl)
                            n1020 = Add(x=w168, y=w158) -> (x+y=w167:dbl)
                            n1021 = Subtract(x=w167, y=1) -> (x-y=w165:dbl)
                            n1022 = Replace Array Subset(array=w169, new element=w156, index (row)=w165, index (col)=w164) -> (w163:T1[][])
                            n1023 = Array Size(array=w163) -> (size(s)=w162:i32[])
                            n1024 = local write "Sequence Storer"(w163) -> ()
                            n1025 = Index Array(array=w162, index=0) -> (element=w160:i32)
                            n1026 = local write "Sequence Instances"(w160) -> ()
                          }
                        }
                        frame "Line" {
                          # "This is the automatic sequence generator which allows for the creation of the sequence. This calculates the LAST coordinates of each bubble first\nbefore going for the first few coordinates of the sequence."
                          n1027 = local read "How Many Frames?"() -> (w189:dbl)
                          n1028 = for {
                            N: w189 -> [_]
                            i -> [w197]
                            # "For why do we multiply?"
                            n1029 = local read "Spot Storage 2"() -> (w207:T1[])
                            n1030 = local read "Numeric"() -> (w194:dbl)
                            n1031 = local read "NewXYRates"() -> (w195:dbl[][])
                            n1032 = Index Array(array=w195, index (row)=w194, index (col)=1) -> (element=w190:dbl)
                            n1033 = Index Array(array=w195, index (row)=w194, index (col)=0) -> (element=w191:dbl)
                            n1034 = Index Array(array=w207, index=w194) -> (element=w205:T1)
                            n1035 = Unbundle By Name(w205) -> ("Position.x"=w212:dbl, "Position.y"=w210:dbl)
                            n1036 = Multiply(x=w191, y=w197) -> (x*y=w211:dbl)
                            n1037 = Multiply(x=w190, y=w197) -> (x*y=w206:dbl)
                            "probe" <- w206
                            n1038 = Subtract(x=w212, y=w211) -> (x-y=w209:dbl)
                            n1039 = Subtract(x=w210, y=w206) -> (x-y=w208:dbl)
                            n1040 = Bundle By Name(cluster=w205, "Position.x"=w209, "Position.y"=w208) -> (w200:T1)
                            n1041 = local read "Sequence Storer"() -> (w213:T1[][])
                            n1042 = local read "Numeric"() -> (w199:dbl)
                            n1043 = Add(x="Start at Which Frame?", y=w197) -> (x+y=w196:dbl)
                            n1044 = Replace Array Subset(array=w213, new element=w200, index (row)=w196, index (col)=w199) -> (w204:T1[][])
                            n1045 = Array Size(array=w204) -> (size(s)=w203:i32[])
                            n1046 = local write "Sequence Storer"(w204) -> ()
                            n1047 = Index Array(array=w203, index=0) -> (element=w201:i32)
                            n1048 = local write "Sequence Instances"(w201) -> ()
                          }
                        }
                      }
                    }
                    frame #1 {
                      w215 = FALSE
                      n1049 = Tick Count (ms)() -> (millisecond timer value=→"Stop":u32)
                      n1050 = local write "Play Pressed"(w215) -> ()
                      "Insert End" <- w215
                    }
                  }
                }
              }
              "Numeric" <- w142
            }
            frame #2 {
              n1051 = local write "Insert"(FALSE) -> ()
            }
          }
        }
      }
    }
    n1052 = And(x=w51, y=w55) -> (x .and. y?=w56:bool)
    n1053 = case shown="True" w56 {
      frame False {
      }
      frame True {
        n1054 = local read "# of Spots"() -> (w296:dbl)
        n1055 = for {
          N: w296 -> [_]
          i -> [w298]
          stop <- w297 stop-if-true
          n1056 = local read "Selection/Group"() -> (w300:T7[])
          n1057 = Index Array(array=w300, index=w298) -> (element=w299:T7)
          n1058 = Unbundle By Name(w299) -> ("Selected"=w297:bool)
          n1059 = case shown="True" w297 {
            tunnel: w298 -> [_ w302]
            frame False {
            }
            frame True {
              n1060 = local write "Current Spot #"(w302) -> ()
              "Induce check" <- TRUE
            }
          }
        }
      }
    }
    n1061 = local read "spots selected"() -> (w66:i32)
    n1062 = local read "spots selected 2"() -> (w67:i32)
    n1063 = local read "Prev Current Spot"() -> (w75:dbl)
    n1064 = local read "Current Spot #"() -> (w76:dbl)
    n1065 = Not Equal?(x=w76, y=w75) -> (x != y?=w74:bool)
    n1066 = Greater?(x=w67, y=w66) -> (0:w68:bool)
    n1067 = local read "Induce check"() -> (w57:bool)
    n1068 = Or(x=w74, y=w68) -> (x .or. y?=w59:bool)
    n1069 = Or(x=w59, y=w57) -> (x .or. y?=w58:bool)
    n1070 = case shown="True" w58 {
      frame False {
      }
      frame True {
        n1071 = stacked-sequence {
          frame #0 {
            # "A small 100 ms delay is given to provide enough time for the data to be processed properly."
            n1072 = local read "Null array"() -> (w308:dbl[])
            n1073 = local write "What to Check"(w308) -> ()
            n1074 = local write "ID"(w308) -> ()
            n1075 = local read "Current Spot #"() -> (w310:dbl)
            n1076 = local write "Potential Collisions"(0) -> ()
            n1077 = local read "Spot Checker"() -> (w309:T1[])
            n1078 = Index Array(array=w309, index=w310) -> (element=w311:T1)
            n1079 = Wait (ms)(milliseconds to wait=10) -> ()  [unwired: 1 out]
            n1080 = Unbundle By Name(w311) -> ("Position.x"=w305:dbl, "Position.y"=w306:dbl)
            n1081 = local write "Orig Y SC"(w306) -> ()
            n1082 = local write "Orig X SC"(w305) -> ()
            n1083 = local write "Induce check"(FALSE) -> ()
          }
          frame #1 {
            n1084 = local read "# of Spots"() -> (w312:dbl)
            n1085 = for {
              N: w312 -> [_]
              tunnel: w312 -> [w317]
              i -> [w313]
              n1086 = local read "Selection/Group"() -> (w316:T7[])
              n1087 = Index Array(array=w316, index=w313) -> (element=w315:T7)
              n1088 = Unbundle By Name(w315) -> ("Selected"=w314:bool)
              n1089 = case shown="True" w314 {
                tunnel: w317 -> [_ w319]
                tunnel: w313 -> [_ w318]
                frame False {
                }
                frame True {
                  n1090 = for {
                    N: w319 -> [_]
                    tunnel: w318 -> [w320]
                    i -> [w321]
                    # "If the bubble is not selected, find difference of bubble to bubble\nbeing checked"
                    n1091 = local read "Selection/Group"() -> (w325:T7[])
                    n1092 = Index Array(array=w325, index=w321) -> (element=w324:T7)
                    n1093 = Unbundle By Name(w324) -> ("Selected"=w322:bool)
                    n1094 = Not(x=w322) -> (.not. x?=w323:bool)
                    n1095 = case shown="True" w323 {
                      tunnel: w321 -> [_ w329]
                      tunnel: w320 -> [_ w328]
                      tunnel: w320 -> [_ w327]
                      frame False {
                      }
                      frame True {
                        n1096 = local read "Spot Checker"() -> (w346:T1[])
                        n1097 = Index Array(array=w346, index=w329) -> (element=w347:T1)
                        n1098 = Index Array(array=w346, index=w328) -> (element=w345:T1)
                        n1099 = Unbundle By Name(w345) -> ("Position.x"=w342:dbl, "Position.y"=w338:dbl)
                        n1100 = Unbundle By Name(w347) -> ("Position.x"=w339:dbl, "Position.y"=w335:dbl)
                        n1101 = local read "Area+ Buffer"() -> (w326:dbl)
                        n1102 = Subtract(x=w342, y=w326) -> (x-y=w343:dbl)
                        n1103 = Greater Or Equal?(x=w339, y=w343) -> (x >= y?=w344:bool)
                        n1104 = Add(x=w338, y=w326) -> (x+y=w337:dbl)
                        n1105 = Subtract(x=w338, y=w326) -> (x-y=w336:dbl)
                        n1106 = Add(x=w342, y=w326) -> (x+y=w340:dbl)
                        n1107 = Less Or Equal?(x=w335, y=w337) -> (x <= y?=w334:bool)
                        n1108 = Greater Or Equal?(x=w335, y=w336) -> (x >= y?=w333:bool)
                        n1109 = Less Or Equal?(x=w339, y=w340) -> (x <= y?=w341:bool)
                        n1110 = And(x=w344, y=w341) -> (x .and. y?=w331:bool)
                        n1111 = And(x=w334, y=w333) -> (x .and. y?=w332:bool)
                        n1112 = And(x=w331, y=w332) -> (x .and. y?=w330:bool)
                        n1113 = case shown="True" w330 {
                          tunnel: w329 -> [_ _]
                          tunnel: w329 -> [_ w349]
                          tunnel: w327 -> [_ w348]
                          frame False {
                          }
                          frame True {
                            n1114 = stacked-sequence {
                              tunnel: w349 -> [w350 _]
                              tunnel: w348 -> [w351 _]
                              frame #0 {
                                n1115 = local read "Potential Collisions"() -> (w354:dbl)
                                n1116 = local read "What to Check"() -> (w355:dbl[])
                                n1117 = Insert Into Array(array=w355, index=w354, new element=w350) -> (w356:dbl[])
                                n1118 = local read "ID"() -> (w353:dbl[])
                                n1119 = local write "What to Check"(w356) -> ()
                                n1120 = Insert Into Array(array=w353, index=w354, new element=w351) -> (w352:dbl[])
                                n1121 = local write "ID"(w352) -> ()
                              }
                              frame #1 {
                                n1122 = local read "Potential Collisions"() -> (w359:dbl)
                                n1123 = Add(x=w359, y=1) -> (x+y=w357:dbl)
                                n1124 = local write "Potential Collisions"(w357) -> ()
                              }
                            }
                          }
                        }
                      }
                    }
                  }
                }
              }
            }
          }
          frame #2 {
            n1125 = local read "Current Spot #"() -> (w360:dbl)
            n1126 = local write "Prev Current Spot"(w360) -> ()
          }
        }
      }
    }
    n1127 = local read "Buffer Zone"() -> (w72:dbl)
    n1128 = Multiply(x=w72, y=2) -> (x*y=w73:dbl)
    n1129 = Add(x="Area to check", y=w73) -> (x+y=→"Area+ Buffer":dbl)
    n1130 = feedback #11() -> (w45:dbl)  [unwired: 1 in]
    n1131 = Equal?(x=w45, y=10000) -> (x = y?=w46:bool)
    n1132 = call "Elapsed Time"("Reset"=w46) -> ("Elapsed Time (s)"=w44:dbl, "Time has Elapsed"=w49:bool)  [unwired: 11 in, 6 out]
    "Elapsed Time" <- w44
    n1133 = feedback-in #11(w44) -> ()
    n1134 = And(x="On", y=w49) -> (x .and. y?=w50:bool)
    n1135 = case shown="True" w50 {
      frame False {
      }
      frame True {
        n1136 = local read "Position"() -> (w295:cluster{"x":dbl, "y":dbl, "z":dbl})
        n1137 = Unbundle By Name(w295) -> ("x"=→"X Pos every 10 sec":dbl)
      }
    }
    n1138 = case shown="True" "OK Button" {
      frame False {
      }
      frame True {
        n1139 = script code="clear all;\nclc;\n\ng = gigecam('169.254.154.83');\n\ng.PixelFormat= 'BayerGR8'\n\nimg = snapshot(g);\n\nimshow(img);"() -> ()  [unwired: 1 in, 1 out]
      }
    }
    n1140 = case shown="True" "O Button" {
      frame False {
      }
      frame True {
        n1141 = script code="%\n    rslt = Hough1_data(img);\n\n    % Frame translation\n    %- omit this as of now \n    \n    % Control method\n    increment = 10; %assuming the diamiter of the agent around 20 pic \n    \n    %- NewLoc = [x,y] whose unit is px\n    %- update new location based on current location obtained by the camera\n    NewLoc(1)= rslt(1);\n    NewLoc(2)= rslt(2);\n    \n    \n    % Update microrobot location with NewLoc\n    % the single robot would move to oblique downword\n    \n    % wait seconds"() -> ("NewLoc"=w291:dbl[])  [unwired: 1 in, 1 out]
        n1142 = Index Array(array=w291, index=1) -> (element=→"Y":dbl)
        n1143 = Index Array(array=w291, index=0) -> (element=→"X":dbl)
      }
    }
  }
  n1144 = flat-sequence {
    tunnel: w6 -> [w1826]
    tunnel: w5 -> [w1825]
    tunnel: [w1824] -> w3
    frame #0 {
      n1145 = disable-structure shown="\"White Image (stub)\"" {
        disable-tunnel: w1826 -> [_ _ _ _ _ _]
        disable-tunnel: w1825 -> [_ _ w1884 _ _ _]
        disable-tunnel: [_ _ w1883 _ _ _] -> w1824
        frame condition #0 {
          w1828 = u32 10 ("Number of buffers")
          (unwired) FALSE ("background subtraction")
          # "This subdiagram uses the IMAQ drivers, with a pre-allocated ringbuffer for images.  This is the code I use with my Mikrotron MC1362-CL"
          n1146 = call <vilib>:"IMAQ Init.vi"("Interface Name"="img0") -> ("IMAQ Session Out"=w1835:refnum<k11>)  [unwired: 9 in, 1 out]
          n1147 = call <vilib>:"IMAQ Configure List.vi"("Region of interest"="Global ROI (requires restart)", "Number of buffers"=w1828, "Continuous?"=enum16{"One-Shot", "Continuous"}."Continuous", "IMAQ Session In"=w1835) -> ("error out"=w1829:errorcluster, "IMAQ Session Out"=w1831:refnum<k11>)  [unwired: 6 in]
          n1148 = for {
            N: w1828 -> [_]
            tunnel: 0 ("Channel") -> [w1848]
            shift-right: [w1851] -> w1833
            shift-left: w1829 -> [w1847]
            shift-right: [w1850] -> w1832
            shift-left: w1831 -> [w1849]
            i -> [w1846]
            n1149 = Format Into String(format string="mikrotronbuffer%04d", w1846) -> (resulting string=w1844:string)  [unwired: 2 in, 1 out]
            n1150 = call "IMAQ Create"("Image Name"=w1844) -> ("New Image"=w1843:T8)  [unwired: 4 in, 1 out]
            n1151 = call <vilib>:"IMAQ Configure Buffer.vi"("Channel"=w1848, "error in (no error)"=w1847, "Buffer Number"=w1846, "Image In"=w1843, "IMAQ Session In"=w1849) -> ("error out"=w1851:errorcluster, "IMAQ Session Out"=w1850:refnum<k11>)  [unwired: 5 in]
          }
          n1152 = call <vilib>:"IMAQ Start.vi"("error in (no error)"=w1833, "IMAQ Session In"=w1832) -> ("error out"=w1839:errorcluster, "IMAQ Session Out"=w1840:refnum<k11>)  [unwired: 8 in]
          n1153 = call "IMAQ Create"("Image Name"="Red Tweezers live image") -> ("New Image"=w1841:T8)  [unwired: 3 in, 2 out]
          n1154 = while {
            tunnel: w1840 -> [w1859]
            tunnel: w1839 -> [w1858]
            tunnel: w1841 -> [_]
            tunnel: [w1860] -> w1837
            tunnel: [w1853] -> w1838
            i -> [w1855]
            stop <- w1861 stop-if-true
            n1155 = local read "stop"() -> (w1861:bool)
            n1156 = call <vilib>:"IMAQ Extract Buffer.vi"("error in (no error)"=w1858, "Buffer to extract"=w1855, "IMAQ Session In"=w1859) -> ("error out"=w1853:errorcluster, "Image Out"=w1852:T8, "IMAQ Session Out"=w1860:refnum<k11>)  [unwired: 3 in, 3 out]
            n1157 = call "imageQ_camera_hook.vi"("Image"=w1852) -> ()  [unwired: 11 in]
            n1158 = feedback #12() -> (w1856:T23)  [unwired: 1 in]
            n1159 = call "Smoothed Frame Rate.vi"("Feedback In"=w1856) -> ("Feedback Out"=w1857:T23, "Frame Rate"=w1854:dbl)  [unwired: 1 in, 4 out]
            n1160 = feedback-in #12(w1857) -> ()
            n1161 = global write "red_tweezers_globals_INTERNAL_VOLATILE.vi" "Video Frame Rate"(w1854) -> ()
          }
          n1162 = call <vilib>:"IMAQ Close.vi"("error in (no error)"=w1838, "IMAQ Session In"=w1837) -> ()  [unwired: 9 in, 1 out]
        }
        frame condition #1 {
          (unwired) FALSE ("background subtraction")
          # "This subdiagram acquires using the IMAQdx drivers.  This covers most FireWire and GigE cameras (at least the ones supporting the IIDC or GenICam standards)."
          n1163 = call <vilib>:"IMAQdx Open Camera.vi"("Session In"=T6 "dalsaGenie") -> ("error out"=w1864:errorcluster, "Session Out"=w1863:T6)  [unwired: 9 in]
          n1164 = call <vilib>:"IMAQdx Configure Grab.vi"("error in"=w1864, "Session In"=w1863) -> ("error out"=w1865:errorcluster, "Session Out"=w1866:T6)  [unwired: 8 in]
          n1165 = call "IMAQ Create"("Image Name"="Red Tweezers live image") -> ("New Image"=w1869:T8)  [unwired: 3 in, 2 out]
          n1166 = while {
            tunnel: w1866 -> [w1878]
            tunnel: w1865 -> [w1877]
            tunnel: w1869 -> [w1871]
            tunnel: [w1879] -> w1867
            tunnel: [w1873] -> w1868
            stop <- w1880 stop-if-true
            n1167 = local read "stop"() -> (w1880:bool)
            n1168 = call <vilib>:"IMAQdx Grab.vi"("error in"=w1877, "Image In"=w1871, "Session In"=w1878) -> ("error out"=w1873:errorcluster, "Image Out"=w1872:T8, "Session Out"=w1879:T6)  [unwired: 5 in, 1 out]
            n1169 = call "imageQ_camera_hook.vi"("Image"=w1872) -> ()  [unwired: 11 in]
            n1170 = feedback #13() -> (w1875:T23)  [unwired: 1 in]
            n1171 = call "Smoothed Frame Rate.vi"("Feedback In"=w1875) -> ("Feedback Out"=w1876:T23, "Frame Rate"=w1874:dbl)  [unwired: 1 in, 4 out]
            n1172 = feedback-in #13(w1876) -> ()
            n1173 = global write "red_tweezers_globals_INTERNAL_VOLATILE.vi" "Video Frame Rate"(w1874) -> ()
          }
          n1174 = call <vilib>:"IMAQdx Close Camera.vi"("error in"=w1868, "Session In"=w1867) -> ()  [unwired: 9 in, 1 out]
        }
        frame condition #2 {
          # "This subdiagram acquires using the IMAQdx drivers.  This covers most FireWire and GigE cameras (at least the ones supporting the IIDC or GenICam standards)."
          n1175 = call <vilib>:"IMAQdx Open Camera.vi"("Session In"="Camera") -> ("error out"=w1892:errorcluster, "Session Out"=w1891:T6)  [unwired: 9 in]
          n1176 = call <vilib>:"IMAQdx Configure Grab.vi"("error in"=w1892, "Session In"=w1891) -> ("error out"=w1888:errorcluster, "Session Out"=w1889:T6)  [unwired: 8 in]
          n1177 = call "IMAQ Create"("Image Name"="Red Tweezers live image") -> ("New Image"=w1886:T8)  [unwired: 3 in, 2 out]
          n1178 = call "IMAQdx_get_ROI.vi"("Session In"=w1889) -> ("ROI"=w1885:u32[], "Session Out"=w1887:T6)  [unwired: 8 in]
          n1179 = while {
            shift-right: [w1901] -> w1881
            shift-left: w1888 -> [w1902]
            shift-right: [w1898] -> w1882
            shift-left: w1887 -> [w1899]
            tunnel: w1886 -> [w1897]
            tunnel: w1885 -> [w1896]
            tunnel: w1884 -> [w1895]
            tunnel: [w1894] -> w1883
            stop <- w1908 stop-if-true
            n1180 = event shown="[0] Timeout" {
              selector: _ -> [_ _ _]
              dyn-events: _ -> [_ _ _]
              timeout: 0 -> [_ _ _]
              tunnel: w1902 -> [w1915 w1922 w1937]
              tunnel: [w1914 w1922 w1937] -> w1901
              tunnel: w1899 -> [w1913 w1923 w1938]
              tunnel: [w1912 w1923 w1938] -> w1898
              tunnel: w1897 -> [w1911 _ _]
              tunnel: w1896 -> [w1910 _ _]
              tunnel: w1895 -> [_ w1921 w1936]
              event Timeout {
                w1909 = 0  # timeout in ms
                # "Use a timeout of a few hundred ms if you want to acquire just fast enough to update the image- or a timeout of zero to run the camera at full speed."
                # "This VI sends the image to the loop above for display.\nIt's better to do this than to display here, because it separates the camera loop from the front panel a bit, and increases speed without sacrificing responsiveness of the UI.  Of course, using the event structure removes some of those benefits- but it is possible to write a high-performance camera loop with fast particle tracking, and still use this mechanism to display images without slowing down acquisition."
                # "If we're not dealing with other events, acquire from the camera."
                n1181 = event-data() -> ("Time"=w1920:u32)  [unwired: 1 in]
                n1182 = call <vilib>:"IMAQdx Grab.vi"("error in"=w1915, "Image In"=w1911, "Session In"=w1913) -> ("error out"=w1914:errorcluster, "Image Out"=w1917:T8, "Session Out"=w1912:T6)  [unwired: 5 in, 1 out]
                n1183 = call "IMAQ Clear Overlay"("Image"=w1917) -> ("Image Out"=w1916:T8)  [unwired: 9 in, 1 out]
                n1184 = Multiply(x=w1920, y=u32 1000) -> (x*y=w1918:u32)
                n1185 = call "imageQ_camera_hook.vi"("timeout in ms (0=don't wait if there are no requests)"=w1909, "Timestamp/us"=w1918, "ROI"=w1910, "Image"=w1916) -> ()  [unwired: 8 in]
              }
              event "Draw ROI", "Zoom": Value Change {
                # "This changes the current mouse mode on the image, allowing zooming/drawing of ROI (which can be useful if you want to window down a camera for particle tracking)."
                n1186 = event-data() -> ("CtlRef"=w1928:refnum<vi>)  [unwired: 1 in]
                n1187 = control-ref of="Draw ROI"() -> (w1929:refnum<vi>)
                n1188 = Equal?(x=w1929, y=w1928) -> (x = y?=w1927:bool)
                n1189 = case shown="True" w1927 {
                  tunnel: [w1932 w1935] -> w1926
                  tunnel: [TRUE ("stop") FALSE ("stop")] -> w1924
                  tunnel: [FALSE ("Update Indicators?") TRUE ("Update Indicators?")] -> w1925
                  frame False {
                    w1932 = u32 8 items=["Zoom Tool"=8, "Selection Tool"=0, "Pan Tool"=9, "Point Tool"=1, "Line Tool"=2, "Rectangle Tool"=3, "Rotated Rectangle Tool"=12, "Polyline Tool"=10, "Polygon Tool"=5, "Freehand Tool"=11, "Closed Freehand Tool"=6, "Ellipse Tool"=4, "Annulus Tool"=7] ("Current ROI Tool")
                  }
                  frame True {
                    w1935 = u32 3 items=["Zoom Tool"=8, "Selection Tool"=0, "Pan Tool"=9, "Point Tool"=1, "Line Tool"=2, "Rectangle Tool"=3, "Rotated Rectangle Tool"=12, "Polyline Tool"=10, "Polygon Tool"=5, "Freehand Tool"=11, "Closed Freehand Tool"=6, "Ellipse Tool"=4, "Annulus Tool"=7] ("Current ROI Tool")
                  }
                }
                n1190 = local write "Draw ROI"(w1925) -> ()
                n1191 = local write "Zoom"(w1924) -> ()
                n1192 = property on="Property Node" class="ImageControl"(reference=w1921, "Current ROI Tool"=w1926) -> ()  [unwired: 1 in, 2 out]
              }
              event "Zoom to Fit": Value Change {
                # "The various ROI tools are hidden, so the image control resizes nicely as the Red Tweezers window is resized.  The zoom to fit button/mouse mode buttons return some of this functionality."
                n1193 = event-data() -> ("NewVal"=w1939:bool)  [unwired: 1 in]
                n1194 = property on="Property Node" class="ImageControl"(reference=w1936, "Zoom to Fit Mode"=w1939) -> ()  [unwired: 1 in, 2 out]
              }
            }
            n1195 = feedback #14() -> (w1907:T23)  [unwired: 1 in]
            n1196 = call "Smoothed Frame Rate.vi"("Feedback In"=w1907, "Alpha"=0.05) -> ("Feedback Out"=w1906:T23, "Frame Rate"=w1903:dbl)  [unwired: 4 out]
            n1197 = feedback-in #14(w1906) -> ()
            n1198 = global write "red_tweezers_globals_INTERNAL_VOLATILE.vi" "Video Frame Rate"(w1903) -> ()
            n1199 = local read "stop"() -> (w1904:bool)
            n1200 = Unbundle By Name(w1901) -> ("status"=w1894:bool)
            n1201 = Or(x=w1894, y=w1904) -> (x .or. y?=w1908:bool)
          }
          n1202 = call <vilib>:"IMAQdx Close Camera.vi"("error in"=w1881, "Session In"=w1882) -> ()  [unwired: 9 in, 1 out]
        }
        frame condition #3 (active) {
          w1941 = 0 ("element")
          w1943 = 1920 ("dimension size")
          w1942 = 1080 ("dimension size")
          w1944 = T26 0 items=["Grayscale (U8)", "Grayscale (I16)", "Grayscale (SGL)", "Complex (CSG)", "RGB (U32)", "HSL (U32)", "RGB (U64)", "Grayscale (U16)"] ("Image Type")
          (unwired) FALSE ("background subtraction")
          # "This subdiagram generates a blank white image- useful if you don't have a camera"
          n1203 = Build Array(w1941, w1941, w1943, w1942) -> (w1940:i32[])
          n1204 = Initialize Array(u8 255 ("element"), w1942, w1943) -> (w1945:u8[][])
          n1205 = global write "red_tweezers_globals_INTERNAL.vi" "Global ROI"(w1940) -> ()
          n1206 = call "IMAQ Create"("Image Name"="red tweezers camera stub", "Image Type"=w1944) -> ("New Image"=w1946:T8)  [unwired: 2 in, 2 out]
          n1207 = call "IMAQ ArrayToImage"("Image Pixels (U8)"=w1945, "Image"=w1946) -> ("Image Out"=w1949:T8)  [unwired: 8 in, 1 out]
          n1208 = call "IMAQ Create"("Image Name"="Red Tweezers live image") -> ("New Image"=w1950:T8)  [unwired: 3 in, 2 out]
          n1209 = while {
            tunnel: w1949 -> [w1953]
            tunnel: w1950 -> [_]
            stop <- w1957 stop-if-true
            n1210 = local read "stop"() -> (w1957:bool)
            n1211 = Wait Until Next ms Multiple(millisecond multiple=u32 20) -> ()  [unwired: 1 out]
            n1212 = call "imageQ_camera_hook.vi"("Image"=w1953) -> ()  [unwired: 11 in]
            n1213 = feedback #15() -> (w1955:T23)  [unwired: 1 in]
            n1214 = call "Smoothed Frame Rate.vi"("Feedback In"=w1955) -> ("Feedback Out"=w1956:T23, "Frame Rate"=w1954:dbl)  [unwired: 1 in, 4 out]
            n1215 = feedback-in #15(w1956) -> ()
            n1216 = global write "red_tweezers_globals_INTERNAL_VOLATILE.vi" "Video Frame Rate"(w1954) -> ()
          }
        }
        frame condition #4 {
          # "Use this subdiagram if you have an external camera VI which writes to the image queue (using imageQ_camera_hook.vi)"
        }
        frame condition #5 {
          w1958 = path "C:/Users/Tweezer Cube/Desktop/red_tweezers_1_4_rc0/camera_for_rt136.llb/Particle Tracking.vi"  # Path to camera VI
          # "Use this subdiagram if you have an external camera VI which writes to the image queue (using imageQ_camera_hook.vi).  This is the slightly more sophisticated version, which checks that said external VI is running, and runs it if not."
          n1217 = Open VI Reference(vi path=w1958) -> (vi reference=w1959:refnum<vi>, error out=w1961:errorcluster)  [unwired: 5 in]
          n1218 = property class="VI"(reference=w1959) -> ("Path"=w1960:path)  [unwired: 1 in, 2 out]
          n1219 = global write "red_tweezers_globals_INTERNAL_VOLATILE.vi" "Current Camera VI"(w1960) -> ()
          n1220 = property class="VI"(reference=w1959, error in=w1961) -> (reference out=w1966:refnum<vi>, error out=w1965:errorcluster, "Exec.State"=w1963:T25)
          n1221 = Equal?(x=w1963, y=T25."Idle") -> (x = y?=w1967:bool)
          n1222 = case shown="True" w1967 {
            tunnel: w1966 -> [w1971 w1980]
            tunnel: w1965 -> [w1970 w1977]
            tunnel: [w1969 w1976] -> w1962
            tunnel: w1963 -> [w1973 _]
            frame False {
              n1223 = Close Reference(reference=w1971, error in (no error)=w1970) -> (error out=w1969:errorcluster)
              n1224 = Equal?(x=w1973, y=T25."Bad") -> (x = y?=w1972:bool)
              n1225 = case shown="False" w1972 {
                frame False {
                }
                frame True {
                  n1226 = One Button Dialog(message="The external camera VI is not running and cannot be started- it's probably broken or missing.  Check the static/dynamically loaded VI reference in the bottom loop on the block diagram.") -> ()  [unwired: 1 in, 1 out]
                }
              }
            }
            frame True {
              n1227 = invoke class="VI" method="Run VI"(reference=w1980, error in=w1977, "Wait until done"=FALSE ("Wait Until Done"), "Auto Dispose Ref"=TRUE ("Auto Dispose Reference")) -> (error out=w1976:errorcluster)  [unwired: 1 in, 4 out]
            }
          }
          n1228 = call <vilib>:"Simple Error Handler.vi"("error source (\" \")"="External camera VI (see the bottom loop in the block diagram)" ("error source (\" \")"), "error in (no error)"=w1962) -> ()  [unwired: 3 in, 5 out]
        }
      }
    }
  }
  n1229 = while {
    tunnel: w9 -> [w1998]
    shift-right: [w1997] -> w8
    shift-left: w10 -> [w1999]
    shift-right: [w1994] -> _
    shift-left: _ -> [w1987]
    shift-right: [w1993] -> _
    shift-left: _ -> [w1991]
    shift-right: [w1992] -> _
    shift-left: FALSE ("Saving") -> [w1988]
    stop <- w1996 stop-if-true
    w1985 = u32 50 ("millisecond multiple")
    # "Start/stop saving data, if necessary"
    n1230 = Divide(x=u32 1000, y=w1985) -> (x/y=w1983:dbl)
    n1231 = Wait Until Next ms Multiple(millisecond multiple=w1985) -> ()  [unwired: 1 out]
    n1232 = call "imageQ_dequeue.vi"("timeout in ms (-1)"=2000, "Return queue"=w1999, "Image Dst"=w1998) -> ("Timestamp/us"=w1989:u64, "Return queue out"=w1997:refnum<queue>, "Image Dst Out"=w2000:T8, "timed out?"=w2003:bool, "ROI"=w1982:u64[])  [unwired: 4 in]
    n1233 = Not(x=w2003) -> (.not. x?=w2001:bool)
    n1234 = case shown="True" w2001 {
      tunnel: w2000 -> [_ w2037]
      tunnel: w1991 -> [w2030 w2040]
      tunnel: w1988 -> [_ w2034]
      tunnel: [w2030 w2035] -> w1990
      tunnel: w1989 -> [_ w2038]
      tunnel: w1987 -> [w2031 w2039]
      tunnel: [w2031 w2036] -> w1986
      tunnel: w1982 -> [_ w2033]
      frame False {
      }
      frame True {
        n1235 = global read "red_tweezers_globals_INTERNAL.vi" "Image Overlay (extras from control loop)"() -> (w2048:T16[])
        n1236 = case shown="True" w2034 {
          tunnel: w2040 -> [w2049 w2051]
          tunnel: w2039 -> [w2050 w2057]
          tunnel: w2038 -> [_ w2056]
          tunnel: w2037 -> [_ w2055]
          tunnel: [w2050 w2054] -> w2036
          tunnel: [w2049 w2053] -> w2035
          frame False {
          }
          frame True {
            n1237 = call "save_data_save.vi"("Image"=w2055, "Timestamp"=w2056, "Avi Refnum"=w2051, "Data refnum"=w2057) -> ("error out"=w2052:errorcluster, "Avi Refnum (duplicate)"=w2053:T27, "Data refnum (duplicate)"=w2054:refnum<file>)  [unwired: 5 in]
            n1238 = case shown="Error" w2052 {
              selector: w2052 -> [_ w2059]
              frame No Error {
              }
              frame Error {
                n1239 = call <vilib>:"Clear Errors.vi"("error in (no error)"=w2059) -> ()  [unwired: 5 in, 2 out]
                n1240 = local write "Save Video"(FALSE ("Save")) -> ()
              }
            }
          }
        }
        n1241 = global write "red_tweezers_globals_INTERNAL.vi" "Global ROI"(w2033) -> ()
        n1242 = global read "red_tweezers_globals_INTERNAL_VOLATILE.vi" "Tracked Spot Positions (3D)"() -> (w2041:cluster{"x":dbl, "y":dbl, "Z":dbl}[])
        n1243 = global read "red_tweezers_globals.vi" "Selection/Group"() -> (w2047:T7[])
        n1244 = global read "red_tweezers_globals.vi" "Spots"() -> (w2046:T1[])
        n1245 = call "overlay_positions.vi"("Positions"=w2041, "Image"=w2037) -> ("Image 2"=w2043:T8)  [unwired: 9 in]
        n1246 = call "render_overlay_elements.vi"("Image Overlay (extras from control loop)"=w2048, "Image"=w2043) -> ("Image Out"=w2045:T8)  [unwired: 5 in]
        n1247 = call "grid_and_guides.vi"("Operation"=T11."Render on image", "Image"=w2045) -> ("Image Out"=w2032:T8)  [unwired: 9 in]
        n1248 = call "overlay_spots_on_image.vi"("Selection and Groups"=w2047, "Spots"=w2046, "image"=w2032) -> ("Image"=→"Image":T8)  [unwired: 3 in, 1 out]
      }
    }
    n1249 = global read "red_tweezers_globals_INTERNAL_VOLATILE.vi" "Video Frame Rate"() -> (→"Video Frame Rate":dbl)
    n1250 = case shown="True" "Save Video" {
      tunnel: [w2006 w2021] -> w1994
      tunnel: [w2005 w2015] -> w1993
      tunnel: [FALSE ("Saving") w2020] -> w1992
      tunnel: w1988 -> [w2009 w2019]
      tunnel: w1990 -> [w2007 w2018]
      tunnel: w1986 -> [w2008 w2017]
      tunnel: w1983 -> [_ w2016]
      frame False {
        n1251 = case shown="True" w2009 {
          tunnel: w2008 -> [w2011 w2014]
          tunnel: w2007 -> [w2010 w2013]
          tunnel: [w2011 _] -> w2006
          tunnel: [w2010 _] -> w2005
          frame False {
          }
          frame True {
            n1252 = local write "Save Video"(FALSE ("Save")) -> ()
            n1253 = call "save_data_stop.vi"("Avi Refnum"=w2013, "Data refnum"=w2014) -> ()  [unwired: 10 in]
          }
        }
      }
      frame True {
        n1254 = case shown="False" w2019 {
          selector: w2019 -> [_ w2029]
          tunnel: [w2026 w2027] -> w2021
          tunnel: [w2025 w2028] -> w2015
          tunnel: [w2022 w2029] -> w2020
          tunnel: w2018 -> [_ w2028]
          tunnel: w2017 -> [_ w2027]
          tunnel: w2016 -> [w2024 _]
          frame False {
            n1255 = call "save_data_start.vi"("Save Video"=TRUE, "Frames Per Second"=w2024) -> ("Saving"=w2022:bool, "Avi Refnum"=w2025:T27, "Data Refnum"=w2026:refnum<file>)  [unwired: 3 in]
            n1256 = local write "Save Video"(w2022) -> ()
          }
          frame True {
          }
        }
      }
    }
    n1257 = local read "stop"() -> (w1996:bool)
  }
  n1258 = Release Queue(queue=w8) -> ()  [unwired: 2 in, 3 out]
  n1259 = case shown="True" w3 {
    frame False {
    }
    frame True {
      n1260 = One Button Dialog(message="Warning: there was a camera error.  You may need to restart Red Tweezers.") -> ()  [unwired: 1 in, 1 out]
    }
  }
  n1261 = flat-sequence {
    tunnel: w18 -> [w2065]
    tunnel: w17 -> [_]
    frame #0 {
      # "This autosaves when we stop.  The sequence structures are necessary so that:\n1. loading settings doesn't stop the VI\n2. plugins are still open (and hence saved) when we save settings"
      n1262 = local read "Plugins"() -> (w2068:T3)
      n1263 = global read "red_tweezers_globals_INTERNAL_VOLATILE.vi" "Current Settings File"() -> (w2062:path)
      n1264 = global read "red_tweezers_globals_INTERNAL_VOLATILE.vi" "Save Settings On Exit"() -> (w2061:bool)
      n1265 = flat-sequence {
        tunnel: w2065 -> [w2071]
        tunnel: [w2071] -> w2064
        frame #0 {
          n1266 = local write "stop"(FALSE ("STOP")) -> ()
        }
      }
      n1267 = case shown="True" w2061 {
        tunnel: w2062 -> [_ w2076]
        tunnel: w2064 -> [w2073 w2074]
        tunnel: [w2073 w2074] -> w2063
        frame False {
        }
        frame True {
          n1268 = Path To String(path=w2076) -> (string=w2075:string)
          n1269 = call "settings_save_to_file.vi"("XML File Path"=w2076) -> ()  [unwired: 11 in]
          n1270 = call "settings_filename_to_registry.vi"("Last Used Settings File"=w2075) -> ()  [unwired: 11 in]
        }
      }
      n1271 = flat-sequence {
        tunnel: w2063 -> [w2069]
        tunnel: [w2069] -> _
        frame #0 {
          n1272 = local write "stop"(TRUE ("STOP")) -> ()
        }
      }
      n1273 = control-ref of="Plugin Pnl"() -> (w2066:refnum<vi>)
      n1274 = control-ref of="Plugin:"() -> (w2067:refnum<vi>)
      n1275 = call "plugins_unload.vi"("error in (no error)"=w2063, "Plugins"=w2068, "Sub Panel"=w2066, "Plugin Chooser"=w2067) -> ()  [unwired: 2 in, 2 out]
    }
  }
